vi "FPGA Beam Scanning V1.vi"(1 "Detectors":T1, 2 "Image Acquisition Parameters":T2={"Scan Type"=enum."Sample Scanning", "Scan Mode"=enum."XY", "Fast Axis Frequency (Hz)"=100.0, "Image Format"=128, "Line Accumulations"=1, "Frames Per Capture"=1, "Frames Accumulations"=1, "Image Dimension (um)"=[], "Number of Z Steps"=1, "Z Steps Size (um)"=1.0, "Pixel Size (nm)"=[]} {"Z Steps Size (um)" min=0.0; "Number of Z Steps" min=1; "Frames Accumulations" min=1; "Frames Per Capture" min=1; "Line Accumulations" min=1; "Image Format" items=["64 x 64"=64, "128 x 128"=128, "256 x 256"=256, "512 x 512"=512, "1024 x 1024"=1024, "2048 x 2048"=2048]}) -> ()   [LabVIEW 2014]
uses:
  Type Defs/Image Acquisition Parameters.ctl
  Detectors.ctl
  <vilib>/vision/Image Controls.llb/IMAQ Image.ctl
  <vilib>/FPGAPlugInAG/PCIe-7852R/niLvFpga_Open_PCIe-7852R.vi
  <vilib>/Utility/error.llb/Error Cluster From Error Code.vi
  <vilib>/rvi/errors/niLvFpgaAdjustHostInterfaceError.vi
  <vilib>/rvi/interface/common/niFpgaWaitOnOcc.vi
  <vilib>/FPGAPlugInAG/PCIe-7852R/niLvFpga_Run_PCIe-7852R.vi
  <vilib>/FPGAPlugInAG/PCIe-7852R/niLvFpga_Close_PCIe-7852R.vi
  <vilib>/rvi/interface/nirviOpenFPGA/nirviOpenFPGA.xnode
  FPGA Bitfiles/MainSTEDFPGAProj_FPGATarget2_BeamScanningCamb_cWDGwb0YZ5k.lvbitx
  FPGA Target VIs/FPGA-7852R/Beam Scanning Cambridge V1.vi
  <vilib>/rvi/interface/nirviReadWriteControl/nirviReadWriteControl.xnode
  <vilib>/rvi/interface/nirviMethod/nirviMethod.xnode
  <vilib>/rvi/interface/nirviCloseFPGA/nirviCloseFPGA.xnode
  <vilib>/rvi/errors/niLvFpgaMergeErrorWithErrorCode.vi
  <vilib>/vision/NI_Vision_Development_Module.lvlib
  NiFpgaLv.dll
  <vilib>/FPGAPlugInAG/PCIe-7852R/niLvFpga_ReadFifo_PCIe-7852R.vi
  <vilib>/FPGAPlugInAG/PCIe-7852R/niLvFpga_ConfigureFifo_PCIe-7852R.vi
  <vilib>/FPGAPlugInAG/PCIe-7852R/niLvFpga_StartFifo_PCIe-7852R.vi
panel:
  # "XY"
  # "Z"
  # "Length"
  # "Height"
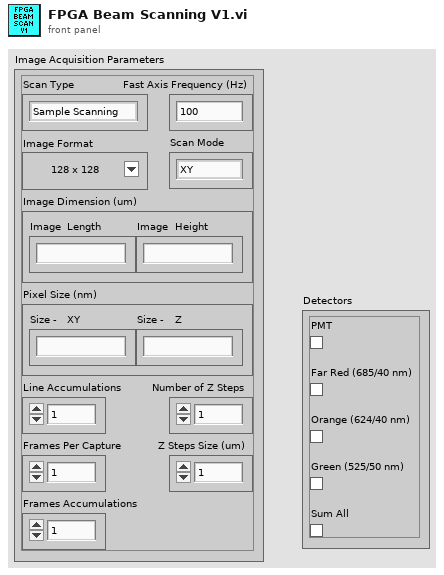
[diagram p1: front panel]
types:
  T1 = typedef "Detectors.ctl" = cluster{"PMT":bool, "Far Red (685/40 nm)":bool, "Orange (624/40 nm)":bool, "Green (525/50 nm)":bool, "Sum All":bool}
  T2 = typedef "Image Acquisition Parameters.ctl" = cluster{"Scan Type":enum16{"Sample Scanning", "Beam Scanning"}, "Scan Mode":enum16{"XY", "XZ", "YZ", "XYZ"}, "Fast Axis Frequency (Hz)":dbl, "Image Format":u16, "Line Accumulations":u16, "Frames Per Capture":u16, "Frames Accumulations":u16, "Image Dimension (um)":dbl[], "Number of Z Steps":u8, "Z Steps Size (um)":dbl, "Pixel Size (nm)":dbl[]}
  T3 = typedef "IMAQ Image.ctl" = refnum<image>
  T4 = enum16{"big-endian, network order", "native, host order", "little-endian"}
  T5 = cluster{"FPGA Sampling Period (ns)":dbl, "Counting Period (us)":dbl, "Samples Per Counting Period":i32, "Start Time (us)":dbl, "Stop Time (us)":dbl, "Normalized Scan End Position":dbl, "Normalized Scan Start Position":dbl}
  T6 = typedef "Scan Parameters.ctl" = cluster{"Fast_Ax_Amp_V":dbl, "Fast_Ax_Off_V":dbl, "Slow_Ax_Amp_V":dbl, "Slow_Ax_Off_V ":dbl, "Slow_Ax_Max_V_VperS":dbl, "Slow_Ax1_Del25ns":i32, "Slow_Ax2_Del25ns":i32, "Stage_X_Off_V":dbl, "Stage_Y_Off_V":dbl, "Stage_Z_Off_V":dbl, "Galvo1_Off_V":dbl, "Galvo2_Off_V":dbl, "Last_Scan_Mode":enum16{"XY", "XZ", "YZ", "XYZ"}, "Current_Scan_Mode":enum16{"XY", "XZ", "YZ", "XYZ"}, "Fly_Back_Lines":u16, "Linear_Ramp_End":u32, "Z_Step_I16":i16, "Z_Start_I16":i16, "Laser_States _U32":u32, "590_Voltage_I16":i16, "775_AOM_Volt_I16":i16, "Blanking OFF":bool, "Unused_Axis_I16":i16}
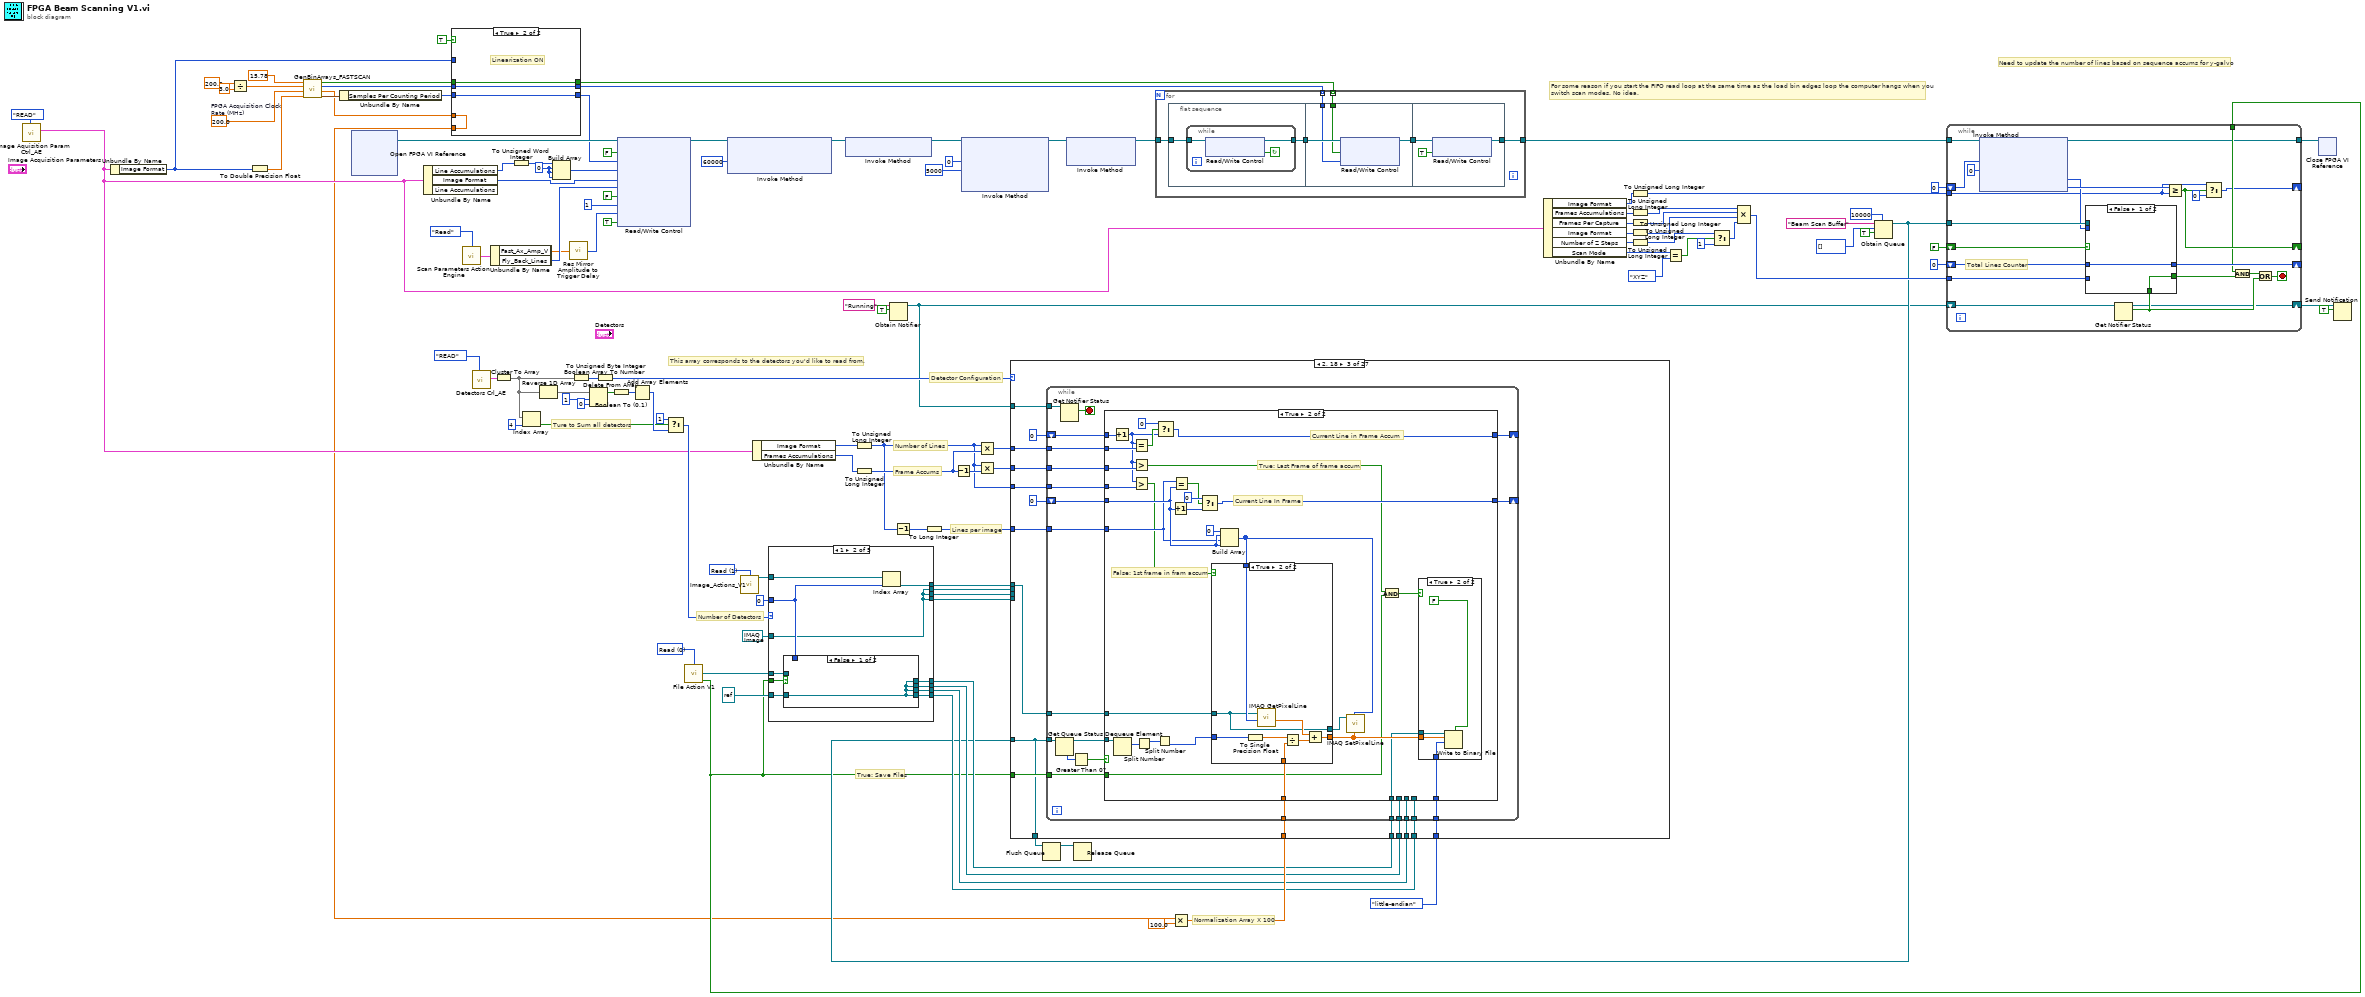
[diagram p0: block diagram]
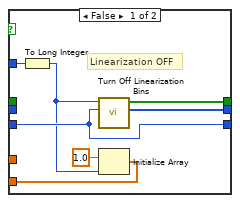
[diagram p2: hidden frame]
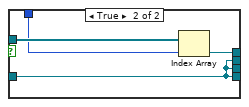
[diagram p4: hidden frame]
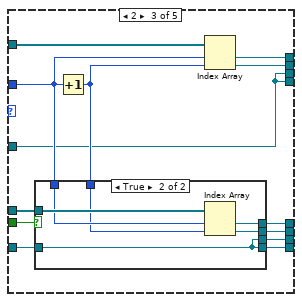
[diagram p5: hidden frame]
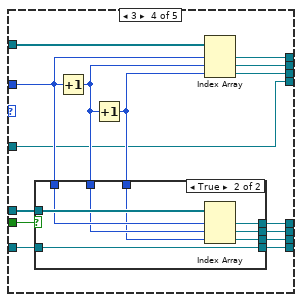
[diagram p7: hidden frame]
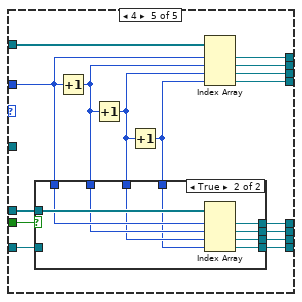
[diagram p9: hidden frame]
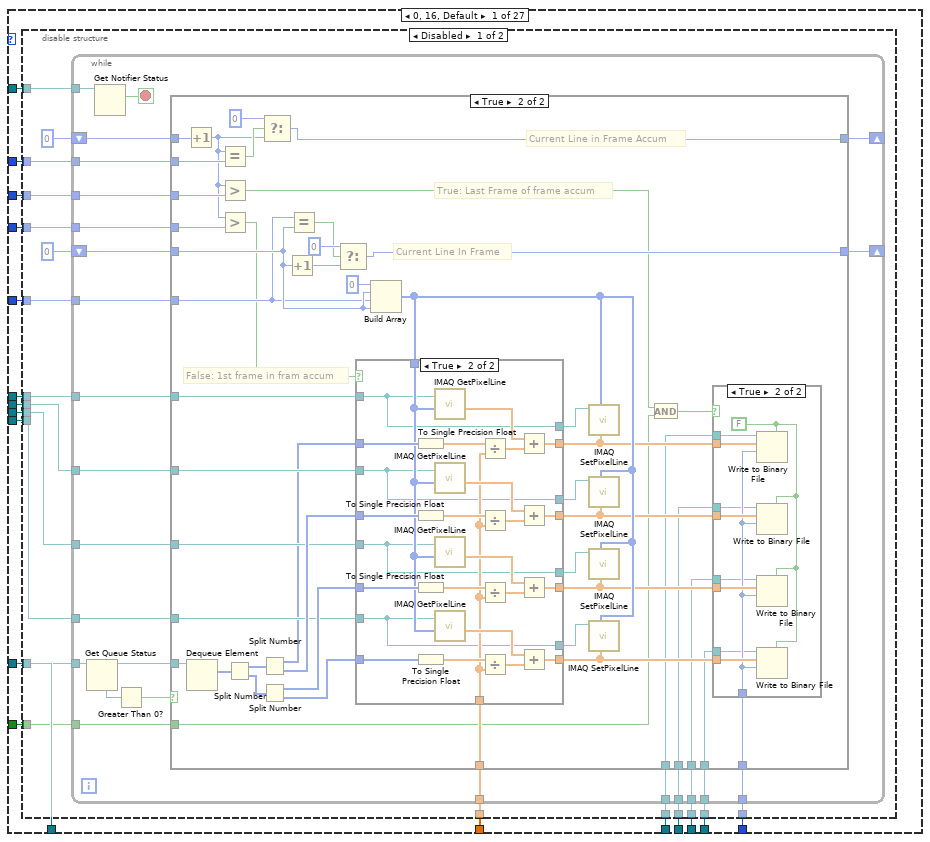
[diagram p11: hidden frame]
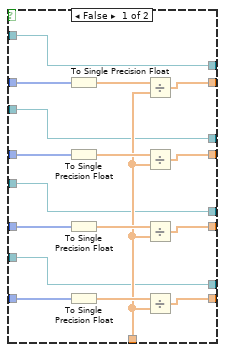
[diagram p14: hidden frame]
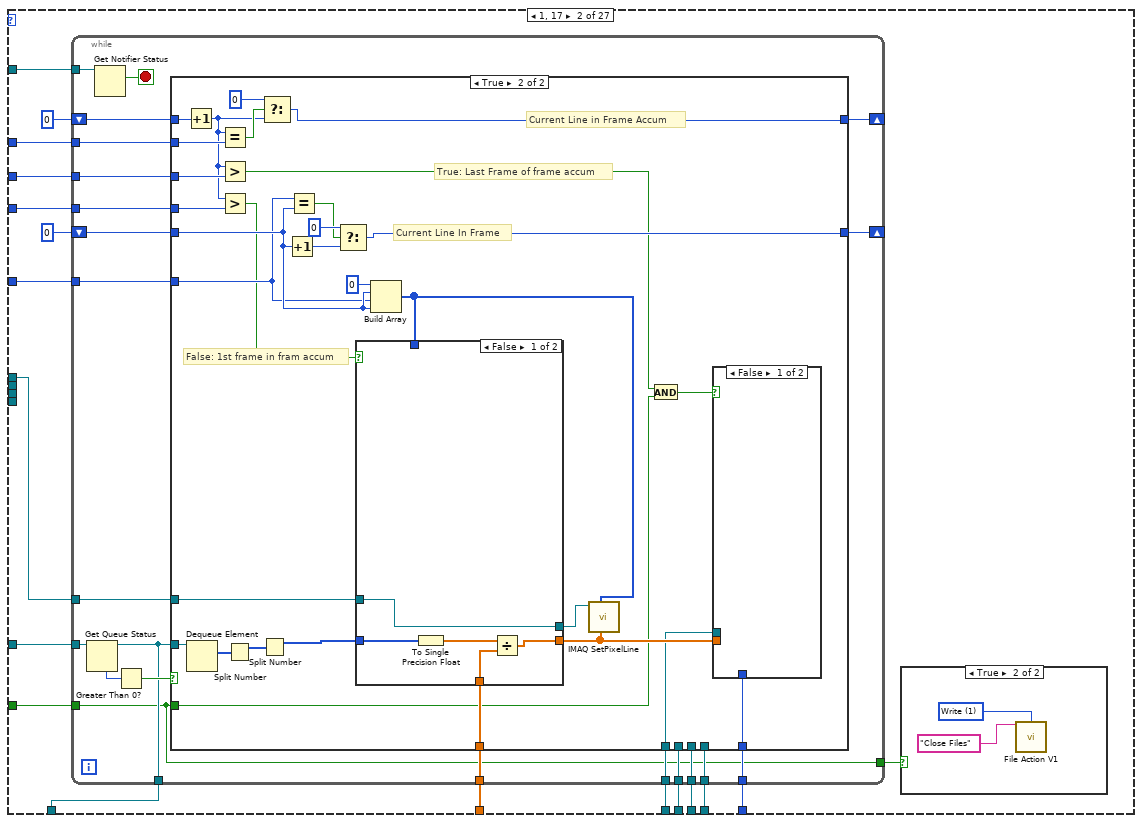
[diagram p16: hidden frame]
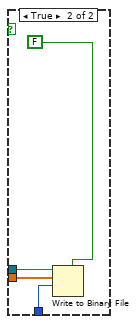
[diagram p19: hidden frame]
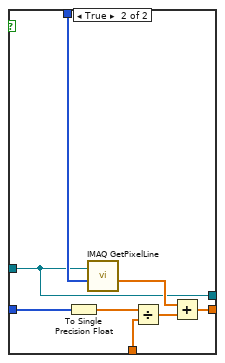
[diagram p20: hidden frame]
diagram:
  w26 = u16 0 items=["Read", "Write"] ("Mode")
  w27 = u16 0 ("element")
  w68 = u16 1 items=["Write", "Read"] ("Mode")
  w114 = 200.0  # FPGA Acquisition Clock Rate (MHz)
  # "Normalization Array X 100"
  # "This array corresponds to the detectors you'd like to read from."
  # "Ture to Sum all detectors"
  # "Number of Detectors"
  # "Detector Configuration"
  # "Frame Accums"
  # "Number of Lines"
  # "True: Save Files"
  # "Lines per image"
  # "For some reason if you start the FIFO read loop at the same time as the load bin edges loop the computer hangs when you\nswitch scan modes. No idea."
  # "Need to update the number of lines based on sequence accums for y-galvo"
  n1 = call "Image Aquisition Param Ctrl_AE.vi"("Action"=enum16{"READ", "WRITE"}."READ") -> ("Image Acquisition Parameters Out"=w15:T2)  [unwired: 10 in]
  n2 = Unbundle By Name(w15) -> ("Image Format"=w6:u16)
  n3 = Divide(x=200.0, y=3.0) -> (x/y=w111:dbl)
  n4 = To Double Precision Float(number=w6) -> (double precision float=w96:dbl)
  n5 = call "GenBinArrays_FASTSCAN.vi"("Pixels Per Line"=w96, "FPGA Acquisition Clock Rate (MHz)"=w114, "Collection Percent (%)"=w111, "Scan Rate (kHz)"=15.78) -> ("Reported Parameters"=w13:T5, "Normalization Array"=w5:sgl[], "Pre Binned Counts (x100)"=w10:u32[], "FPGA Bin Edges"=w12:bool[])
  n6 = Unbundle By Name(w13) -> ("Samples Per Counting Period"=w8:i32)
  n7 = xnode "Open FPGA VI Reference"() -> ("FPGA VI Reference Out"=w118:refnum<k20>)  [unwired: 2 in, 1 out]
  n8 = Unbundle By Name(w15) -> ("Line Accumulations"=w37:u16, "Image Format"=w34:u16)  [unwired: 1 out]
  n9 = case shown="True" TRUE {
    tunnel: w12 -> [_ w129]
    tunnel: [w125 w129] -> w11
    tunnel: w10 -> [_ w128]
    tunnel: [w124 w128] -> w9
    tunnel: w8 -> [w123 w127]
    tunnel: [w123 w127] -> w7
    tunnel: w6 -> [w122 _]
    tunnel: w5 -> [_ w126]
    tunnel: [w119 w126] -> w4
    frame False {
      # "Linearization OFF"
      n10 = To Long Integer(number=w122) -> (32bit integer=w120:i32)
      n11 = call "Turn Off Linearization Bins.vi"("Number of Samples"=w123, "Number of Pixels"=w120) -> ("Pre Binned Values"=w124:u32[], "Equal Edges Array"=w125:bool[])  [unwired: 8 in]
      n12 = Initialize Array(sgl 1.0 ("element"), w120) -> (w119:sgl[])
    }
    frame True {
      # "Linearization ON"
    }
  }
  n13 = call "Scan Parameters Action Engine.vi"("Action"=enum16{"Read", "Write"}."Read") -> ("Scan Parameters OUT"=w32:T6)  [unwired: 14 in]
  n14 = call "Detectors Crl_AE.vi"("Action"=enum16{"READ", "WRITE"}."READ") -> ("Detectors Parameters Out"=w16:T1)  [unwired: 10 in]
  n15 = Unbundle By Name(w32) -> ("Fast_Ax_Amp_V"=w24:dbl, "Fly_Back_Lines"=w31:u16)
  n16 = Cluster To Array(cluster=w16) -> (array=w21:bool[])
  n17 = To Unsigned Word Integer(number=w37) -> (unsigned 16bit integer=w36:u16)
  n18 = Index Array(array=w21, index=4) -> (element=w19:bool)
  n19 = Reverse 1D Array(array=w21) -> (reversed array=w51:bool[])
  n20 = Build Array(w36, w27, w27, w27) -> (w35:u16[])
  n21 = call "Res Mirror Amplitude to Trigger Delay.vi"("Amplitude (V)"=w24) -> ("Trigger Delay (Ticks)"=w1:u16)
  n22 = Boolean Array To Number(Boolean array=w21) -> (number=w23:u32)
  n23 = Delete From Array(array=w51, length=1, index=0) -> (array with subset deleted=w55:bool[])  [unwired: 1 out]
  n24 = To Unsigned Byte Integer(number=w23) -> (unsigned 8bit integer=w22:u8)
  n25 = Boolean To (0,1)(Boolean=w55) -> (0, 1=w54:i16[])
  n26 = xnode "Read/Write Control"("FPGA VI Reference In"=w118, "Ready For Write"=FALSE, "FPGA Samples"=w7, "Accums Per Line"=w35, "Lines Per Image"=w34, "Dead Lines"=w31, "Line Trigger"=FALSE, "Sequences"=u8 1, "Trigger Delay (Ticks)"=w1, "Stop Acquisition"=TRUE) -> ("FPGA VI Reference Out"=w117:refnum<k20>)  [unwired: 1 in, 1 out]
  n27 = Add Array Elements(numeric array=w54) -> (sum=w53:i16)
  n28 = Select(t=i16 1, s=w19, f=w53) -> (s? t:f=w48:i16)
  n29 = call "File Action V1.vi"("Mode"=w26) -> ("File REFs"=w65:refnum<file>[], "Files Open"=w25:bool)  [unwired: 12 in, 1 out]
  n30 = xnode "Invoke Method"("FPGA VI Reference In"=w117, "Requested Depth"=u32 60000) -> ("FPGA VI Reference Out"=w94:refnum<k20>)  [unwired: 1 in, 2 out]
  n31 = call "Image_Actions_V1.vi"("Mode"=w68) -> ("Image REFs OUT"=w67:T3[])  [unwired: 13 in, 1 out]
  n32 = Unbundle By Name(w15) -> ("Image Format"=w87:u16, "Frames Accumulations"=w86:u16)
  n33 = case shown="1" w48 {
    tunnel: [w131 w132 w148 w168 w207] -> w60
    tunnel: [w131 w132 w148 w182 w206] -> w61
    tunnel: [w131 w132 w160 w181 w205] -> w62
    tunnel: [w131 w142 w159 w180 w204] -> w63
    tunnel: 0 ("Offset") -> [_ w138 w155 w176 w200]
    tunnel: w67 -> [_ w141 w158 w179 w203]
    tunnel: T3 refnum ("New Image") -> [w131 w132 w148 w168 _]
    tunnel: w65 -> [_ w139 w156 w177 w201]
    tunnel: w25 -> [_ w140 w157 w178 w202]
    tunnel: [w130 w137 w153 w173 w196] -> w59
    tunnel: [w130 w136 w152 w172 w195] -> w58
    tunnel: [w130 w135 w151 w171 w194] -> w57
    tunnel: [w130 w134 w150 w170 w193] -> w56
    tunnel: refnum<file> refnum ("element") -> [w130 w133 w149 w169 w192]
    frame 0, Default {
    }
    frame 1 {
      n34 = case shown="False" w140 {
        tunnel: w139 -> [_ w147]
        tunnel: w138 -> [_ w146]
        tunnel: [w143 w145] -> w137
        tunnel: [w143 w144] -> w136
        tunnel: [w143 w144] -> w135
        tunnel: [w143 w144] -> w134
        tunnel: w133 -> [w143 w144]
        frame False {
        }
        frame True {
          n35 = Index Array(array=w147, index=w146) -> (element=w145:refnum<file>)
        }
      }
      n36 = Index Array(array=w141, index=w138) -> (element=w142:T3)
    }
    frame 2 {
      n37 = Increment(x=w155) -> (x+1=w154:i32)
      n38 = case shown="True" w157 {
        tunnel: w156 -> [_ w167]
        tunnel: w155 -> [_ w166]
        tunnel: w154 -> [_ w165]
        tunnel: [w161 w164] -> w153
        tunnel: [w161 w163] -> w152
        tunnel: [w161 w162] -> w151
        tunnel: [w161 w162] -> w150
        tunnel: w149 -> [w161 w162]
        frame False {
        }
        frame True {
          n39 = Index Array(array=w167, index #1=w166, index #2=w165) -> (element #1=w164:refnum<file>, element #2=w163:refnum<file>)
        }
      }
      n40 = Index Array(array=w158, index #1=w155, index #2=w154) -> (element #1=w159:T3, element #2=w160:T3)
    }
    frame 3 {
      n41 = Increment(x=w176) -> (x+1=w175:i32)
      n42 = Increment(x=w175) -> (x+1=w174:i32)
      n43 = case shown="True" w178 {
        tunnel: w177 -> [_ w191]
        tunnel: w176 -> [_ w190]
        tunnel: w175 -> [_ w189]
        tunnel: w174 -> [_ w188]
        tunnel: [w183 w187] -> w173
        tunnel: [w183 w186] -> w172
        tunnel: [w183 w185] -> w171
        tunnel: [w183 w184] -> w170
        tunnel: w169 -> [w183 w184]
        frame False {
        }
        frame True {
          n44 = Index Array(array=w191, index #1=w190, index #2=w189, index #3=w188) -> (element #1=w187:refnum<file>, element #2=w186:refnum<file>, element #3=w185:refnum<file>)
        }
      }
      n45 = Index Array(array=w179, index #1=w176, index #2=w175, index #3=w174) -> (element #1=w180:T3, element #2=w181:T3, element #3=w182:T3)
    }
    frame 4 {
      n46 = Increment(x=w200) -> (x+1=w199:i32)
      n47 = Increment(x=w199) -> (x+1=w198:i32)
      n48 = Increment(x=w198) -> (x+1=w197:i32)
      n49 = case shown="True" w202 {
        tunnel: w201 -> [_ w217]
        tunnel: w200 -> [_ w216]
        tunnel: w199 -> [_ w215]
        tunnel: w198 -> [_ w214]
        tunnel: w197 -> [_ w213]
        tunnel: [w208 w212] -> w196
        tunnel: [w208 w211] -> w195
        tunnel: [w208 w210] -> w194
        tunnel: [w208 w209] -> w193
        tunnel: w192 -> [w208 _]
        frame False {
        }
        frame True {
          n50 = Index Array(array=w217, index #1=w216, index #2=w215, index #3=w214, index #4=w213) -> (element #1=w212:refnum<file>, element #2=w211:refnum<file>, element #3=w210:refnum<file>, element #4=w209:refnum<file>)
        }
      }
      n51 = Index Array(array=w203, index #1=w200, index #2=w199, index #3=w198, index #4=w197) -> (element #1=w204:T3, element #2=w205:T3, element #3=w206:T3, element #4=w207:T3)
    }
  }
  n52 = xnode "Invoke Method"("FPGA VI Reference In"=w94) -> ("FPGA VI Reference Out"=w95:refnum<k20>)  [unwired: 1 in, 1 out]
  n53 = To Unsigned Long Integer(number=w87) -> (unsigned 32bit integer=w71:u32)
  n54 = To Unsigned Long Integer(number=w86) -> (unsigned 32bit integer=w72:u32)
  n55 = Obtain Notifier(name (unnamed)="Running", notification data type=TRUE) -> (notifier out=w14:refnum<notifier>)  [unwired: 2 in, 2 out]
  n56 = Decrement(x=w71) -> (x-1=w69:u32)
  n57 = To Long Integer(number=w69) -> (32bit integer=w77:i32)
  n58 = Decrement(x=w72) -> (x-1=w75:u32)
  n59 = xnode "Invoke Method"("FPGA VI Reference In"=w95, "Number of Elements"=u32 0, "Timeout (ms)"=5000) -> ("FPGA VI Reference Out"=w116:refnum<k20>)  [unwired: 1 in, 3 out]
  n60 = Multiply(x=w71, y=w72) -> (x*y=w73:u32)
  n61 = Multiply(x=w71, y=w75) -> (x*y=w74:u32)
  n62 = xnode "Invoke Method"("FPGA VI Reference In"=w116) -> ("FPGA VI Reference Out"=w110:refnum<k20>)  [unwired: 2 in, 1 out]
  n63 = for {
    tunnel: [w221] -> w83
    tunnel: w110 -> [w220]
    tunnel: w11 -> [w219] mode=indexing
    tunnel: w9 -> [w218] mode=indexing
    n64 = flat-sequence {
      tunnel: [w225] -> w223
      tunnel: w220 -> [w224]
      tunnel: w223 -> [w232]
      tunnel: [w231] -> w222
      tunnel: w219 -> [w230]
      tunnel: w218 -> [w229]
      tunnel: w222 -> [w235]
      tunnel: [w234] -> w221
      frame #0 {
        n65 = while {
          tunnel: [w228] -> w225
          tunnel: w224 -> [w227]
          stop <- w226 continue-if-true
          n66 = xnode "Read/Write Control"("FPGA VI Reference In"=w227) -> ("FPGA VI Reference Out"=w228:refnum<k20>, "Ready For Write"=w226:bool)  [unwired: 1 in, 1 out]
        }
      }
      frame #1 {
        n67 = xnode "Read/Write Control"("FPGA VI Reference In"=w232, "BinEdge"=w230, "PreBinnedValue"=w229) -> ("FPGA VI Reference Out"=w231:refnum<k20>)  [unwired: 1 in, 1 out]
      }
      frame #2 {
        n68 = xnode "Read/Write Control"("FPGA VI Reference In"=w235, "Ready For Write"=TRUE) -> ("FPGA VI Reference Out"=w234:refnum<k20>)  [unwired: 1 in, 1 out]
      }
    }
  }
  n69 = Multiply(x=w4, y=sgl 100.0) -> (x*y=w85:sgl[])
  n70 = Unbundle By Name(w15) -> ("Image Format"=w102:u16, "Frames Accumulations"=w45:u16, "Frames Per Capture"=w103:u16, "Image Format"=w46:u16, "Number of Z Steps"=w42:u8, "Scan Mode"=w43:enum16{"XY", "XZ", "YZ", "XYZ"})
  n71 = To Unsigned Long Integer(number=w102) -> (unsigned 32bit integer=w109:u32)
  n72 = To Unsigned Long Integer(number=w45) -> (unsigned 32bit integer=w41:u32)
  n73 = To Unsigned Long Integer(number=w103) -> (unsigned 32bit integer=w40:u32)
  n74 = To Unsigned Long Integer(number=w46) -> (unsigned 32bit integer=w39:u32)
  n75 = To Unsigned Long Integer(number=w42) -> (unsigned 32bit integer=w38:u32)
  n76 = Equal?(x=w43, y=enum16{"XY", "XZ", "YZ", "XYZ"}."XYZ") -> (x = y?=w90:bool)
  n77 = Select(t=w38, s=w90, f=u32 1) -> (s? t:f=w89:u32)
  n78 = Compound Arithmetic op=MULTIPLY(w41, w40, w39, w89) -> (w104:u32)
  n79 = Obtain Queue(max queue size (-1, unlimited)=10000, name (unnamed)="Beam Scan Buffer", element data type=u64[] [], create if not found? (T)=TRUE) -> (queue out=w29:refnum<queue>)  [unwired: 1 in, 2 out]
  n80 = case shown="2, 18" w22 {
    tunnel: w77 -> [w252 w414 w503 w592 w697 w785 w892 w1000 w1124 w1212 w1319 w1427 w1552 w1659 w1785 w1912 w2054 w2143 w2233 w2323 w2415 w2505 w2595 w2687 w2776 w2868 w2960]
    tunnel: w25 -> [w249 w411 w500 w589 w694 w782 w889 w997 w1121 w1209 w1316 w1424 w1549 w1656 w1782 w1909 w2051 w2140 w2230 w2320 w2412 w2502 w2592 w2684 w2773 w2865 w2957]
    tunnel: T4."little-endian" ("byte order (0:big-endian, network order)") -> [w251 w413 w502 w591 w696 w784 w891 w999 w1123 w1211 w1318 w1426 w1551 w1658 w1784 w1911 w2053 w2142 w2232 w2322 w2414 w2504 w2594 w2686 w2775 w2867 w2959]
    tunnel: w85 -> [w250 w412 w501 w590 w695 w783 w890 w998 w1122 w1210 w1317 w1425 w1550 w1657 w1783 w1910 w2052 w2141 w2231 w2321 w2413 w2503 w2593 w2685 w2774 w2866 w2958]
    tunnel: w74 -> [w248 w409 w498 w587 w692 w780 w887 w995 w1119 w1207 w1314 w1422 w1547 w1654 w1780 w1907 w2049 w2138 w2228 w2318 w2410 w2500 w2590 w2682 w2771 w2863 w2955]
    tunnel: w73 -> [w247 w408 w497 w586 w691 w779 w886 w994 w1118 w1206 w1313 w1421 w1546 w1653 w1779 w1906 w2048 w2137 w2227 w2317 w2409 w2499 w2589 w2681 w2770 w2862 w2954]
    tunnel: w71 -> [w246 w407 w496 w585 w690 w778 w885 w993 w1117 w1205 w1312 w1420 w1545 w1652 w1778 w1905 w2047 w2136 w2226 w2316 w2408 w2498 w2588 w2680 w2769 w2861 w2953]
    tunnel: w29 -> [w245 w406 w495 w578 w689 w777 w884 w992 w1116 w1204 w1311 w1419 w1544 w1651 w1777 w1904 w2046 w2135 w2225 w2315 w2407 w2497 w2587 w2679 w2768 w2860 w2952]
    tunnel: w63 -> [w240 w401 w490 w580 w684 w772 w879 w987 w1111 w1199 w1306 w1414 w1539 w1646 w1772 w1899 w2041 w2130 w2220 w2310 w2402 w2492 w2582 w2674 w2763 w2855 w2947]
    tunnel: w62 -> [w239 _ _ w579 _ w771 w878 w986 _ w1198 w1305 w1413 w1538 w1645 w1771 w1898 _ _ _ _ _ _ _ _ _ _ _]
    tunnel: w61 -> [w238 _ _ _ _ _ _ w985 _ _ _ w1412 _ w1644 w1770 w1897 _ _ _ _ _ _ _ _ _ _ _]
    tunnel: w60 -> [w237 _ _ _ _ _ _ _ _ _ _ _ _ _ _ w1896 _ _ _ _ _ _ _ _ _ _ _]
    tunnel: [w245 w400 w495 w577 w689 w777 w884 w992 w1116 w1204 w1311 w1419 w1544 w1651 w1777 w1904 w2046 w2135 w2225 w2315 w2407 w2497 w2587 w2679 w2768 w2860 w2952] -> w28
    tunnel: w59 -> [w244 w405 w494 w584 w688 w776 w883 w991 w1115 w1203 w1310 w1418 w1543 w1650 w1776 w1903 w2045 w2134 w2224 w2314 w2406 w2496 w2586 w2678 w2767 w2859 w2951]
    tunnel: w58 -> [w243 w404 w493 w583 w687 w775 w882 w990 w1114 w1202 w1309 w1417 w1542 w1649 w1775 w1902 w2044 w2133 w2223 w2313 w2405 w2495 w2585 w2677 w2766 w2858 w2950]
    tunnel: w57 -> [w242 w403 w492 w582 w686 w774 w881 w989 w1113 w1201 w1308 w1416 w1541 w1648 w1774 w1901 w2043 w2132 w2222 w2312 w2404 w2494 w2584 w2676 w2765 w2857 w2949]
    tunnel: w56 -> [w241 w402 w491 w581 w685 w773 w880 w988 w1112 w1200 w1307 w1415 w1540 w1647 w1773 w1900 w2042 w2131 w2221 w2311 w2403 w2493 w2583 w2675 w2764 w2856 w2948]
    tunnel: w14 -> [w236 w398 w489 w576 w683 w770 w877 w984 w1110 w1197 w1304 w1411 w1537 w1643 w1769 w1895 w2040 w2129 w2219 w2309 w2401 w2491 w2581 w2673 w2762 w2854 w2946]
    frame 0, 16, Default {
      n81 = disable-structure shown="Disabled" {
        disable-tunnel: w252 -> [w270 _]
        disable-tunnel: w251 -> [w269 _]
        disable-tunnel: w250 -> [w268 _]
        disable-tunnel: w249 -> [w267 _]
        disable-tunnel: w236 -> [w266 _]
        disable-tunnel: w248 -> [w264 _]
        disable-tunnel: w247 -> [w263 _]
        disable-tunnel: w246 -> [w262 _]
        disable-tunnel: w245 -> [w261 _]
        disable-tunnel: w244 -> [w260 _]
        disable-tunnel: w243 -> [w259 _]
        disable-tunnel: w242 -> [w258 _]
        disable-tunnel: w241 -> [w257 _]
        disable-tunnel: w240 -> [w256 _]
        disable-tunnel: w239 -> [w255 _]
        disable-tunnel: w238 -> [w254 _]
        disable-tunnel: w237 -> [w253 _]
        frame Disabled {
          n82 = while {
            shift-right: [w294] -> _
            shift-left: 0 -> [w295]
            tunnel: w270 -> [w296]
            tunnel: w269 -> [w293]
            tunnel: w268 -> [w292]
            tunnel: w267 -> [w291]
            tunnel: w266 -> [w287]
            shift-right: [w284] -> _
            shift-left: u32 0 -> [w285]
            tunnel: w264 -> [w283]
            tunnel: w263 -> [w282]
            tunnel: w262 -> [w281]
            tunnel: w261 -> [w280]
            tunnel: w256 -> [w279]
            tunnel: w255 -> [w278]
            tunnel: w254 -> [w277]
            tunnel: w253 -> [w276]
            tunnel: w260 -> [w275]
            tunnel: w259 -> [w274]
            tunnel: w258 -> [w273]
            tunnel: w257 -> [w272]
            stop <- w286 stop-if-true
            n83 = Get Queue Status(queue=w280) -> (queue out=w288:refnum<queue>, # elements in queue=w290:i32)  [unwired: 2 in, 6 out]
            n84 = Get Notifier Status(notifier=w287) -> (current notification=w286:bool)  [unwired: 1 in, 4 out]
            n85 = Greater Than 0?(x=w290) -> (x > 0?=w289:bool)
            n86 = case shown="True" w289 {
              tunnel: w296 -> [_ w333]
              tunnel: w295 -> [w298 w334]
              tunnel: [w298 w332] -> w294
              tunnel: w293 -> [_ w326]
              tunnel: w292 -> [_ w325]
              tunnel: w291 -> [_ w315]
              tunnel: w288 -> [_ w324]
              tunnel: w285 -> [w297 w321]
              tunnel: [w297 w320] -> w284
              tunnel: w283 -> [_ w319]
              tunnel: w282 -> [_ w318]
              tunnel: w281 -> [_ w313]
              tunnel: w279 -> [_ w311]
              tunnel: w278 -> [_ w310]
              tunnel: w277 -> [_ w309]
              tunnel: w276 -> [_ w308]
              tunnel: w275 -> [_ w302]
              tunnel: w274 -> [_ w301]
              tunnel: w273 -> [_ w300]
              tunnel: w272 -> [_ w299]
              frame False {
              }
              frame True {
                # "False: 1st frame in fram accum"
                # "True: Last Frame of frame accum"
                # "Current Line in Frame Accum"
                # "Current Line In Frame"
                n87 = Increment(x=w321) -> (x+1=w314:u32)
                n88 = Dequeue Element(queue=w324) -> (element=w343:u64[])  [unwired: 2 in, 3 out]
                n89 = Equal?(x=w314, y=w318) -> (x = y?=w323:bool)
                n90 = Greater?(x=w314, y=w319) -> (0:w316:bool)
                n91 = Greater?(x=w314, y=w313) -> (0:w312:bool)
                n92 = Split Number(x=w343) -> (hi(x)=w344:u32[], lo(x)=w342:u32[])
                n93 = Split Number(x=w344) -> (hi(x)=w303:u16[], lo(x)=w341:u16[])
                n94 = Split Number(x=w342) -> (hi(x)=w340:u16[], lo(x)=w339:u16[])
                n95 = Select(t=u32 0, s=w323, f=w314) -> (s? t:f=w320:u32)
                n96 = Increment(x=w334) -> (x+1=w336:i32)
                n97 = Equal?(x=w333, y=w334) -> (x = y?=w335:bool)
                n98 = Select(t=0, s=w335, f=w336) -> (s? t:f=w332:i32)
                n99 = Build Array(0, w334, w333, w334) -> (w331:i32[])
                n100 = case shown="True" w312 {
                  tunnel: w303 -> [w370 w397]
                  tunnel: w341 -> [w365 w396]
                  tunnel: w340 -> [w364 w395]
                  tunnel: w339 -> [w363 w394]
                  tunnel: [w361 w386] -> w328
                  tunnel: [w362 w385] -> w329
                  tunnel: [w369 w384] -> w330
                  tunnel: [w360 w383] -> w327
                  tunnel: w331 -> [_ w378]
                  tunnel: w325 -> [w359 w376]
                  tunnel: w311 -> [w358 w373]
                  tunnel: w310 -> [w357 w374]
                  tunnel: w309 -> [w356 w375]
                  tunnel: w308 -> [w355 w372]
                  tunnel: [w356 w375] -> w305
                  tunnel: [w357 w374] -> w306
                  tunnel: [w358 w373] -> w307
                  tunnel: [w355 w372] -> w304
                  frame False {
                    n101 = To Single Precision Float(number=w370) -> (single precision float=w371:sgl[])
                    n102 = To Single Precision Float(number=w365) -> (single precision float=w368:sgl[])
                    n103 = To Single Precision Float(number=w364) -> (single precision float=w367:sgl[])
                    n104 = To Single Precision Float(number=w363) -> (single precision float=w366:sgl[])
                    n105 = Divide(x=w371, y=w359) -> (x/y=w369:sgl[])
                    n106 = Divide(x=w368, y=w359) -> (x/y=w362:sgl[])
                    n107 = Divide(x=w367, y=w359) -> (x/y=w361:sgl[])
                    n108 = Divide(x=w366, y=w359) -> (x/y=w360:sgl[])
                  }
                  frame True {
                    n109 = To Single Precision Float(number=w397) -> (single precision float=w377:sgl[])
                    n110 = To Single Precision Float(number=w396) -> (single precision float=w393:sgl[])
                    n111 = To Single Precision Float(number=w395) -> (single precision float=w392:sgl[])
                    n112 = To Single Precision Float(number=w394) -> (single precision float=w391:sgl[])
                    n113 = call "IMAQ GetPixelLine"("Line Coordinates"=w378, "Image"=w373) -> ("Pixels Line (Float)"=w382:sgl[])  [unwired: 2 in, 4 out]
                    n114 = call "IMAQ GetPixelLine"("Line Coordinates"=w378, "Image"=w374) -> ("Pixels Line (Float)"=w381:sgl[])  [unwired: 2 in, 4 out]
                    n115 = call "IMAQ GetPixelLine"("Line Coordinates"=w378, "Image"=w375) -> ("Pixels Line (Float)"=w380:sgl[])  [unwired: 2 in, 4 out]
                    n116 = call "IMAQ GetPixelLine"("Line Coordinates"=w378, "Image"=w372) -> ("Pixels Line (Float)"=w379:sgl[])  [unwired: 2 in, 4 out]
                    n117 = Divide(x=w377, y=w376) -> (x/y=w390:sgl[])
                    n118 = Divide(x=w393, y=w376) -> (x/y=w389:sgl[])
                    n119 = Divide(x=w392, y=w376) -> (x/y=w388:sgl[])
                    n120 = Divide(x=w391, y=w376) -> (x/y=w387:sgl[])
                    n121 = Add(x=w382, y=w390) -> (x+y=w384:sgl[])
                    n122 = Add(x=w381, y=w389) -> (x+y=w385:sgl[])
                    n123 = Add(x=w380, y=w388) -> (x+y=w386:sgl[])
                    n124 = Add(x=w379, y=w387) -> (x+y=w383:sgl[])
                  }
                }
                n125 = call "IMAQ SetPixelLine"("Pixels Line (Float)"=w330, "Line Coordinates"=w331, "Image"=w307) -> ()  [unwired: 7 in, 2 out]
                n126 = call "IMAQ SetPixelLine"("Pixels Line (Float)"=w329, "Line Coordinates"=w331, "Image"=w306) -> ()  [unwired: 7 in, 2 out]
                n127 = call "IMAQ SetPixelLine"("Pixels Line (Float)"=w328, "Line Coordinates"=w331, "Image"=w305) -> ()  [unwired: 7 in, 2 out]
                n128 = call "IMAQ SetPixelLine"("Pixels Line (Float)"=w327, "Line Coordinates"=w331, "Image"=w304) -> ()  [unwired: 7 in, 2 out]
                n129 = And(x=w316, y=w315) -> (x .and. y?=w317:bool)
                n130 = case shown="True" w317 {
                  tunnel: w330 -> [_ w354]
                  tunnel: w329 -> [_ w353]
                  tunnel: w328 -> [_ w352]
                  tunnel: w327 -> [_ w351]
                  tunnel: w326 -> [_ w349]
                  tunnel: w302 -> [_ w348]
                  tunnel: w301 -> [_ w347]
                  tunnel: w300 -> [_ w346]
                  tunnel: w299 -> [_ w345]
                  frame False {
                  }
                  frame True {
                    w350 = FALSE ("prepend array or string size? (T)")
                    n131 = Write to Binary File(file (use dialog)=w348, data=w354, 5:w350, 9:w349) -> ()  [unwired: 2 in, 3 out]
                    n132 = Write to Binary File(file (use dialog)=w347, data=w353, 5:w350, 9:w349) -> ()  [unwired: 2 in, 3 out]
                    n133 = Write to Binary File(file (use dialog)=w346, data=w352, 5:w350, 9:w349) -> ()  [unwired: 2 in, 3 out]
                    n134 = Write to Binary File(file (use dialog)=w345, data=w351, 5:w350, 9:w349) -> ()  [unwired: 2 in, 3 out]
                  }
                }
              }
            }
          }
        }
        frame Enabled {
        }
      }
    }
    frame 1, 17 {
      n135 = while {
        shift-right: [w437] -> _
        shift-left: 0 -> [w438]
        tunnel: w414 -> [w439]
        tunnel: w413 -> [w436]
        tunnel: w412 -> [w435]
        tunnel: w411 -> [w418]
        tunnel: w398 -> [w432]
        shift-right: [w429] -> _
        shift-left: u32 0 -> [w430]
        tunnel: w409 -> [w428]
        tunnel: w408 -> [w427]
        tunnel: w407 -> [w426]
        tunnel: w406 -> [w425]
        tunnel: w401 -> [w424]
        tunnel: w405 -> [w423]
        tunnel: w404 -> [w422]
        tunnel: w403 -> [w421]
        tunnel: w402 -> [w420]
        tunnel: [w419] -> w400
        tunnel: [w418] -> w399
        stop <- w431 stop-if-true
        n136 = Get Queue Status(queue=w425) -> (queue out=w419:refnum<queue>, # elements in queue=w434:i32)  [unwired: 2 in, 6 out]
        n137 = Get Notifier Status(notifier=w432) -> (current notification=w431:bool)  [unwired: 1 in, 4 out]
        n138 = Greater Than 0?(x=w434) -> (x > 0?=w433:bool)
        n139 = case shown="True" w433 {
          tunnel: w439 -> [_ w466]
          tunnel: w438 -> [w441 w467]
          tunnel: [w441 w465] -> w437
          tunnel: w436 -> [_ w462]
          tunnel: w435 -> [_ w461]
          tunnel: w418 -> [_ w444]
          tunnel: w419 -> [_ w460]
          tunnel: w430 -> [w440 w457]
          tunnel: [w440 w456] -> w429
          tunnel: w428 -> [_ w455]
          tunnel: w427 -> [_ w454]
          tunnel: w426 -> [_ w450]
          tunnel: w424 -> [_ w448]
          tunnel: w423 -> [_ w446]
          tunnel: w422 -> [_ _]
          tunnel: w421 -> [_ _]
          tunnel: w420 -> [_ _]
          frame False {
          }
          frame True {
            # "False: 1st frame in fram accum"
            # "True: Last Frame of frame accum"
            # "Current Line in Frame Accum"
            # "Current Line In Frame"
            n140 = Increment(x=w457) -> (x+1=w451:u32)
            n141 = Dequeue Element(queue=w460) -> (element=w470:u64[])  [unwired: 2 in, 3 out]
            n142 = Equal?(x=w451, y=w454) -> (x = y?=w459:bool)
            n143 = Greater?(x=w451, y=w455) -> (0:w452:bool)
            n144 = Greater?(x=w451, y=w450) -> (0:w449:bool)
            n145 = Split Number(x=w470) -> (hi(x)=w471:u32[])  [unwired: 1 out]
            n146 = Split Number(x=w471) -> (hi(x)=w445:u16[])  [unwired: 1 out]
            n147 = Select(t=u32 0, s=w459, f=w451) -> (s? t:f=w456:u32)
            n148 = Increment(x=w467) -> (x+1=w443:i32)
            n149 = Equal?(x=w466, y=w467) -> (x = y?=w468:bool)
            n150 = Select(t=0, s=w468, f=w443) -> (s? t:f=w465:i32)
            n151 = Build Array(0, w467, w466, w467) -> (w464:i32[])
            n152 = case shown="False" w449 {
              tunnel: w445 -> [w479 w488]
              tunnel: [w478 w485] -> w463
              tunnel: w464 -> [_ w483]
              tunnel: w461 -> [w477 w482]
              tunnel: w448 -> [w476 w481]
              tunnel: [w476 w481] -> w447
              frame False {
                n153 = To Single Precision Float(number=w479) -> (single precision float=w480:sgl[])
                n154 = Divide(x=w480, y=w477) -> (x/y=w478:sgl[])
              }
              frame True {
                n155 = To Single Precision Float(number=w488) -> (single precision float=w487:sgl[])
                n156 = call "IMAQ GetPixelLine"("Line Coordinates"=w483, "Image"=w481) -> ("Pixels Line (Float)"=w484:sgl[])  [unwired: 2 in, 4 out]
                n157 = Divide(x=w487, y=w482) -> (x/y=w486:sgl[])
                n158 = Add(x=w484, y=w486) -> (x+y=w485:sgl[])
              }
            }
            n159 = call "IMAQ SetPixelLine"("Pixels Line (Float)"=w463, "Line Coordinates"=w464, "Image"=w447) -> ()  [unwired: 7 in, 2 out]
            n160 = And(x=w452, y=w444) -> (x .and. y?=w453:bool)
            n161 = case shown="False" w453 {
              tunnel: w463 -> [_ w475]
              tunnel: w462 -> [_ w473]
              tunnel: w446 -> [_ w472]
              frame False {
              }
              frame True {
                n162 = Write to Binary File(file (use dialog)=w472, data=w475, 5:FALSE ("prepend array or string size? (T)"), 9:w473) -> ()  [unwired: 2 in, 3 out]
              }
            }
          }
        }
      }
      n163 = case shown="True" w399 {
        frame False {
        }
        frame True {
          w417 = u16 1 items=["Read", "Write"] ("Mode")
          n164 = call "File Action V1.vi"("Action"="Close Files", "Mode"=w417) -> ()  [unwired: 11 in, 3 out]
        }
      }
    }
    frame 2, 18 {
      n165 = while {
        shift-right: [w524] -> _
        shift-left: 0 -> [w525]
        tunnel: w503 -> [w526]
        tunnel: w502 -> [w523]
        tunnel: w501 -> [w522]
        tunnel: w500 -> [w521]
        tunnel: w489 -> [w517]
        shift-right: [w514] -> _
        shift-left: u32 0 -> [w515]
        tunnel: w498 -> [w513]
        tunnel: w497 -> [w512]
        tunnel: w496 -> [w511]
        tunnel: w495 -> [w510]
        tunnel: w490 -> [w509]
        tunnel: w494 -> [w508]
        tunnel: w493 -> [w507]
        tunnel: w492 -> [w506]
        tunnel: w491 -> [w505]
        stop <- w516 stop-if-true
        n166 = Get Queue Status(queue=w510) -> (queue out=w518:refnum<queue>, # elements in queue=w520:i32)  [unwired: 2 in, 6 out]
        n167 = Get Notifier Status(notifier=w517) -> (current notification=w516:bool)  [unwired: 1 in, 4 out]
        n168 = Greater Than 0?(x=w520) -> (x > 0?=w519:bool)
        n169 = case shown="True" w519 {
          tunnel: w526 -> [_ w552]
          tunnel: w525 -> [w528 w553]
          tunnel: [w528 w551] -> w524
          tunnel: w523 -> [_ w548]
          tunnel: w522 -> [_ w547]
          tunnel: w521 -> [_ w537]
          tunnel: w518 -> [_ w546]
          tunnel: w515 -> [w527 w543]
          tunnel: [w527 w542] -> w514
          tunnel: w513 -> [_ w541]
          tunnel: w512 -> [_ w540]
          tunnel: w511 -> [_ w535]
          tunnel: w509 -> [_ w533]
          tunnel: w508 -> [_ w531]
          tunnel: w507 -> [_ _]
          tunnel: w506 -> [_ _]
          tunnel: w505 -> [_ _]
          frame False {
          }
          frame True {
            # "False: 1st frame in fram accum"
            # "True: Last Frame of frame accum"
            # "Current Line in Frame Accum"
            # "Current Line In Frame"
            n170 = Increment(x=w543) -> (x+1=w536:u32)
            n171 = Dequeue Element(queue=w546) -> (element=w557:u64[])  [unwired: 2 in, 3 out]
            n172 = Equal?(x=w536, y=w540) -> (x = y?=w545:bool)
            n173 = Greater?(x=w536, y=w541) -> (0:w538:bool)
            n174 = Greater?(x=w536, y=w535) -> (0:w534:bool)
            n175 = Split Number(x=w557) -> (hi(x)=w558:u32[])  [unwired: 1 out]
            n176 = Split Number(x=w558) -> (lo(x)=w530:u16[])  [unwired: 1 out]
            n177 = Select(t=u32 0, s=w545, f=w536) -> (s? t:f=w542:u32)
            n178 = Increment(x=w553) -> (x+1=w555:i32)
            n179 = Equal?(x=w552, y=w553) -> (x = y?=w554:bool)
            n180 = Select(t=0, s=w554, f=w555) -> (s? t:f=w551:i32)
            n181 = Build Array(0, w553, w552, w553) -> (w550:i32[])
            n182 = case shown="True" w534 {
              tunnel: w530 -> [w566 w575]
              tunnel: [w565 w572] -> w549
              tunnel: w550 -> [_ w570]
              tunnel: w547 -> [w564 w569]
              tunnel: w533 -> [w563 w568]
              tunnel: [w563 w568] -> w532
              frame False {
                n183 = To Single Precision Float(number=w566) -> (single precision float=w567:sgl[])
                n184 = Divide(x=w567, y=w564) -> (x/y=w565:sgl[])
              }
              frame True {
                n185 = To Single Precision Float(number=w575) -> (single precision float=w574:sgl[])
                n186 = call "IMAQ GetPixelLine"("Line Coordinates"=w570, "Image"=w568) -> ("Pixels Line (Float)"=w571:sgl[])  [unwired: 2 in, 4 out]
                n187 = Divide(x=w574, y=w569) -> (x/y=w573:sgl[])
                n188 = Add(x=w571, y=w573) -> (x+y=w572:sgl[])
              }
            }
            n189 = call "IMAQ SetPixelLine"("Pixels Line (Float)"=w549, "Line Coordinates"=w550, "Image"=w532) -> ()  [unwired: 7 in, 2 out]
            n190 = And(x=w538, y=w537) -> (x .and. y?=w539:bool)
            n191 = case shown="True" w539 {
              tunnel: w549 -> [_ w562]
              tunnel: w548 -> [_ w560]
              tunnel: w531 -> [_ w559]
              frame False {
              }
              frame True {
                n192 = Write to Binary File(file (use dialog)=w559, data=w562, 5:FALSE ("prepend array or string size? (T)"), 9:w560) -> ()  [unwired: 2 in, 3 out]
              }
            }
          }
        }
      }
    }
    frame 3 {
      n193 = while {
        shift-right: [w614] -> _
        shift-left: 0 -> [w615]
        tunnel: w592 -> [w616]
        tunnel: w591 -> [w613]
        tunnel: w590 -> [w612]
        tunnel: w589 -> [w611]
        tunnel: w576 -> [w608]
        shift-right: [w605] -> _
        shift-left: u32 0 -> [w606]
        tunnel: w587 -> [w604]
        tunnel: w586 -> [w603]
        tunnel: w585 -> [w602]
        tunnel: w578 -> [w601]
        tunnel: w580 -> [w600]
        tunnel: w579 -> [w599]
        tunnel: w584 -> [w598]
        tunnel: w583 -> [w597]
        tunnel: w582 -> [w596]
        tunnel: w581 -> [w595]
        tunnel: [w594] -> w577
        stop <- w607 stop-if-true
        n194 = Get Queue Status(queue=w601) -> (queue out=w594:refnum<queue>, # elements in queue=w610:i32)  [unwired: 2 in, 6 out]
        n195 = Get Notifier Status(notifier=w608) -> (current notification=w607:bool)  [unwired: 1 in, 4 out]
        n196 = Greater Than 0?(x=w610) -> (x > 0?=w609:bool)
        n197 = case shown="True" w609 {
          tunnel: w616 -> [_ w646]
          tunnel: w615 -> [w618 w647]
          tunnel: [w618 w645] -> w614
          tunnel: w613 -> [_ w641]
          tunnel: w612 -> [_ w640]
          tunnel: w611 -> [_ w630]
          tunnel: w594 -> [_ w639]
          tunnel: w606 -> [w617 w636]
          tunnel: [w617 w635] -> w605
          tunnel: w604 -> [_ w634]
          tunnel: w603 -> [_ w633]
          tunnel: w602 -> [_ w628]
          tunnel: w600 -> [_ w626]
          tunnel: w599 -> [_ w625]
          tunnel: w598 -> [_ w622]
          tunnel: w597 -> [_ w621]
          tunnel: w596 -> [_ _]
          tunnel: w595 -> [_ _]
          frame False {
          }
          frame True {
            # "False: 1st frame in fram accum"
            # "True: Last Frame of frame accum"
            # "Current Line in Frame Accum"
            # "Current Line In Frame"
            n198 = Increment(x=w636) -> (x+1=w629:u32)
            n199 = Dequeue Element(queue=w639) -> (element=w652:u64[])  [unwired: 2 in, 3 out]
            n200 = Equal?(x=w629, y=w633) -> (x = y?=w638:bool)
            n201 = Greater?(x=w629, y=w634) -> (0:w631:bool)
            n202 = Greater?(x=w629, y=w628) -> (0:w627:bool)
            n203 = Split Number(x=w652) -> (hi(x)=w653:u32[])  [unwired: 1 out]
            n204 = Split Number(x=w653) -> (hi(x)=w620:u16[], lo(x)=w619:u16[])
            n205 = Select(t=u32 0, s=w638, f=w629) -> (s? t:f=w635:u32)
            n206 = Increment(x=w647) -> (x+1=w649:i32)
            n207 = Equal?(x=w646, y=w647) -> (x = y?=w648:bool)
            n208 = Select(t=0, s=w648, f=w649) -> (s? t:f=w645:i32)
            n209 = Build Array(0, w647, w646, w647) -> (w644:i32[])
            n210 = case shown="True" w627 {
              tunnel: w620 -> [w666 w682]
              tunnel: w619 -> [w665 w681]
              tunnel: [w663 w676] -> w642
              tunnel: [w664 w675] -> w643
              tunnel: w644 -> [_ w672]
              tunnel: w640 -> [w662 w671]
              tunnel: w626 -> [w661 w669]
              tunnel: w625 -> [w660 w670]
              tunnel: [w660 w670] -> w623
              tunnel: [w661 w669] -> w624
              frame False {
                n211 = To Single Precision Float(number=w666) -> (single precision float=w668:sgl[])
                n212 = To Single Precision Float(number=w665) -> (single precision float=w667:sgl[])
                n213 = Divide(x=w668, y=w662) -> (x/y=w664:sgl[])
                n214 = Divide(x=w667, y=w662) -> (x/y=w663:sgl[])
              }
              frame True {
                n215 = To Single Precision Float(number=w682) -> (single precision float=w680:sgl[])
                n216 = To Single Precision Float(number=w681) -> (single precision float=w679:sgl[])
                n217 = call "IMAQ GetPixelLine"("Line Coordinates"=w672, "Image"=w669) -> ("Pixels Line (Float)"=w674:sgl[])  [unwired: 2 in, 4 out]
                n218 = call "IMAQ GetPixelLine"("Line Coordinates"=w672, "Image"=w670) -> ("Pixels Line (Float)"=w673:sgl[])  [unwired: 2 in, 4 out]
                n219 = Divide(x=w680, y=w671) -> (x/y=w678:sgl[])
                n220 = Divide(x=w679, y=w671) -> (x/y=w677:sgl[])
                n221 = Add(x=w674, y=w678) -> (x+y=w675:sgl[])
                n222 = Add(x=w673, y=w677) -> (x+y=w676:sgl[])
              }
            }
            n223 = call "IMAQ SetPixelLine"("Pixels Line (Float)"=w643, "Line Coordinates"=w644, "Image"=w624) -> ()  [unwired: 7 in, 2 out]
            n224 = call "IMAQ SetPixelLine"("Pixels Line (Float)"=w642, "Line Coordinates"=w644, "Image"=w623) -> ()  [unwired: 7 in, 2 out]
            n225 = And(x=w631, y=w630) -> (x .and. y?=w632:bool)
            n226 = case shown="False" w632 {
              tunnel: w643 -> [_ w659]
              tunnel: w642 -> [_ w658]
              tunnel: w641 -> [_ w656]
              tunnel: w622 -> [_ w655]
              tunnel: w621 -> [_ w654]
              frame False {
              }
              frame True {
                w657 = FALSE ("prepend array or string size? (T)")
                n227 = Write to Binary File(file (use dialog)=w655, data=w659, 5:w657, 9:w656) -> ()  [unwired: 2 in, 3 out]
                n228 = Write to Binary File(file (use dialog)=w654, data=w658, 5:w657, 9:w656) -> ()  [unwired: 2 in, 3 out]
              }
            }
          }
        }
      }
    }
    frame 4, 20 {
      n229 = while {
        shift-right: [w718] -> _
        shift-left: 0 -> [w719]
        tunnel: w697 -> [w720]
        tunnel: w696 -> [w717]
        tunnel: w695 -> [w716]
        tunnel: w694 -> [w715]
        tunnel: w683 -> [w711]
        shift-right: [w708] -> _
        shift-left: u32 0 -> [w709]
        tunnel: w692 -> [w707]
        tunnel: w691 -> [w706]
        tunnel: w690 -> [w705]
        tunnel: w689 -> [w704]
        tunnel: w684 -> [w703]
        tunnel: w688 -> [w702]
        tunnel: w687 -> [w701]
        tunnel: w686 -> [w700]
        tunnel: w685 -> [w699]
        stop <- w710 stop-if-true
        n230 = Get Queue Status(queue=w704) -> (queue out=w712:refnum<queue>, # elements in queue=w714:i32)  [unwired: 2 in, 6 out]
        n231 = Get Notifier Status(notifier=w711) -> (current notification=w710:bool)  [unwired: 1 in, 4 out]
        n232 = Greater Than 0?(x=w714) -> (x > 0?=w713:bool)
        n233 = case shown="True" w713 {
          tunnel: w720 -> [_ w745]
          tunnel: w719 -> [w722 w746]
          tunnel: [w722 w744] -> w718
          tunnel: w717 -> [_ w741]
          tunnel: w716 -> [_ w740]
          tunnel: w715 -> [_ w730]
          tunnel: w712 -> [_ w739]
          tunnel: w709 -> [w721 w736]
          tunnel: [w721 w735] -> w708
          tunnel: w707 -> [_ w734]
          tunnel: w706 -> [_ w733]
          tunnel: w705 -> [_ w728]
          tunnel: w703 -> [_ w726]
          tunnel: w702 -> [_ w724]
          tunnel: w701 -> [_ _]
          tunnel: w700 -> [_ _]
          tunnel: w699 -> [_ _]
          frame False {
          }
          frame True {
            # "False: 1st frame in fram accum"
            # "True: Last Frame of frame accum"
            # "Current Line in Frame Accum"
            # "Current Line In Frame"
            n234 = Increment(x=w736) -> (x+1=w729:u32)
            n235 = Dequeue Element(queue=w739) -> (element=w752:u64[])  [unwired: 2 in, 3 out]
            n236 = Equal?(x=w729, y=w733) -> (x = y?=w738:bool)
            n237 = Greater?(x=w729, y=w734) -> (0:w731:bool)
            n238 = Greater?(x=w729, y=w728) -> (0:w727:bool)
            n239 = Split Number(x=w752) -> (lo(x)=w751:u32[])  [unwired: 1 out]
            n240 = Split Number(x=w751) -> (hi(x)=w723:u16[])  [unwired: 1 out]
            n241 = Select(t=u32 0, s=w738, f=w729) -> (s? t:f=w735:u32)
            n242 = Increment(x=w746) -> (x+1=w748:i32)
            n243 = Equal?(x=w745, y=w746) -> (x = y?=w747:bool)
            n244 = Select(t=0, s=w747, f=w748) -> (s? t:f=w744:i32)
            n245 = Build Array(0, w746, w745, w746) -> (w743:i32[])
            n246 = case shown="True" w727 {
              tunnel: w723 -> [w760 w769]
              tunnel: [w759 w766] -> w742
              tunnel: w743 -> [_ w764]
              tunnel: w740 -> [w758 w763]
              tunnel: w726 -> [w757 w762]
              tunnel: [w757 w762] -> w725
              frame False {
                n247 = To Single Precision Float(number=w760) -> (single precision float=w761:sgl[])
                n248 = Divide(x=w761, y=w758) -> (x/y=w759:sgl[])
              }
              frame True {
                n249 = To Single Precision Float(number=w769) -> (single precision float=w768:sgl[])
                n250 = call "IMAQ GetPixelLine"("Line Coordinates"=w764, "Image"=w762) -> ("Pixels Line (Float)"=w765:sgl[])  [unwired: 2 in, 4 out]
                n251 = Divide(x=w768, y=w763) -> (x/y=w767:sgl[])
                n252 = Add(x=w765, y=w767) -> (x+y=w766:sgl[])
              }
            }
            n253 = call "IMAQ SetPixelLine"("Pixels Line (Float)"=w742, "Line Coordinates"=w743, "Image"=w725) -> ()  [unwired: 7 in, 2 out]
            n254 = And(x=w731, y=w730) -> (x .and. y?=w732:bool)
            n255 = case shown="True" w732 {
              tunnel: w742 -> [_ w756]
              tunnel: w741 -> [_ w754]
              tunnel: w724 -> [_ w753]
              frame False {
              }
              frame True {
                n256 = Write to Binary File(file (use dialog)=w753, data=w756, 5:FALSE ("prepend array or string size? (T)"), 9:w754) -> ()  [unwired: 2 in, 3 out]
              }
            }
          }
        }
      }
    }
    frame 5 {
      n257 = while {
        shift-right: [w807] -> _
        shift-left: 0 -> [w808]
        tunnel: w785 -> [w809]
        tunnel: w784 -> [w806]
        tunnel: w783 -> [w805]
        tunnel: w782 -> [w804]
        tunnel: w770 -> [w800]
        shift-right: [w797] -> _
        shift-left: u32 0 -> [w798]
        tunnel: w780 -> [w796]
        tunnel: w779 -> [w795]
        tunnel: w778 -> [w794]
        tunnel: w777 -> [w793]
        tunnel: w772 -> [w792]
        tunnel: w771 -> [w791]
        tunnel: w776 -> [w790]
        tunnel: w775 -> [w789]
        tunnel: w774 -> [w788]
        tunnel: w773 -> [w787]
        stop <- w799 stop-if-true
        n258 = Get Queue Status(queue=w793) -> (queue out=w801:refnum<queue>, # elements in queue=w803:i32)  [unwired: 2 in, 6 out]
        n259 = Get Notifier Status(notifier=w800) -> (current notification=w799:bool)  [unwired: 1 in, 4 out]
        n260 = Greater Than 0?(x=w803) -> (x > 0?=w802:bool)
        n261 = case shown="True" w802 {
          tunnel: w809 -> [_ w838]
          tunnel: w808 -> [w811 w839]
          tunnel: [w811 w837] -> w807
          tunnel: w806 -> [_ w833]
          tunnel: w805 -> [_ w832]
          tunnel: w804 -> [_ w822]
          tunnel: w801 -> [_ w831]
          tunnel: w798 -> [w810 w828]
          tunnel: [w810 w827] -> w797
          tunnel: w796 -> [_ w826]
          tunnel: w795 -> [_ w825]
          tunnel: w794 -> [_ w820]
          tunnel: w792 -> [_ w818]
          tunnel: w791 -> [_ w817]
          tunnel: w790 -> [_ w813]
          tunnel: w789 -> [_ w812]
          tunnel: w788 -> [_ _]
          tunnel: w787 -> [_ _]
          frame False {
          }
          frame True {
            # "False: 1st frame in fram accum"
            # "True: Last Frame of frame accum"
            # "Current Line in Frame Accum"
            # "Current Line In Frame"
            n262 = Increment(x=w828) -> (x+1=w821:u32)
            n263 = Dequeue Element(queue=w831) -> (element=w846:u64[])  [unwired: 2 in, 3 out]
            n264 = Equal?(x=w821, y=w825) -> (x = y?=w830:bool)
            n265 = Greater?(x=w821, y=w826) -> (0:w823:bool)
            n266 = Greater?(x=w821, y=w820) -> (0:w819:bool)
            n267 = Split Number(x=w846) -> (hi(x)=w847:u32[], lo(x)=w845:u32[])
            n268 = Split Number(x=w847) -> (hi(x)=w814:u16[])  [unwired: 1 out]
            n269 = Split Number(x=w845) -> (hi(x)=w844:u16[])  [unwired: 1 out]
            n270 = Select(t=u32 0, s=w830, f=w821) -> (s? t:f=w827:u32)
            n271 = Increment(x=w839) -> (x+1=w841:i32)
            n272 = Equal?(x=w838, y=w839) -> (x = y?=w840:bool)
            n273 = Select(t=0, s=w840, f=w841) -> (s? t:f=w837:i32)
            n274 = Build Array(0, w839, w838, w839) -> (w836:i32[])
            n275 = case shown="False" w819 {
              tunnel: w814 -> [w861 w876]
              tunnel: w844 -> [w858 w875]
              tunnel: [w857 w871] -> w834
              tunnel: [w860 w870] -> w835
              tunnel: w836 -> [_ w867]
              tunnel: w832 -> [w856 w865]
              tunnel: w818 -> [w855 w863]
              tunnel: w817 -> [w854 w864]
              tunnel: [w854 w864] -> w815
              tunnel: [w855 w863] -> w816
              frame False {
                n276 = To Single Precision Float(number=w861) -> (single precision float=w862:sgl[])
                n277 = To Single Precision Float(number=w858) -> (single precision float=w859:sgl[])
                n278 = Divide(x=w862, y=w856) -> (x/y=w860:sgl[])
                n279 = Divide(x=w859, y=w856) -> (x/y=w857:sgl[])
              }
              frame True {
                n280 = To Single Precision Float(number=w876) -> (single precision float=w866:sgl[])
                n281 = To Single Precision Float(number=w875) -> (single precision float=w874:sgl[])
                n282 = call "IMAQ GetPixelLine"("Line Coordinates"=w867, "Image"=w863) -> ("Pixels Line (Float)"=w869:sgl[])  [unwired: 2 in, 4 out]
                n283 = call "IMAQ GetPixelLine"("Line Coordinates"=w867, "Image"=w864) -> ("Pixels Line (Float)"=w868:sgl[])  [unwired: 2 in, 4 out]
                n284 = Divide(x=w866, y=w865) -> (x/y=w873:sgl[])
                n285 = Divide(x=w874, y=w865) -> (x/y=w872:sgl[])
                n286 = Add(x=w869, y=w873) -> (x+y=w870:sgl[])
                n287 = Add(x=w868, y=w872) -> (x+y=w871:sgl[])
              }
            }
            n288 = call "IMAQ SetPixelLine"("Pixels Line (Float)"=w835, "Line Coordinates"=w836, "Image"=w816) -> ()  [unwired: 7 in, 2 out]
            n289 = call "IMAQ SetPixelLine"("Pixels Line (Float)"=w834, "Line Coordinates"=w836, "Image"=w815) -> ()  [unwired: 7 in, 2 out]
            n290 = And(x=w823, y=w822) -> (x .and. y?=w824:bool)
            n291 = case shown="True" w824 {
              tunnel: w835 -> [_ w853]
              tunnel: w834 -> [_ w852]
              tunnel: w833 -> [_ w850]
              tunnel: w813 -> [_ w849]
              tunnel: w812 -> [_ w848]
              frame False {
              }
              frame True {
                w851 = FALSE ("prepend array or string size? (T)")
                n292 = Write to Binary File(file (use dialog)=w849, data=w853, 5:w851, 9:w850) -> ()  [unwired: 2 in, 3 out]
                n293 = Write to Binary File(file (use dialog)=w848, data=w852, 5:w851, 9:w850) -> ()  [unwired: 2 in, 3 out]
              }
            }
          }
        }
      }
    }
    frame 6 {
      n294 = while {
        shift-right: [w914] -> _
        shift-left: 0 -> [w915]
        tunnel: w892 -> [w916]
        tunnel: w891 -> [w913]
        tunnel: w890 -> [w912]
        tunnel: w889 -> [w911]
        tunnel: w877 -> [w907]
        shift-right: [w904] -> _
        shift-left: u32 0 -> [w905]
        tunnel: w887 -> [w903]
        tunnel: w886 -> [w902]
        tunnel: w885 -> [w901]
        tunnel: w884 -> [w900]
        tunnel: w879 -> [w899]
        tunnel: w878 -> [w898]
        tunnel: w883 -> [w897]
        tunnel: w882 -> [w896]
        tunnel: w881 -> [w895]
        tunnel: w880 -> [w894]
        stop <- w906 stop-if-true
        n295 = Get Queue Status(queue=w900) -> (queue out=w908:refnum<queue>, # elements in queue=w910:i32)  [unwired: 2 in, 6 out]
        n296 = Get Notifier Status(notifier=w907) -> (current notification=w906:bool)  [unwired: 1 in, 4 out]
        n297 = Greater Than 0?(x=w910) -> (x > 0?=w909:bool)
        n298 = case shown="False" w909 {
          tunnel: w916 -> [_ w944]
          tunnel: w915 -> [w918 w945]
          tunnel: [w918 w943] -> w914
          tunnel: w913 -> [_ w939]
          tunnel: w912 -> [_ w938]
          tunnel: w911 -> [_ w928]
          tunnel: w908 -> [_ w937]
          tunnel: w905 -> [w917 w934]
          tunnel: [w917 w933] -> w904
          tunnel: w903 -> [_ w932]
          tunnel: w902 -> [_ w931]
          tunnel: w901 -> [_ w926]
          tunnel: w899 -> [_ w924]
          tunnel: w898 -> [_ w923]
          tunnel: w897 -> [_ w920]
          tunnel: w896 -> [_ w919]
          tunnel: w895 -> [_ _]
          tunnel: w894 -> [_ _]
          frame False {
          }
          frame True {
            # "False: 1st frame in fram accum"
            # "True: Last Frame of frame accum"
            # "Current Line in Frame Accum"
            # "Current Line In Frame"
            n299 = Increment(x=w934) -> (x+1=w927:u32)
            n300 = Dequeue Element(queue=w937) -> (element=w953:u64[])  [unwired: 2 in, 3 out]
            n301 = Equal?(x=w927, y=w931) -> (x = y?=w936:bool)
            n302 = Greater?(x=w927, y=w932) -> (0:w929:bool)
            n303 = Greater?(x=w927, y=w926) -> (0:w925:bool)
            n304 = Split Number(x=w953) -> (hi(x)=w954:u32[], lo(x)=w952:u32[])
            n305 = Split Number(x=w954) -> (lo(x)=w951:u16[])  [unwired: 1 out]
            n306 = Split Number(x=w952) -> (hi(x)=w950:u16[])  [unwired: 1 out]
            n307 = Select(t=u32 0, s=w936, f=w927) -> (s? t:f=w933:u32)
            n308 = Increment(x=w945) -> (x+1=w947:i32)
            n309 = Equal?(x=w944, y=w945) -> (x = y?=w946:bool)
            n310 = Select(t=0, s=w946, f=w947) -> (s? t:f=w943:i32)
            n311 = Build Array(0, w945, w944, w945) -> (w942:i32[])
            n312 = case shown="False" w925 {
              tunnel: w951 -> [w967 w983]
              tunnel: w950 -> [w966 w982]
              tunnel: [w964 w977] -> w940
              tunnel: [w965 w976] -> w941
              tunnel: w942 -> [_ w973]
              tunnel: w938 -> [w963 w972]
              tunnel: w924 -> [w962 w970]
              tunnel: w923 -> [w961 w971]
              tunnel: [w961 w971] -> w921
              tunnel: [w962 w970] -> w922
              frame False {
                n313 = To Single Precision Float(number=w967) -> (single precision float=w969:sgl[])
                n314 = To Single Precision Float(number=w966) -> (single precision float=w968:sgl[])
                n315 = Divide(x=w969, y=w963) -> (x/y=w965:sgl[])
                n316 = Divide(x=w968, y=w963) -> (x/y=w964:sgl[])
              }
              frame True {
                n317 = To Single Precision Float(number=w983) -> (single precision float=w981:sgl[])
                n318 = To Single Precision Float(number=w982) -> (single precision float=w980:sgl[])
                n319 = call "IMAQ GetPixelLine"("Line Coordinates"=w973, "Image"=w970) -> ("Pixels Line (Float)"=w975:sgl[])  [unwired: 2 in, 4 out]
                n320 = call "IMAQ GetPixelLine"("Line Coordinates"=w973, "Image"=w971) -> ("Pixels Line (Float)"=w974:sgl[])  [unwired: 2 in, 4 out]
                n321 = Divide(x=w981, y=w972) -> (x/y=w979:sgl[])
                n322 = Divide(x=w980, y=w972) -> (x/y=w978:sgl[])
                n323 = Add(x=w975, y=w979) -> (x+y=w976:sgl[])
                n324 = Add(x=w974, y=w978) -> (x+y=w977:sgl[])
              }
            }
            n325 = call "IMAQ SetPixelLine"("Pixels Line (Float)"=w941, "Line Coordinates"=w942, "Image"=w922) -> ()  [unwired: 7 in, 2 out]
            n326 = call "IMAQ SetPixelLine"("Pixels Line (Float)"=w940, "Line Coordinates"=w942, "Image"=w921) -> ()  [unwired: 7 in, 2 out]
            n327 = And(x=w929, y=w928) -> (x .and. y?=w930:bool)
            n328 = case shown="True" w930 {
              tunnel: w941 -> [_ w960]
              tunnel: w940 -> [_ w959]
              tunnel: w939 -> [_ w957]
              tunnel: w920 -> [_ w956]
              tunnel: w919 -> [_ w955]
              frame False {
              }
              frame True {
                w958 = FALSE ("prepend array or string size? (T)")
                n329 = Write to Binary File(file (use dialog)=w956, data=w960, 5:w958, 9:w957) -> ()  [unwired: 2 in, 3 out]
                n330 = Write to Binary File(file (use dialog)=w955, data=w959, 5:w958, 9:w957) -> ()  [unwired: 2 in, 3 out]
              }
            }
          }
        }
      }
    }
    frame 7 {
      n331 = while {
        shift-right: [w1023] -> _
        shift-left: 0 -> [w1024]
        tunnel: w1000 -> [w1025]
        tunnel: w999 -> [w1022]
        tunnel: w998 -> [w1021]
        tunnel: w997 -> [w1020]
        tunnel: w984 -> [w1016]
        shift-right: [w1013] -> _
        shift-left: u32 0 -> [w1014]
        tunnel: w995 -> [w1012]
        tunnel: w994 -> [w1011]
        tunnel: w993 -> [w1010]
        tunnel: w992 -> [w1009]
        tunnel: w987 -> [w1008]
        tunnel: w986 -> [w1007]
        tunnel: w985 -> [w1006]
        tunnel: w991 -> [w1005]
        tunnel: w990 -> [w1004]
        tunnel: w989 -> [w1003]
        tunnel: w988 -> [w1002]
        stop <- w1015 stop-if-true
        n332 = Get Queue Status(queue=w1009) -> (queue out=w1017:refnum<queue>, # elements in queue=w1019:i32)  [unwired: 2 in, 6 out]
        n333 = Get Notifier Status(notifier=w1016) -> (current notification=w1015:bool)  [unwired: 1 in, 4 out]
        n334 = Greater Than 0?(x=w1019) -> (x > 0?=w1018:bool)
        n335 = case shown="True" w1018 {
          tunnel: w1025 -> [_ w1058]
          tunnel: w1024 -> [w1027 w1059]
          tunnel: [w1027 w1057] -> w1023
          tunnel: w1022 -> [_ w1052]
          tunnel: w1021 -> [_ w1051]
          tunnel: w1020 -> [_ w1041]
          tunnel: w1017 -> [_ w1050]
          tunnel: w1014 -> [w1026 w1047]
          tunnel: [w1026 w1046] -> w1013
          tunnel: w1012 -> [_ w1045]
          tunnel: w1011 -> [_ w1044]
          tunnel: w1010 -> [_ w1039]
          tunnel: w1008 -> [_ w1037]
          tunnel: w1007 -> [_ w1036]
          tunnel: w1006 -> [_ w1035]
          tunnel: w1005 -> [_ w1030]
          tunnel: w1004 -> [_ w1029]
          tunnel: w1003 -> [_ w1028]
          tunnel: w1002 -> [_ _]
          frame False {
          }
          frame True {
            # "False: 1st frame in fram accum"
            # "True: Last Frame of frame accum"
            # "Current Line in Frame Accum"
            # "Current Line In Frame"
            n336 = Increment(x=w1047) -> (x+1=w1040:u32)
            n337 = Dequeue Element(queue=w1050) -> (element=w1067:u64[])  [unwired: 2 in, 3 out]
            n338 = Equal?(x=w1040, y=w1044) -> (x = y?=w1049:bool)
            n339 = Greater?(x=w1040, y=w1045) -> (0:w1042:bool)
            n340 = Greater?(x=w1040, y=w1039) -> (0:w1038:bool)
            n341 = Split Number(x=w1067) -> (hi(x)=w1068:u32[], lo(x)=w1066:u32[])
            n342 = Split Number(x=w1068) -> (hi(x)=w1031:u16[], lo(x)=w1065:u16[])
            n343 = Split Number(x=w1066) -> (hi(x)=w1064:u16[])  [unwired: 1 out]
            n344 = Select(t=u32 0, s=w1049, f=w1040) -> (s? t:f=w1046:u32)
            n345 = Increment(x=w1059) -> (x+1=w1061:i32)
            n346 = Equal?(x=w1058, y=w1059) -> (x = y?=w1060:bool)
            n347 = Select(t=0, s=w1060, f=w1061) -> (s? t:f=w1057:i32)
            n348 = Build Array(0, w1059, w1058, w1059) -> (w1056:i32[])
            n349 = case shown="False" w1038 {
              tunnel: w1031 -> [w1088 w1109]
              tunnel: w1065 -> [w1084 w1108]
              tunnel: w1064 -> [w1083 w1107]
              tunnel: [w1081 w1101] -> w1053
              tunnel: [w1082 w1100] -> w1054
              tunnel: [w1087 w1099] -> w1055
              tunnel: w1056 -> [_ w1095]
              tunnel: w1051 -> [w1080 w1093]
              tunnel: w1037 -> [w1079 w1090]
              tunnel: w1036 -> [w1078 w1091]
              tunnel: w1035 -> [w1077 w1092]
              tunnel: [w1077 w1092] -> w1032
              tunnel: [w1078 w1091] -> w1033
              tunnel: [w1079 w1090] -> w1034
              frame False {
                n350 = To Single Precision Float(number=w1088) -> (single precision float=w1089:sgl[])
                n351 = To Single Precision Float(number=w1084) -> (single precision float=w1086:sgl[])
                n352 = To Single Precision Float(number=w1083) -> (single precision float=w1085:sgl[])
                n353 = Divide(x=w1089, y=w1080) -> (x/y=w1087:sgl[])
                n354 = Divide(x=w1086, y=w1080) -> (x/y=w1082:sgl[])
                n355 = Divide(x=w1085, y=w1080) -> (x/y=w1081:sgl[])
              }
              frame True {
                n356 = To Single Precision Float(number=w1109) -> (single precision float=w1094:sgl[])
                n357 = To Single Precision Float(number=w1108) -> (single precision float=w1106:sgl[])
                n358 = To Single Precision Float(number=w1107) -> (single precision float=w1105:sgl[])
                n359 = call "IMAQ GetPixelLine"("Line Coordinates"=w1095, "Image"=w1090) -> ("Pixels Line (Float)"=w1098:sgl[])  [unwired: 2 in, 4 out]
                n360 = call "IMAQ GetPixelLine"("Line Coordinates"=w1095, "Image"=w1091) -> ("Pixels Line (Float)"=w1097:sgl[])  [unwired: 2 in, 4 out]
                n361 = call "IMAQ GetPixelLine"("Line Coordinates"=w1095, "Image"=w1092) -> ("Pixels Line (Float)"=w1096:sgl[])  [unwired: 2 in, 4 out]
                n362 = Divide(x=w1094, y=w1093) -> (x/y=w1104:sgl[])
                n363 = Divide(x=w1106, y=w1093) -> (x/y=w1103:sgl[])
                n364 = Divide(x=w1105, y=w1093) -> (x/y=w1102:sgl[])
                n365 = Add(x=w1098, y=w1104) -> (x+y=w1099:sgl[])
                n366 = Add(x=w1097, y=w1103) -> (x+y=w1100:sgl[])
                n367 = Add(x=w1096, y=w1102) -> (x+y=w1101:sgl[])
              }
            }
            n368 = call "IMAQ SetPixelLine"("Pixels Line (Float)"=w1055, "Line Coordinates"=w1056, "Image"=w1034) -> ()  [unwired: 7 in, 2 out]
            n369 = call "IMAQ SetPixelLine"("Pixels Line (Float)"=w1054, "Line Coordinates"=w1056, "Image"=w1033) -> ()  [unwired: 7 in, 2 out]
            n370 = call "IMAQ SetPixelLine"("Pixels Line (Float)"=w1053, "Line Coordinates"=w1056, "Image"=w1032) -> ()  [unwired: 7 in, 2 out]
            n371 = And(x=w1042, y=w1041) -> (x .and. y?=w1043:bool)
            n372 = case shown="True" w1043 {
              tunnel: w1055 -> [_ w1076]
              tunnel: w1054 -> [_ w1075]
              tunnel: w1053 -> [_ w1074]
              tunnel: w1052 -> [_ w1072]
              tunnel: w1030 -> [_ w1071]
              tunnel: w1029 -> [_ w1070]
              tunnel: w1028 -> [_ w1069]
              frame False {
              }
              frame True {
                w1073 = FALSE ("prepend array or string size? (T)")
                n373 = Write to Binary File(file (use dialog)=w1071, data=w1076, 5:w1073, 9:w1072) -> ()  [unwired: 2 in, 3 out]
                n374 = Write to Binary File(file (use dialog)=w1070, data=w1075, 5:w1073, 9:w1072) -> ()  [unwired: 2 in, 3 out]
                n375 = Write to Binary File(file (use dialog)=w1069, data=w1074, 5:w1073, 9:w1072) -> ()  [unwired: 2 in, 3 out]
              }
            }
          }
        }
      }
    }
    frame 8, 24 {
      n376 = while {
        shift-right: [w1145] -> _
        shift-left: 0 -> [w1146]
        tunnel: w1124 -> [w1147]
        tunnel: w1123 -> [w1144]
        tunnel: w1122 -> [w1143]
        tunnel: w1121 -> [w1142]
        tunnel: w1110 -> [w1138]
        shift-right: [w1135] -> _
        shift-left: u32 0 -> [w1136]
        tunnel: w1119 -> [w1134]
        tunnel: w1118 -> [w1133]
        tunnel: w1117 -> [w1132]
        tunnel: w1116 -> [w1131]
        tunnel: w1111 -> [w1130]
        tunnel: w1115 -> [w1129]
        tunnel: w1114 -> [w1128]
        tunnel: w1113 -> [w1127]
        tunnel: w1112 -> [w1126]
        stop <- w1137 stop-if-true
        n377 = Get Queue Status(queue=w1131) -> (queue out=w1139:refnum<queue>, # elements in queue=w1141:i32)  [unwired: 2 in, 6 out]
        n378 = Get Notifier Status(notifier=w1138) -> (current notification=w1137:bool)  [unwired: 1 in, 4 out]
        n379 = Greater Than 0?(x=w1141) -> (x > 0?=w1140:bool)
        n380 = case shown="True" w1140 {
          tunnel: w1147 -> [_ w1171]
          tunnel: w1146 -> [w1149 w1172]
          tunnel: [w1149 w1170] -> w1145
          tunnel: w1144 -> [_ w1167]
          tunnel: w1143 -> [_ w1166]
          tunnel: w1142 -> [_ w1156]
          tunnel: w1139 -> [_ w1165]
          tunnel: w1136 -> [w1148 w1162]
          tunnel: [w1148 w1161] -> w1135
          tunnel: w1134 -> [_ w1160]
          tunnel: w1133 -> [_ w1159]
          tunnel: w1132 -> [_ w1154]
          tunnel: w1130 -> [_ w1152]
          tunnel: w1129 -> [_ w1150]
          tunnel: w1128 -> [_ _]
          tunnel: w1127 -> [_ _]
          tunnel: w1126 -> [_ _]
          frame False {
          }
          frame True {
            # "False: 1st frame in fram accum"
            # "True: Last Frame of frame accum"
            # "Current Line in Frame Accum"
            # "Current Line In Frame"
            n381 = Increment(x=w1162) -> (x+1=w1155:u32)
            n382 = Dequeue Element(queue=w1165) -> (element=w1179:u64[])  [unwired: 2 in, 3 out]
            n383 = Equal?(x=w1155, y=w1159) -> (x = y?=w1164:bool)
            n384 = Greater?(x=w1155, y=w1160) -> (0:w1157:bool)
            n385 = Greater?(x=w1155, y=w1154) -> (0:w1153:bool)
            n386 = Split Number(x=w1179) -> (lo(x)=w1178:u32[])  [unwired: 1 out]
            n387 = Split Number(x=w1178) -> (lo(x)=w1177:u16[])  [unwired: 1 out]
            n388 = Select(t=u32 0, s=w1164, f=w1155) -> (s? t:f=w1161:u32)
            n389 = Increment(x=w1172) -> (x+1=w1174:i32)
            n390 = Equal?(x=w1171, y=w1172) -> (x = y?=w1173:bool)
            n391 = Select(t=0, s=w1173, f=w1174) -> (s? t:f=w1170:i32)
            n392 = Build Array(0, w1172, w1171, w1172) -> (w1169:i32[])
            n393 = case shown="True" w1153 {
              tunnel: w1177 -> [w1187 w1196]
              tunnel: [w1186 w1193] -> w1168
              tunnel: w1169 -> [_ w1191]
              tunnel: w1166 -> [w1185 w1190]
              tunnel: w1152 -> [w1184 w1189]
              tunnel: [w1184 w1189] -> w1151
              frame False {
                n394 = To Single Precision Float(number=w1187) -> (single precision float=w1188:sgl[])
                n395 = Divide(x=w1188, y=w1185) -> (x/y=w1186:sgl[])
              }
              frame True {
                n396 = To Single Precision Float(number=w1196) -> (single precision float=w1195:sgl[])
                n397 = call "IMAQ GetPixelLine"("Line Coordinates"=w1191, "Image"=w1189) -> ("Pixels Line (Float)"=w1192:sgl[])  [unwired: 2 in, 4 out]
                n398 = Divide(x=w1195, y=w1190) -> (x/y=w1194:sgl[])
                n399 = Add(x=w1192, y=w1194) -> (x+y=w1193:sgl[])
              }
            }
            n400 = call "IMAQ SetPixelLine"("Pixels Line (Float)"=w1168, "Line Coordinates"=w1169, "Image"=w1151) -> ()  [unwired: 7 in, 2 out]
            n401 = And(x=w1157, y=w1156) -> (x .and. y?=w1158:bool)
            n402 = case shown="True" w1158 {
              tunnel: w1168 -> [_ w1183]
              tunnel: w1167 -> [_ w1181]
              tunnel: w1150 -> [_ w1180]
              frame False {
              }
              frame True {
                n403 = Write to Binary File(file (use dialog)=w1180, data=w1183, 5:FALSE ("prepend array or string size? (T)"), 9:w1181) -> ()  [unwired: 2 in, 3 out]
              }
            }
          }
        }
      }
    }
    frame 9 {
      n404 = while {
        shift-right: [w1234] -> _
        shift-left: 0 -> [w1235]
        tunnel: w1212 -> [w1236]
        tunnel: w1211 -> [w1233]
        tunnel: w1210 -> [w1232]
        tunnel: w1209 -> [w1231]
        tunnel: w1197 -> [w1227]
        shift-right: [w1224] -> _
        shift-left: u32 0 -> [w1225]
        tunnel: w1207 -> [w1223]
        tunnel: w1206 -> [w1222]
        tunnel: w1205 -> [w1221]
        tunnel: w1204 -> [w1220]
        tunnel: w1199 -> [w1219]
        tunnel: w1198 -> [w1218]
        tunnel: w1203 -> [w1217]
        tunnel: w1202 -> [w1216]
        tunnel: w1201 -> [w1215]
        tunnel: w1200 -> [w1214]
        stop <- w1226 stop-if-true
        n405 = Get Queue Status(queue=w1220) -> (queue out=w1228:refnum<queue>, # elements in queue=w1230:i32)  [unwired: 2 in, 6 out]
        n406 = Get Notifier Status(notifier=w1227) -> (current notification=w1226:bool)  [unwired: 1 in, 4 out]
        n407 = Greater Than 0?(x=w1230) -> (x > 0?=w1229:bool)
        n408 = case shown="True" w1229 {
          tunnel: w1236 -> [_ w1265]
          tunnel: w1235 -> [w1238 w1266]
          tunnel: [w1238 w1264] -> w1234
          tunnel: w1233 -> [_ w1260]
          tunnel: w1232 -> [_ w1259]
          tunnel: w1231 -> [_ w1249]
          tunnel: w1228 -> [_ w1258]
          tunnel: w1225 -> [w1237 w1255]
          tunnel: [w1237 w1254] -> w1224
          tunnel: w1223 -> [_ w1253]
          tunnel: w1222 -> [_ w1252]
          tunnel: w1221 -> [_ w1247]
          tunnel: w1219 -> [_ w1245]
          tunnel: w1218 -> [_ w1244]
          tunnel: w1217 -> [_ w1240]
          tunnel: w1216 -> [_ w1239]
          tunnel: w1215 -> [_ _]
          tunnel: w1214 -> [_ _]
          frame False {
          }
          frame True {
            # "False: 1st frame in fram accum"
            # "True: Last Frame of frame accum"
            # "Current Line in Frame Accum"
            # "Current Line In Frame"
            n409 = Increment(x=w1255) -> (x+1=w1248:u32)
            n410 = Dequeue Element(queue=w1258) -> (element=w1273:u64[])  [unwired: 2 in, 3 out]
            n411 = Equal?(x=w1248, y=w1252) -> (x = y?=w1257:bool)
            n412 = Greater?(x=w1248, y=w1253) -> (0:w1250:bool)
            n413 = Greater?(x=w1248, y=w1247) -> (0:w1246:bool)
            n414 = Split Number(x=w1273) -> (hi(x)=w1274:u32[], lo(x)=w1272:u32[])
            n415 = Split Number(x=w1274) -> (hi(x)=w1241:u16[])  [unwired: 1 out]
            n416 = Split Number(x=w1272) -> (lo(x)=w1271:u16[])  [unwired: 1 out]
            n417 = Select(t=u32 0, s=w1257, f=w1248) -> (s? t:f=w1254:u32)
            n418 = Increment(x=w1266) -> (x+1=w1268:i32)
            n419 = Equal?(x=w1265, y=w1266) -> (x = y?=w1267:bool)
            n420 = Select(t=0, s=w1267, f=w1268) -> (s? t:f=w1264:i32)
            n421 = Build Array(0, w1266, w1265, w1266) -> (w1263:i32[])
            n422 = case shown="True" w1246 {
              tunnel: w1241 -> [w1288 w1303]
              tunnel: w1271 -> [w1285 w1302]
              tunnel: [w1287 w1298] -> w1262
              tunnel: [w1284 w1297] -> w1261
              tunnel: w1263 -> [_ w1294]
              tunnel: w1259 -> [w1283 w1292]
              tunnel: w1245 -> [w1282 w1291]
              tunnel: w1244 -> [w1281 w1290]
              tunnel: [w1282 w1291] -> w1243
              tunnel: [w1281 w1290] -> w1242
              frame False {
                n423 = To Single Precision Float(number=w1288) -> (single precision float=w1289:sgl[])
                n424 = To Single Precision Float(number=w1285) -> (single precision float=w1286:sgl[])
                n425 = Divide(x=w1289, y=w1283) -> (x/y=w1287:sgl[])
                n426 = Divide(x=w1286, y=w1283) -> (x/y=w1284:sgl[])
              }
              frame True {
                n427 = To Single Precision Float(number=w1303) -> (single precision float=w1293:sgl[])
                n428 = To Single Precision Float(number=w1302) -> (single precision float=w1301:sgl[])
                n429 = call "IMAQ GetPixelLine"("Line Coordinates"=w1294, "Image"=w1291) -> ("Pixels Line (Float)"=w1296:sgl[])  [unwired: 2 in, 4 out]
                n430 = call "IMAQ GetPixelLine"("Line Coordinates"=w1294, "Image"=w1290) -> ("Pixels Line (Float)"=w1295:sgl[])  [unwired: 2 in, 4 out]
                n431 = Divide(x=w1293, y=w1292) -> (x/y=w1300:sgl[])
                n432 = Divide(x=w1301, y=w1292) -> (x/y=w1299:sgl[])
                n433 = Add(x=w1296, y=w1300) -> (x+y=w1298:sgl[])
                n434 = Add(x=w1295, y=w1299) -> (x+y=w1297:sgl[])
              }
            }
            n435 = call "IMAQ SetPixelLine"("Pixels Line (Float)"=w1262, "Line Coordinates"=w1263, "Image"=w1243) -> ()  [unwired: 7 in, 2 out]
            n436 = call "IMAQ SetPixelLine"("Pixels Line (Float)"=w1261, "Line Coordinates"=w1263, "Image"=w1242) -> ()  [unwired: 7 in, 2 out]
            n437 = And(x=w1250, y=w1249) -> (x .and. y?=w1251:bool)
            n438 = case shown="True" w1251 {
              tunnel: w1262 -> [_ w1280]
              tunnel: w1261 -> [_ w1279]
              tunnel: w1260 -> [_ w1277]
              tunnel: w1240 -> [_ w1276]
              tunnel: w1239 -> [_ w1275]
              frame False {
              }
              frame True {
                w1278 = FALSE ("prepend array or string size? (T)")
                n439 = Write to Binary File(file (use dialog)=w1276, data=w1280, 5:w1278, 9:w1277) -> ()  [unwired: 2 in, 3 out]
                n440 = Write to Binary File(file (use dialog)=w1275, data=w1279, 5:w1278, 9:w1277) -> ()  [unwired: 2 in, 3 out]
              }
            }
          }
        }
      }
    }
    frame 10 {
      n441 = while {
        shift-right: [w1341] -> _
        shift-left: 0 -> [w1342]
        tunnel: w1319 -> [w1343]
        tunnel: w1318 -> [w1340]
        tunnel: w1317 -> [w1339]
        tunnel: w1316 -> [w1338]
        tunnel: w1304 -> [w1334]
        shift-right: [w1331] -> _
        shift-left: u32 0 -> [w1332]
        tunnel: w1314 -> [w1330]
        tunnel: w1313 -> [w1329]
        tunnel: w1312 -> [w1328]
        tunnel: w1311 -> [w1327]
        tunnel: w1306 -> [w1326]
        tunnel: w1305 -> [w1325]
        tunnel: w1310 -> [w1324]
        tunnel: w1309 -> [w1323]
        tunnel: w1308 -> [w1322]
        tunnel: w1307 -> [w1321]
        stop <- w1333 stop-if-true
        n442 = Get Queue Status(queue=w1327) -> (queue out=w1335:refnum<queue>, # elements in queue=w1337:i32)  [unwired: 2 in, 6 out]
        n443 = Get Notifier Status(notifier=w1334) -> (current notification=w1333:bool)  [unwired: 1 in, 4 out]
        n444 = Greater Than 0?(x=w1337) -> (x > 0?=w1336:bool)
        n445 = case shown="True" w1336 {
          tunnel: w1343 -> [_ w1371]
          tunnel: w1342 -> [w1345 w1372]
          tunnel: [w1345 w1370] -> w1341
          tunnel: w1340 -> [_ w1366]
          tunnel: w1339 -> [_ w1365]
          tunnel: w1338 -> [_ w1355]
          tunnel: w1335 -> [_ w1364]
          tunnel: w1332 -> [w1344 w1361]
          tunnel: [w1344 w1360] -> w1331
          tunnel: w1330 -> [_ w1359]
          tunnel: w1329 -> [_ w1358]
          tunnel: w1328 -> [_ w1353]
          tunnel: w1326 -> [_ w1351]
          tunnel: w1325 -> [_ w1350]
          tunnel: w1324 -> [_ w1347]
          tunnel: w1323 -> [_ w1346]
          tunnel: w1322 -> [_ _]
          tunnel: w1321 -> [_ _]
          frame False {
          }
          frame True {
            # "False: 1st frame in fram accum"
            # "True: Last Frame of frame accum"
            # "Current Line in Frame Accum"
            # "Current Line In Frame"
            n446 = Increment(x=w1361) -> (x+1=w1354:u32)
            n447 = Dequeue Element(queue=w1364) -> (element=w1380:u64[])  [unwired: 2 in, 3 out]
            n448 = Equal?(x=w1354, y=w1358) -> (x = y?=w1363:bool)
            n449 = Greater?(x=w1354, y=w1359) -> (0:w1356:bool)
            n450 = Greater?(x=w1354, y=w1353) -> (0:w1352:bool)
            n451 = Split Number(x=w1380) -> (hi(x)=w1381:u32[], lo(x)=w1379:u32[])
            n452 = Split Number(x=w1381) -> (lo(x)=w1378:u16[])  [unwired: 1 out]
            n453 = Split Number(x=w1379) -> (lo(x)=w1377:u16[])  [unwired: 1 out]
            n454 = Select(t=u32 0, s=w1363, f=w1354) -> (s? t:f=w1360:u32)
            n455 = Increment(x=w1372) -> (x+1=w1374:i32)
            n456 = Equal?(x=w1371, y=w1372) -> (x = y?=w1373:bool)
            n457 = Select(t=0, s=w1373, f=w1374) -> (s? t:f=w1370:i32)
            n458 = Build Array(0, w1372, w1371, w1372) -> (w1369:i32[])
            n459 = case shown="True" w1352 {
              tunnel: w1378 -> [w1394 w1410]
              tunnel: w1377 -> [w1393 w1409]
              tunnel: [w1392 w1404] -> w1368
              tunnel: [w1391 w1403] -> w1367
              tunnel: w1369 -> [_ w1400]
              tunnel: w1365 -> [w1390 w1399]
              tunnel: w1351 -> [w1389 w1398]
              tunnel: w1350 -> [w1388 w1397]
              tunnel: [w1389 w1398] -> w1349
              tunnel: [w1388 w1397] -> w1348
              frame False {
                n460 = To Single Precision Float(number=w1394) -> (single precision float=w1396:sgl[])
                n461 = To Single Precision Float(number=w1393) -> (single precision float=w1395:sgl[])
                n462 = Divide(x=w1396, y=w1390) -> (x/y=w1392:sgl[])
                n463 = Divide(x=w1395, y=w1390) -> (x/y=w1391:sgl[])
              }
              frame True {
                n464 = To Single Precision Float(number=w1410) -> (single precision float=w1408:sgl[])
                n465 = To Single Precision Float(number=w1409) -> (single precision float=w1407:sgl[])
                n466 = call "IMAQ GetPixelLine"("Line Coordinates"=w1400, "Image"=w1398) -> ("Pixels Line (Float)"=w1402:sgl[])  [unwired: 2 in, 4 out]
                n467 = call "IMAQ GetPixelLine"("Line Coordinates"=w1400, "Image"=w1397) -> ("Pixels Line (Float)"=w1401:sgl[])  [unwired: 2 in, 4 out]
                n468 = Divide(x=w1408, y=w1399) -> (x/y=w1406:sgl[])
                n469 = Divide(x=w1407, y=w1399) -> (x/y=w1405:sgl[])
                n470 = Add(x=w1402, y=w1406) -> (x+y=w1404:sgl[])
                n471 = Add(x=w1401, y=w1405) -> (x+y=w1403:sgl[])
              }
            }
            n472 = call "IMAQ SetPixelLine"("Pixels Line (Float)"=w1368, "Line Coordinates"=w1369, "Image"=w1349) -> ()  [unwired: 7 in, 2 out]
            n473 = call "IMAQ SetPixelLine"("Pixels Line (Float)"=w1367, "Line Coordinates"=w1369, "Image"=w1348) -> ()  [unwired: 7 in, 2 out]
            n474 = And(x=w1356, y=w1355) -> (x .and. y?=w1357:bool)
            n475 = case shown="True" w1357 {
              tunnel: w1368 -> [_ w1387]
              tunnel: w1367 -> [_ w1386]
              tunnel: w1366 -> [_ w1384]
              tunnel: w1347 -> [_ w1383]
              tunnel: w1346 -> [_ w1382]
              frame False {
              }
              frame True {
                w1385 = FALSE ("prepend array or string size? (T)")
                n476 = Write to Binary File(file (use dialog)=w1383, data=w1387, 5:w1385, 9:w1384) -> ()  [unwired: 2 in, 3 out]
                n477 = Write to Binary File(file (use dialog)=w1382, data=w1386, 5:w1385, 9:w1384) -> ()  [unwired: 2 in, 3 out]
              }
            }
          }
        }
      }
    }
    frame 11 {
      n478 = while {
        shift-right: [w1450] -> _
        shift-left: 0 -> [w1451]
        tunnel: w1427 -> [w1452]
        tunnel: w1426 -> [w1449]
        tunnel: w1425 -> [w1448]
        tunnel: w1424 -> [w1447]
        tunnel: w1411 -> [w1443]
        shift-right: [w1440] -> _
        shift-left: u32 0 -> [w1441]
        tunnel: w1422 -> [w1439]
        tunnel: w1421 -> [w1438]
        tunnel: w1420 -> [w1437]
        tunnel: w1419 -> [w1436]
        tunnel: w1414 -> [w1435]
        tunnel: w1413 -> [w1434]
        tunnel: w1412 -> [w1433]
        tunnel: w1418 -> [w1432]
        tunnel: w1417 -> [w1431]
        tunnel: w1416 -> [w1430]
        tunnel: w1415 -> [w1429]
        stop <- w1442 stop-if-true
        n479 = Get Queue Status(queue=w1436) -> (queue out=w1444:refnum<queue>, # elements in queue=w1446:i32)  [unwired: 2 in, 6 out]
        n480 = Get Notifier Status(notifier=w1443) -> (current notification=w1442:bool)  [unwired: 1 in, 4 out]
        n481 = Greater Than 0?(x=w1446) -> (x > 0?=w1445:bool)
        n482 = case shown="True" w1445 {
          tunnel: w1452 -> [_ w1485]
          tunnel: w1451 -> [w1454 w1486]
          tunnel: [w1454 w1484] -> w1450
          tunnel: w1449 -> [_ w1479]
          tunnel: w1448 -> [_ w1478]
          tunnel: w1447 -> [_ w1468]
          tunnel: w1444 -> [_ w1477]
          tunnel: w1441 -> [w1453 w1474]
          tunnel: [w1453 w1473] -> w1440
          tunnel: w1439 -> [_ w1472]
          tunnel: w1438 -> [_ w1471]
          tunnel: w1437 -> [_ w1466]
          tunnel: w1435 -> [_ w1464]
          tunnel: w1434 -> [_ w1463]
          tunnel: w1433 -> [_ w1462]
          tunnel: w1432 -> [_ w1457]
          tunnel: w1431 -> [_ w1456]
          tunnel: w1430 -> [_ w1455]
          tunnel: w1429 -> [_ _]
          frame False {
          }
          frame True {
            # "False: 1st frame in fram accum"
            # "True: Last Frame of frame accum"
            # "Current Line in Frame Accum"
            # "Current Line In Frame"
            n483 = Increment(x=w1474) -> (x+1=w1467:u32)
            n484 = Dequeue Element(queue=w1477) -> (element=w1494:u64[])  [unwired: 2 in, 3 out]
            n485 = Equal?(x=w1467, y=w1471) -> (x = y?=w1476:bool)
            n486 = Greater?(x=w1467, y=w1472) -> (0:w1469:bool)
            n487 = Greater?(x=w1467, y=w1466) -> (0:w1465:bool)
            n488 = Split Number(x=w1494) -> (hi(x)=w1495:u32[], lo(x)=w1493:u32[])
            n489 = Split Number(x=w1495) -> (hi(x)=w1458:u16[], lo(x)=w1492:u16[])
            n490 = Split Number(x=w1493) -> (lo(x)=w1491:u16[])  [unwired: 1 out]
            n491 = Select(t=u32 0, s=w1476, f=w1467) -> (s? t:f=w1473:u32)
            n492 = Increment(x=w1486) -> (x+1=w1488:i32)
            n493 = Equal?(x=w1485, y=w1486) -> (x = y?=w1487:bool)
            n494 = Select(t=0, s=w1487, f=w1488) -> (s? t:f=w1484:i32)
            n495 = Build Array(0, w1486, w1485, w1486) -> (w1483:i32[])
            n496 = case shown="False" w1465 {
              tunnel: w1458 -> [w1515 w1536]
              tunnel: w1492 -> [w1511 w1535]
              tunnel: w1491 -> [w1510 w1534]
              tunnel: [w1509 w1528] -> w1481
              tunnel: [w1514 w1527] -> w1482
              tunnel: [w1508 w1526] -> w1480
              tunnel: w1483 -> [_ w1522]
              tunnel: w1478 -> [w1507 w1520]
              tunnel: w1464 -> [w1506 w1518]
              tunnel: w1463 -> [w1505 w1519]
              tunnel: w1462 -> [w1504 w1517]
              tunnel: [w1505 w1519] -> w1460
              tunnel: [w1506 w1518] -> w1461
              tunnel: [w1504 w1517] -> w1459
              frame False {
                n497 = To Single Precision Float(number=w1515) -> (single precision float=w1516:sgl[])
                n498 = To Single Precision Float(number=w1511) -> (single precision float=w1513:sgl[])
                n499 = To Single Precision Float(number=w1510) -> (single precision float=w1512:sgl[])
                n500 = Divide(x=w1516, y=w1507) -> (x/y=w1514:sgl[])
                n501 = Divide(x=w1513, y=w1507) -> (x/y=w1509:sgl[])
                n502 = Divide(x=w1512, y=w1507) -> (x/y=w1508:sgl[])
              }
              frame True {
                n503 = To Single Precision Float(number=w1536) -> (single precision float=w1521:sgl[])
                n504 = To Single Precision Float(number=w1535) -> (single precision float=w1533:sgl[])
                n505 = To Single Precision Float(number=w1534) -> (single precision float=w1532:sgl[])
                n506 = call "IMAQ GetPixelLine"("Line Coordinates"=w1522, "Image"=w1518) -> ("Pixels Line (Float)"=w1525:sgl[])  [unwired: 2 in, 4 out]
                n507 = call "IMAQ GetPixelLine"("Line Coordinates"=w1522, "Image"=w1519) -> ("Pixels Line (Float)"=w1524:sgl[])  [unwired: 2 in, 4 out]
                n508 = call "IMAQ GetPixelLine"("Line Coordinates"=w1522, "Image"=w1517) -> ("Pixels Line (Float)"=w1523:sgl[])  [unwired: 2 in, 4 out]
                n509 = Divide(x=w1521, y=w1520) -> (x/y=w1531:sgl[])
                n510 = Divide(x=w1533, y=w1520) -> (x/y=w1530:sgl[])
                n511 = Divide(x=w1532, y=w1520) -> (x/y=w1529:sgl[])
                n512 = Add(x=w1525, y=w1531) -> (x+y=w1527:sgl[])
                n513 = Add(x=w1524, y=w1530) -> (x+y=w1528:sgl[])
                n514 = Add(x=w1523, y=w1529) -> (x+y=w1526:sgl[])
              }
            }
            n515 = call "IMAQ SetPixelLine"("Pixels Line (Float)"=w1482, "Line Coordinates"=w1483, "Image"=w1461) -> ()  [unwired: 7 in, 2 out]
            n516 = call "IMAQ SetPixelLine"("Pixels Line (Float)"=w1481, "Line Coordinates"=w1483, "Image"=w1460) -> ()  [unwired: 7 in, 2 out]
            n517 = call "IMAQ SetPixelLine"("Pixels Line (Float)"=w1480, "Line Coordinates"=w1483, "Image"=w1459) -> ()  [unwired: 7 in, 2 out]
            n518 = And(x=w1469, y=w1468) -> (x .and. y?=w1470:bool)
            n519 = case shown="True" w1470 {
              tunnel: w1482 -> [_ w1503]
              tunnel: w1481 -> [_ w1502]
              tunnel: w1480 -> [_ w1501]
              tunnel: w1479 -> [_ w1499]
              tunnel: w1457 -> [_ w1498]
              tunnel: w1456 -> [_ w1497]
              tunnel: w1455 -> [_ w1496]
              frame False {
              }
              frame True {
                w1500 = FALSE ("prepend array or string size? (T)")
                n520 = Write to Binary File(file (use dialog)=w1498, data=w1503, 5:w1500, 9:w1499) -> ()  [unwired: 2 in, 3 out]
                n521 = Write to Binary File(file (use dialog)=w1497, data=w1502, 5:w1500, 9:w1499) -> ()  [unwired: 2 in, 3 out]
                n522 = Write to Binary File(file (use dialog)=w1496, data=w1501, 5:w1500, 9:w1499) -> ()  [unwired: 2 in, 3 out]
              }
            }
          }
        }
      }
    }
    frame 12 {
      n523 = while {
        shift-right: [w1574] -> _
        shift-left: 0 -> [w1575]
        tunnel: w1552 -> [w1576]
        tunnel: w1551 -> [w1573]
        tunnel: w1550 -> [w1572]
        tunnel: w1549 -> [w1571]
        tunnel: w1537 -> [w1567]
        shift-right: [w1564] -> _
        shift-left: u32 0 -> [w1565]
        tunnel: w1547 -> [w1563]
        tunnel: w1546 -> [w1562]
        tunnel: w1545 -> [w1561]
        tunnel: w1544 -> [w1560]
        tunnel: w1539 -> [w1559]
        tunnel: w1538 -> [w1558]
        tunnel: w1543 -> [w1557]
        tunnel: w1542 -> [w1556]
        tunnel: w1541 -> [w1555]
        tunnel: w1540 -> [w1554]
        stop <- w1566 stop-if-true
        n524 = Get Queue Status(queue=w1560) -> (queue out=w1568:refnum<queue>, # elements in queue=w1570:i32)  [unwired: 2 in, 6 out]
        n525 = Get Notifier Status(notifier=w1567) -> (current notification=w1566:bool)  [unwired: 1 in, 4 out]
        n526 = Greater Than 0?(x=w1570) -> (x > 0?=w1569:bool)
        n527 = case shown="True" w1569 {
          tunnel: w1576 -> [_ w1605]
          tunnel: w1575 -> [w1578 w1606]
          tunnel: [w1578 w1604] -> w1574
          tunnel: w1573 -> [_ w1600]
          tunnel: w1572 -> [_ w1599]
          tunnel: w1571 -> [_ w1589]
          tunnel: w1568 -> [_ w1598]
          tunnel: w1565 -> [w1577 w1595]
          tunnel: [w1577 w1594] -> w1564
          tunnel: w1563 -> [_ w1593]
          tunnel: w1562 -> [_ w1592]
          tunnel: w1561 -> [_ w1587]
          tunnel: w1559 -> [_ w1585]
          tunnel: w1558 -> [_ w1584]
          tunnel: w1557 -> [_ w1581]
          tunnel: w1556 -> [_ w1580]
          tunnel: w1555 -> [_ _]
          tunnel: w1554 -> [_ _]
          frame False {
          }
          frame True {
            # "False: 1st frame in fram accum"
            # "True: Last Frame of frame accum"
            # "Current Line in Frame Accum"
            # "Current Line In Frame"
            n528 = Increment(x=w1595) -> (x+1=w1588:u32)
            n529 = Dequeue Element(queue=w1598) -> (element=w1613:u64[])  [unwired: 2 in, 3 out]
            n530 = Equal?(x=w1588, y=w1592) -> (x = y?=w1597:bool)
            n531 = Greater?(x=w1588, y=w1593) -> (0:w1590:bool)
            n532 = Greater?(x=w1588, y=w1587) -> (0:w1586:bool)
            n533 = Split Number(x=w1613) -> (lo(x)=w1612:u32[])  [unwired: 1 out]
            n534 = Split Number(x=w1612) -> (hi(x)=w1579:u16[], lo(x)=w1611:u16[])
            n535 = Select(t=u32 0, s=w1597, f=w1588) -> (s? t:f=w1594:u32)
            n536 = Increment(x=w1606) -> (x+1=w1608:i32)
            n537 = Equal?(x=w1605, y=w1606) -> (x = y?=w1607:bool)
            n538 = Select(t=0, s=w1607, f=w1608) -> (s? t:f=w1604:i32)
            n539 = Build Array(0, w1606, w1605, w1606) -> (w1603:i32[])
            n540 = case shown="True" w1586 {
              tunnel: w1579 -> [w1627 w1642]
              tunnel: w1611 -> [w1624 w1641]
              tunnel: [w1626 w1637] -> w1602
              tunnel: [w1623 w1636] -> w1601
              tunnel: w1603 -> [_ w1633]
              tunnel: w1599 -> [w1622 w1631]
              tunnel: w1585 -> [w1621 w1630]
              tunnel: w1584 -> [w1620 w1629]
              tunnel: [w1621 w1630] -> w1583
              tunnel: [w1620 w1629] -> w1582
              frame False {
                n541 = To Single Precision Float(number=w1627) -> (single precision float=w1628:sgl[])
                n542 = To Single Precision Float(number=w1624) -> (single precision float=w1625:sgl[])
                n543 = Divide(x=w1628, y=w1622) -> (x/y=w1626:sgl[])
                n544 = Divide(x=w1625, y=w1622) -> (x/y=w1623:sgl[])
              }
              frame True {
                n545 = To Single Precision Float(number=w1642) -> (single precision float=w1632:sgl[])
                n546 = To Single Precision Float(number=w1641) -> (single precision float=w1640:sgl[])
                n547 = call "IMAQ GetPixelLine"("Line Coordinates"=w1633, "Image"=w1630) -> ("Pixels Line (Float)"=w1635:sgl[])  [unwired: 2 in, 4 out]
                n548 = call "IMAQ GetPixelLine"("Line Coordinates"=w1633, "Image"=w1629) -> ("Pixels Line (Float)"=w1634:sgl[])  [unwired: 2 in, 4 out]
                n549 = Divide(x=w1632, y=w1631) -> (x/y=w1639:sgl[])
                n550 = Divide(x=w1640, y=w1631) -> (x/y=w1638:sgl[])
                n551 = Add(x=w1635, y=w1639) -> (x+y=w1637:sgl[])
                n552 = Add(x=w1634, y=w1638) -> (x+y=w1636:sgl[])
              }
            }
            n553 = call "IMAQ SetPixelLine"("Pixels Line (Float)"=w1602, "Line Coordinates"=w1603, "Image"=w1583) -> ()  [unwired: 7 in, 2 out]
            n554 = call "IMAQ SetPixelLine"("Pixels Line (Float)"=w1601, "Line Coordinates"=w1603, "Image"=w1582) -> ()  [unwired: 7 in, 2 out]
            n555 = And(x=w1590, y=w1589) -> (x .and. y?=w1591:bool)
            n556 = case shown="True" w1591 {
              tunnel: w1602 -> [_ w1619]
              tunnel: w1601 -> [_ w1618]
              tunnel: w1600 -> [_ w1616]
              tunnel: w1581 -> [_ w1615]
              tunnel: w1580 -> [_ w1614]
              frame False {
              }
              frame True {
                w1617 = FALSE ("prepend array or string size? (T)")
                n557 = Write to Binary File(file (use dialog)=w1615, data=w1619, 5:w1617, 9:w1616) -> ()  [unwired: 2 in, 3 out]
                n558 = Write to Binary File(file (use dialog)=w1614, data=w1618, 5:w1617, 9:w1616) -> ()  [unwired: 2 in, 3 out]
              }
            }
          }
        }
      }
    }
    frame 13 {
      n559 = while {
        shift-right: [w1682] -> _
        shift-left: 0 -> [w1683]
        tunnel: w1659 -> [w1684]
        tunnel: w1658 -> [w1681]
        tunnel: w1657 -> [w1680]
        tunnel: w1656 -> [w1679]
        tunnel: w1643 -> [w1675]
        shift-right: [w1672] -> _
        shift-left: u32 0 -> [w1673]
        tunnel: w1654 -> [w1671]
        tunnel: w1653 -> [w1670]
        tunnel: w1652 -> [w1669]
        tunnel: w1651 -> [w1668]
        tunnel: w1646 -> [w1667]
        tunnel: w1645 -> [w1666]
        tunnel: w1644 -> [w1665]
        tunnel: w1650 -> [w1664]
        tunnel: w1649 -> [w1663]
        tunnel: w1648 -> [w1662]
        tunnel: w1647 -> [w1661]
        stop <- w1674 stop-if-true
        n560 = Get Queue Status(queue=w1668) -> (queue out=w1676:refnum<queue>, # elements in queue=w1678:i32)  [unwired: 2 in, 6 out]
        n561 = Get Notifier Status(notifier=w1675) -> (current notification=w1674:bool)  [unwired: 1 in, 4 out]
        n562 = Greater Than 0?(x=w1678) -> (x > 0?=w1677:bool)
        n563 = case shown="True" w1677 {
          tunnel: w1684 -> [_ w1717]
          tunnel: w1683 -> [w1686 w1718]
          tunnel: [w1686 w1716] -> w1682
          tunnel: w1681 -> [_ w1711]
          tunnel: w1680 -> [_ w1710]
          tunnel: w1679 -> [_ w1700]
          tunnel: w1676 -> [_ w1709]
          tunnel: w1673 -> [w1685 w1706]
          tunnel: [w1685 w1705] -> w1672
          tunnel: w1671 -> [_ w1704]
          tunnel: w1670 -> [_ w1703]
          tunnel: w1669 -> [_ w1698]
          tunnel: w1667 -> [_ w1696]
          tunnel: w1666 -> [_ w1695]
          tunnel: w1665 -> [_ w1694]
          tunnel: w1664 -> [_ w1689]
          tunnel: w1663 -> [_ w1688]
          tunnel: w1662 -> [_ w1687]
          tunnel: w1661 -> [_ _]
          frame False {
          }
          frame True {
            # "False: 1st frame in fram accum"
            # "True: Last Frame of frame accum"
            # "Current Line in Frame Accum"
            # "Current Line In Frame"
            n564 = Increment(x=w1706) -> (x+1=w1699:u32)
            n565 = Dequeue Element(queue=w1709) -> (element=w1726:u64[])  [unwired: 2 in, 3 out]
            n566 = Equal?(x=w1699, y=w1703) -> (x = y?=w1708:bool)
            n567 = Greater?(x=w1699, y=w1704) -> (0:w1701:bool)
            n568 = Greater?(x=w1699, y=w1698) -> (0:w1697:bool)
            n569 = Split Number(x=w1726) -> (hi(x)=w1727:u32[], lo(x)=w1725:u32[])
            n570 = Split Number(x=w1727) -> (hi(x)=w1690:u16[])  [unwired: 1 out]
            n571 = Split Number(x=w1725) -> (hi(x)=w1724:u16[], lo(x)=w1723:u16[])
            n572 = Select(t=u32 0, s=w1708, f=w1699) -> (s? t:f=w1705:u32)
            n573 = Increment(x=w1718) -> (x+1=w1720:i32)
            n574 = Equal?(x=w1717, y=w1718) -> (x = y?=w1719:bool)
            n575 = Select(t=0, s=w1719, f=w1720) -> (s? t:f=w1716:i32)
            n576 = Build Array(0, w1718, w1717, w1718) -> (w1715:i32[])
            n577 = case shown="True" w1697 {
              tunnel: w1690 -> [w1747 w1768]
              tunnel: w1724 -> [w1743 w1767]
              tunnel: w1723 -> [w1742 w1766]
              tunnel: [w1741 w1760] -> w1713
              tunnel: [w1746 w1759] -> w1714
              tunnel: [w1740 w1758] -> w1712
              tunnel: w1715 -> [_ w1754]
              tunnel: w1710 -> [w1739 w1752]
              tunnel: w1696 -> [w1738 w1750]
              tunnel: w1695 -> [w1737 w1751]
              tunnel: w1694 -> [w1736 w1749]
              tunnel: [w1737 w1751] -> w1692
              tunnel: [w1738 w1750] -> w1693
              tunnel: [w1736 w1749] -> w1691
              frame False {
                n578 = To Single Precision Float(number=w1747) -> (single precision float=w1748:sgl[])
                n579 = To Single Precision Float(number=w1743) -> (single precision float=w1745:sgl[])
                n580 = To Single Precision Float(number=w1742) -> (single precision float=w1744:sgl[])
                n581 = Divide(x=w1748, y=w1739) -> (x/y=w1746:sgl[])
                n582 = Divide(x=w1745, y=w1739) -> (x/y=w1741:sgl[])
                n583 = Divide(x=w1744, y=w1739) -> (x/y=w1740:sgl[])
              }
              frame True {
                n584 = To Single Precision Float(number=w1768) -> (single precision float=w1753:sgl[])
                n585 = To Single Precision Float(number=w1767) -> (single precision float=w1765:sgl[])
                n586 = To Single Precision Float(number=w1766) -> (single precision float=w1764:sgl[])
                n587 = call "IMAQ GetPixelLine"("Line Coordinates"=w1754, "Image"=w1750) -> ("Pixels Line (Float)"=w1757:sgl[])  [unwired: 2 in, 4 out]
                n588 = call "IMAQ GetPixelLine"("Line Coordinates"=w1754, "Image"=w1751) -> ("Pixels Line (Float)"=w1756:sgl[])  [unwired: 2 in, 4 out]
                n589 = call "IMAQ GetPixelLine"("Line Coordinates"=w1754, "Image"=w1749) -> ("Pixels Line (Float)"=w1755:sgl[])  [unwired: 2 in, 4 out]
                n590 = Divide(x=w1753, y=w1752) -> (x/y=w1763:sgl[])
                n591 = Divide(x=w1765, y=w1752) -> (x/y=w1762:sgl[])
                n592 = Divide(x=w1764, y=w1752) -> (x/y=w1761:sgl[])
                n593 = Add(x=w1757, y=w1763) -> (x+y=w1759:sgl[])
                n594 = Add(x=w1756, y=w1762) -> (x+y=w1760:sgl[])
                n595 = Add(x=w1755, y=w1761) -> (x+y=w1758:sgl[])
              }
            }
            n596 = call "IMAQ SetPixelLine"("Pixels Line (Float)"=w1714, "Line Coordinates"=w1715, "Image"=w1693) -> ()  [unwired: 7 in, 2 out]
            n597 = call "IMAQ SetPixelLine"("Pixels Line (Float)"=w1713, "Line Coordinates"=w1715, "Image"=w1692) -> ()  [unwired: 7 in, 2 out]
            n598 = call "IMAQ SetPixelLine"("Pixels Line (Float)"=w1712, "Line Coordinates"=w1715, "Image"=w1691) -> ()  [unwired: 7 in, 2 out]
            n599 = And(x=w1701, y=w1700) -> (x .and. y?=w1702:bool)
            n600 = case shown="True" w1702 {
              tunnel: w1714 -> [_ w1735]
              tunnel: w1713 -> [_ w1734]
              tunnel: w1712 -> [_ w1733]
              tunnel: w1711 -> [_ w1731]
              tunnel: w1689 -> [_ w1730]
              tunnel: w1688 -> [_ w1729]
              tunnel: w1687 -> [_ w1728]
              frame False {
              }
              frame True {
                w1732 = FALSE ("prepend array or string size? (T)")
                n601 = Write to Binary File(file (use dialog)=w1730, data=w1735, 5:w1732, 9:w1731) -> ()  [unwired: 2 in, 3 out]
                n602 = Write to Binary File(file (use dialog)=w1729, data=w1734, 5:w1732, 9:w1731) -> ()  [unwired: 2 in, 3 out]
                n603 = Write to Binary File(file (use dialog)=w1728, data=w1733, 5:w1732, 9:w1731) -> ()  [unwired: 2 in, 3 out]
              }
            }
          }
        }
      }
    }
    frame 14 {
      n604 = while {
        shift-right: [w1808] -> _
        shift-left: 0 -> [w1809]
        tunnel: w1785 -> [w1810]
        tunnel: w1784 -> [w1807]
        tunnel: w1783 -> [w1806]
        tunnel: w1782 -> [w1805]
        tunnel: w1769 -> [w1801]
        shift-right: [w1798] -> _
        shift-left: u32 0 -> [w1799]
        tunnel: w1780 -> [w1797]
        tunnel: w1779 -> [w1796]
        tunnel: w1778 -> [w1795]
        tunnel: w1777 -> [w1794]
        tunnel: w1772 -> [w1789]
        tunnel: w1771 -> [w1788]
        tunnel: w1770 -> [w1787]
        tunnel: w1776 -> [w1793]
        tunnel: w1775 -> [w1792]
        tunnel: w1774 -> [w1791]
        tunnel: w1773 -> [w1790]
        stop <- w1800 stop-if-true
        n605 = Get Queue Status(queue=w1794) -> (queue out=w1802:refnum<queue>, # elements in queue=w1804:i32)  [unwired: 2 in, 6 out]
        n606 = Get Notifier Status(notifier=w1801) -> (current notification=w1800:bool)  [unwired: 1 in, 4 out]
        n607 = Greater Than 0?(x=w1804) -> (x > 0?=w1803:bool)
        n608 = case shown="True" w1803 {
          tunnel: w1810 -> [_ w1842]
          tunnel: w1809 -> [w1812 w1843]
          tunnel: [w1812 w1841] -> w1808
          tunnel: w1807 -> [_ w1836]
          tunnel: w1806 -> [_ w1835]
          tunnel: w1805 -> [_ w1825]
          tunnel: w1802 -> [_ w1834]
          tunnel: w1799 -> [w1811 w1831]
          tunnel: [w1811 w1830] -> w1798
          tunnel: w1797 -> [_ w1829]
          tunnel: w1796 -> [_ w1828]
          tunnel: w1795 -> [_ w1823]
          tunnel: w1789 -> [_ w1821]
          tunnel: w1788 -> [_ w1820]
          tunnel: w1787 -> [_ w1819]
          tunnel: w1793 -> [_ w1815]
          tunnel: w1792 -> [_ w1814]
          tunnel: w1791 -> [_ w1813]
          tunnel: w1790 -> [_ _]
          frame False {
          }
          frame True {
            # "False: 1st frame in fram accum"
            # "True: Last Frame of frame accum"
            # "Current Line in Frame Accum"
            # "Current Line In Frame"
            n609 = Increment(x=w1831) -> (x+1=w1824:u32)
            n610 = Dequeue Element(queue=w1834) -> (element=w1852:u64[])  [unwired: 2 in, 3 out]
            n611 = Equal?(x=w1824, y=w1828) -> (x = y?=w1833:bool)
            n612 = Greater?(x=w1824, y=w1829) -> (0:w1826:bool)
            n613 = Greater?(x=w1824, y=w1823) -> (0:w1822:bool)
            n614 = Split Number(x=w1852) -> (hi(x)=w1853:u32[], lo(x)=w1851:u32[])
            n615 = Split Number(x=w1853) -> (lo(x)=w1850:u16[])  [unwired: 1 out]
            n616 = Split Number(x=w1851) -> (hi(x)=w1849:u16[], lo(x)=w1848:u16[])
            n617 = Select(t=u32 0, s=w1833, f=w1824) -> (s? t:f=w1830:u32)
            n618 = Increment(x=w1843) -> (x+1=w1845:i32)
            n619 = Equal?(x=w1842, y=w1843) -> (x = y?=w1844:bool)
            n620 = Select(t=0, s=w1844, f=w1845) -> (s? t:f=w1841:i32)
            n621 = Build Array(0, w1843, w1842, w1843) -> (w1840:i32[])
            n622 = case shown="True" w1822 {
              tunnel: w1850 -> [w1871 w1894]
              tunnel: w1849 -> [w1870 w1893]
              tunnel: w1848 -> [w1869 w1892]
              tunnel: [w1867 w1885] -> w1838
              tunnel: [w1868 w1884] -> w1839
              tunnel: [w1866 w1883] -> w1837
              tunnel: w1840 -> [_ w1879]
              tunnel: w1835 -> [w1865 w1878]
              tunnel: w1821 -> [w1864 w1876]
              tunnel: w1820 -> [w1863 w1877]
              tunnel: w1819 -> [w1862 w1875]
              tunnel: [w1863 w1877] -> w1817
              tunnel: [w1864 w1876] -> w1818
              tunnel: [w1862 w1875] -> w1816
              frame False {
                n623 = To Single Precision Float(number=w1871) -> (single precision float=w1874:sgl[])
                n624 = To Single Precision Float(number=w1870) -> (single precision float=w1873:sgl[])
                n625 = To Single Precision Float(number=w1869) -> (single precision float=w1872:sgl[])
                n626 = Divide(x=w1874, y=w1865) -> (x/y=w1868:sgl[])
                n627 = Divide(x=w1873, y=w1865) -> (x/y=w1867:sgl[])
                n628 = Divide(x=w1872, y=w1865) -> (x/y=w1866:sgl[])
              }
              frame True {
                n629 = To Single Precision Float(number=w1894) -> (single precision float=w1891:sgl[])
                n630 = To Single Precision Float(number=w1893) -> (single precision float=w1890:sgl[])
                n631 = To Single Precision Float(number=w1892) -> (single precision float=w1889:sgl[])
                n632 = call "IMAQ GetPixelLine"("Line Coordinates"=w1879, "Image"=w1876) -> ("Pixels Line (Float)"=w1882:sgl[])  [unwired: 2 in, 4 out]
                n633 = call "IMAQ GetPixelLine"("Line Coordinates"=w1879, "Image"=w1877) -> ("Pixels Line (Float)"=w1881:sgl[])  [unwired: 2 in, 4 out]
                n634 = call "IMAQ GetPixelLine"("Line Coordinates"=w1879, "Image"=w1875) -> ("Pixels Line (Float)"=w1880:sgl[])  [unwired: 2 in, 4 out]
                n635 = Divide(x=w1891, y=w1878) -> (x/y=w1888:sgl[])
                n636 = Divide(x=w1890, y=w1878) -> (x/y=w1887:sgl[])
                n637 = Divide(x=w1889, y=w1878) -> (x/y=w1886:sgl[])
                n638 = Add(x=w1882, y=w1888) -> (x+y=w1884:sgl[])
                n639 = Add(x=w1881, y=w1887) -> (x+y=w1885:sgl[])
                n640 = Add(x=w1880, y=w1886) -> (x+y=w1883:sgl[])
              }
            }
            n641 = call "IMAQ SetPixelLine"("Pixels Line (Float)"=w1839, "Line Coordinates"=w1840, "Image"=w1818) -> ()  [unwired: 7 in, 2 out]
            n642 = call "IMAQ SetPixelLine"("Pixels Line (Float)"=w1838, "Line Coordinates"=w1840, "Image"=w1817) -> ()  [unwired: 7 in, 2 out]
            n643 = call "IMAQ SetPixelLine"("Pixels Line (Float)"=w1837, "Line Coordinates"=w1840, "Image"=w1816) -> ()  [unwired: 7 in, 2 out]
            n644 = And(x=w1826, y=w1825) -> (x .and. y?=w1827:bool)
            n645 = case shown="True" w1827 {
              tunnel: w1839 -> [_ w1861]
              tunnel: w1838 -> [_ w1860]
              tunnel: w1837 -> [_ w1859]
              tunnel: w1836 -> [_ w1857]
              tunnel: w1815 -> [_ w1856]
              tunnel: w1814 -> [_ w1855]
              tunnel: w1813 -> [_ w1854]
              frame False {
              }
              frame True {
                w1858 = FALSE ("prepend array or string size? (T)")
                n646 = Write to Binary File(file (use dialog)=w1856, data=w1861, 5:w1858, 9:w1857) -> ()  [unwired: 2 in, 3 out]
                n647 = Write to Binary File(file (use dialog)=w1855, data=w1860, 5:w1858, 9:w1857) -> ()  [unwired: 2 in, 3 out]
                n648 = Write to Binary File(file (use dialog)=w1854, data=w1859, 5:w1858, 9:w1857) -> ()  [unwired: 2 in, 3 out]
              }
            }
          }
        }
      }
    }
    frame 15 {
      n649 = while {
        shift-right: [w1936] -> _
        shift-left: 0 -> [w1937]
        tunnel: w1912 -> [w1938]
        tunnel: w1911 -> [w1935]
        tunnel: w1910 -> [w1934]
        tunnel: w1909 -> [w1933]
        tunnel: w1895 -> [w1929]
        shift-right: [w1926] -> _
        shift-left: u32 0 -> [w1927]
        tunnel: w1907 -> [w1925]
        tunnel: w1906 -> [w1924]
        tunnel: w1905 -> [w1923]
        tunnel: w1904 -> [w1922]
        tunnel: w1899 -> [w1921]
        tunnel: w1898 -> [w1920]
        tunnel: w1897 -> [w1919]
        tunnel: w1896 -> [w1918]
        tunnel: w1903 -> [w1917]
        tunnel: w1902 -> [w1916]
        tunnel: w1901 -> [w1915]
        tunnel: w1900 -> [w1914]
        stop <- w1928 stop-if-true
        n650 = Get Queue Status(queue=w1922) -> (queue out=w1930:refnum<queue>, # elements in queue=w1932:i32)  [unwired: 2 in, 6 out]
        n651 = Get Notifier Status(notifier=w1929) -> (current notification=w1928:bool)  [unwired: 1 in, 4 out]
        n652 = Greater Than 0?(x=w1932) -> (x > 0?=w1931:bool)
        n653 = case shown="True" w1931 {
          tunnel: w1938 -> [_ w1975]
          tunnel: w1937 -> [w1940 w1976]
          tunnel: [w1940 w1974] -> w1936
          tunnel: w1935 -> [_ w1968]
          tunnel: w1934 -> [_ w1967]
          tunnel: w1933 -> [_ w1957]
          tunnel: w1930 -> [_ w1966]
          tunnel: w1927 -> [w1939 w1963]
          tunnel: [w1939 w1962] -> w1926
          tunnel: w1925 -> [_ w1961]
          tunnel: w1924 -> [_ w1960]
          tunnel: w1923 -> [_ w1955]
          tunnel: w1921 -> [_ w1953]
          tunnel: w1920 -> [_ w1952]
          tunnel: w1919 -> [_ w1951]
          tunnel: w1918 -> [_ w1950]
          tunnel: w1917 -> [_ w1944]
          tunnel: w1916 -> [_ w1943]
          tunnel: w1915 -> [_ w1942]
          tunnel: w1914 -> [_ w1941]
          frame False {
          }
          frame True {
            # "False: 1st frame in fram accum"
            # "True: Last Frame of frame accum"
            # "Current Line in Frame Accum"
            # "Current Line In Frame"
            n654 = Increment(x=w1963) -> (x+1=w1956:u32)
            n655 = Dequeue Element(queue=w1966) -> (element=w1985:u64[])  [unwired: 2 in, 3 out]
            n656 = Equal?(x=w1956, y=w1960) -> (x = y?=w1965:bool)
            n657 = Greater?(x=w1956, y=w1961) -> (0:w1958:bool)
            n658 = Greater?(x=w1956, y=w1955) -> (0:w1954:bool)
            n659 = Split Number(x=w1985) -> (hi(x)=w1986:u32[], lo(x)=w1984:u32[])
            n660 = Split Number(x=w1986) -> (hi(x)=w1945:u16[], lo(x)=w1983:u16[])
            n661 = Split Number(x=w1984) -> (hi(x)=w1982:u16[], lo(x)=w1981:u16[])
            n662 = Select(t=u32 0, s=w1965, f=w1956) -> (s? t:f=w1962:u32)
            n663 = Increment(x=w1976) -> (x+1=w1978:i32)
            n664 = Equal?(x=w1975, y=w1976) -> (x = y?=w1977:bool)
            n665 = Select(t=0, s=w1977, f=w1978) -> (s? t:f=w1974:i32)
            n666 = Build Array(0, w1976, w1975, w1976) -> (w1973:i32[])
            n667 = case shown="True" w1954 {
              tunnel: w1945 -> [w2012 w2039]
              tunnel: w1983 -> [w2007 w2038]
              tunnel: w1982 -> [w2006 w2037]
              tunnel: w1981 -> [w2005 w2036]
              tunnel: [w2003 w2028] -> w1970
              tunnel: [w2004 w2027] -> w1971
              tunnel: [w2011 w2026] -> w1972
              tunnel: [w2002 w2025] -> w1969
              tunnel: w1973 -> [_ w2020]
              tunnel: w1967 -> [w2001 w2018]
              tunnel: w1953 -> [w2000 w2015]
              tunnel: w1952 -> [w1999 w2016]
              tunnel: w1951 -> [w1998 w2017]
              tunnel: w1950 -> [w1997 w2014]
              tunnel: [w1998 w2017] -> w1947
              tunnel: [w1999 w2016] -> w1948
              tunnel: [w2000 w2015] -> w1949
              tunnel: [w1997 w2014] -> w1946
              frame False {
                n668 = To Single Precision Float(number=w2012) -> (single precision float=w2013:sgl[])
                n669 = To Single Precision Float(number=w2007) -> (single precision float=w2010:sgl[])
                n670 = To Single Precision Float(number=w2006) -> (single precision float=w2009:sgl[])
                n671 = To Single Precision Float(number=w2005) -> (single precision float=w2008:sgl[])
                n672 = Divide(x=w2013, y=w2001) -> (x/y=w2011:sgl[])
                n673 = Divide(x=w2010, y=w2001) -> (x/y=w2004:sgl[])
                n674 = Divide(x=w2009, y=w2001) -> (x/y=w2003:sgl[])
                n675 = Divide(x=w2008, y=w2001) -> (x/y=w2002:sgl[])
              }
              frame True {
                n676 = To Single Precision Float(number=w2039) -> (single precision float=w2019:sgl[])
                n677 = To Single Precision Float(number=w2038) -> (single precision float=w2035:sgl[])
                n678 = To Single Precision Float(number=w2037) -> (single precision float=w2034:sgl[])
                n679 = To Single Precision Float(number=w2036) -> (single precision float=w2033:sgl[])
                n680 = call "IMAQ GetPixelLine"("Line Coordinates"=w2020, "Image"=w2015) -> ("Pixels Line (Float)"=w2024:sgl[])  [unwired: 2 in, 4 out]
                n681 = call "IMAQ GetPixelLine"("Line Coordinates"=w2020, "Image"=w2016) -> ("Pixels Line (Float)"=w2023:sgl[])  [unwired: 2 in, 4 out]
                n682 = call "IMAQ GetPixelLine"("Line Coordinates"=w2020, "Image"=w2017) -> ("Pixels Line (Float)"=w2022:sgl[])  [unwired: 2 in, 4 out]
                n683 = call "IMAQ GetPixelLine"("Line Coordinates"=w2020, "Image"=w2014) -> ("Pixels Line (Float)"=w2021:sgl[])  [unwired: 2 in, 4 out]
                n684 = Divide(x=w2019, y=w2018) -> (x/y=w2032:sgl[])
                n685 = Divide(x=w2035, y=w2018) -> (x/y=w2031:sgl[])
                n686 = Divide(x=w2034, y=w2018) -> (x/y=w2030:sgl[])
                n687 = Divide(x=w2033, y=w2018) -> (x/y=w2029:sgl[])
                n688 = Add(x=w2024, y=w2032) -> (x+y=w2026:sgl[])
                n689 = Add(x=w2023, y=w2031) -> (x+y=w2027:sgl[])
                n690 = Add(x=w2022, y=w2030) -> (x+y=w2028:sgl[])
                n691 = Add(x=w2021, y=w2029) -> (x+y=w2025:sgl[])
              }
            }
            n692 = call "IMAQ SetPixelLine"("Pixels Line (Float)"=w1972, "Line Coordinates"=w1973, "Image"=w1949) -> ()  [unwired: 7 in, 2 out]
            n693 = call "IMAQ SetPixelLine"("Pixels Line (Float)"=w1971, "Line Coordinates"=w1973, "Image"=w1948) -> ()  [unwired: 7 in, 2 out]
            n694 = call "IMAQ SetPixelLine"("Pixels Line (Float)"=w1970, "Line Coordinates"=w1973, "Image"=w1947) -> ()  [unwired: 7 in, 2 out]
            n695 = call "IMAQ SetPixelLine"("Pixels Line (Float)"=w1969, "Line Coordinates"=w1973, "Image"=w1946) -> ()  [unwired: 7 in, 2 out]
            n696 = And(x=w1958, y=w1957) -> (x .and. y?=w1959:bool)
            n697 = case shown="True" w1959 {
              tunnel: w1972 -> [_ w1996]
              tunnel: w1971 -> [_ w1995]
              tunnel: w1970 -> [_ w1994]
              tunnel: w1969 -> [_ w1993]
              tunnel: w1968 -> [_ w1991]
              tunnel: w1944 -> [_ w1990]
              tunnel: w1943 -> [_ w1989]
              tunnel: w1942 -> [_ w1988]
              tunnel: w1941 -> [_ w1987]
              frame False {
              }
              frame True {
                w1992 = FALSE ("prepend array or string size? (T)")
                n698 = Write to Binary File(file (use dialog)=w1990, data=w1996, 5:w1992, 9:w1991) -> ()  [unwired: 2 in, 3 out]
                n699 = Write to Binary File(file (use dialog)=w1989, data=w1995, 5:w1992, 9:w1991) -> ()  [unwired: 2 in, 3 out]
                n700 = Write to Binary File(file (use dialog)=w1988, data=w1994, 5:w1992, 9:w1991) -> ()  [unwired: 2 in, 3 out]
                n701 = Write to Binary File(file (use dialog)=w1987, data=w1993, 5:w1992, 9:w1991) -> ()  [unwired: 2 in, 3 out]
              }
            }
          }
        }
      }
    }
    frame 19 {
      n702 = while {
        shift-right: [w2075] -> _
        shift-left: 0 -> [w2076]
        tunnel: w2054 -> [w2077]
        tunnel: w2053 -> [w2074]
        tunnel: w2052 -> [w2073]
        tunnel: w2051 -> [w2072]
        tunnel: w2040 -> [w2068]
        shift-right: [w2065] -> _
        shift-left: u32 0 -> [w2066]
        tunnel: w2049 -> [w2064]
        tunnel: w2048 -> [w2063]
        tunnel: w2047 -> [w2062]
        tunnel: w2046 -> [w2061]
        tunnel: w2041 -> [w2060]
        tunnel: w2045 -> [w2059]
        tunnel: w2044 -> [w2058]
        tunnel: w2043 -> [w2057]
        tunnel: w2042 -> [w2056]
        stop <- w2067 stop-if-true
        n703 = Get Queue Status(queue=w2061) -> (queue out=w2069:refnum<queue>, # elements in queue=w2071:i32)  [unwired: 2 in, 6 out]
        n704 = Get Notifier Status(notifier=w2068) -> (current notification=w2067:bool)  [unwired: 1 in, 4 out]
        n705 = Greater Than 0?(x=w2071) -> (x > 0?=w2070:bool)
        n706 = case shown="True" w2070 {
          tunnel: w2077 -> [_ w2106]
          tunnel: w2076 -> [w2079 w2107]
          tunnel: [w2079 w2105] -> w2075
          tunnel: w2074 -> [_ w2102]
          tunnel: w2073 -> [_ w2101]
          tunnel: w2072 -> [_ w2091]
          tunnel: w2069 -> [_ w2100]
          tunnel: w2066 -> [w2078 w2097]
          tunnel: [w2078 w2096] -> w2065
          tunnel: w2064 -> [_ w2095]
          tunnel: w2063 -> [_ w2094]
          tunnel: w2062 -> [_ w2089]
          tunnel: w2060 -> [_ w2087]
          tunnel: w2059 -> [_ w2085]
          tunnel: w2058 -> [_ _]
          tunnel: w2057 -> [_ _]
          tunnel: w2056 -> [_ _]
          frame False {
          }
          frame True {
            # "True: Last Frame of frame accum"
            # "Current Line in Frame Accum"
            # "Current Line In Frame"
            n707 = Increment(x=w2097) -> (x+1=w2090:u32)
            n708 = Dequeue Element(queue=w2100) -> (element=w2112:u64[])  [unwired: 2 in, 3 out]
            n709 = Equal?(x=w2090, y=w2094) -> (x = y?=w2099:bool)
            n710 = Greater?(x=w2090, y=w2095) -> (0:w2092:bool)
            n711 = Greater?(x=w2090, y=w2089) -> (0:w2088:bool)
            n712 = Split Number(x=w2112) -> (hi(x)=w2113:u32[])  [unwired: 1 out]
            n713 = Split Number(x=w2113) -> (hi(x)=w2084:u16[], lo(x)=w2083:u16[])
            n714 = Select(t=u32 0, s=w2099, f=w2090) -> (s? t:f=w2096:u32)
            n715 = Increment(x=w2107) -> (x+1=w2109:i32)
            n716 = Equal?(x=w2106, y=w2107) -> (x = y?=w2108:bool)
            n717 = To Single Precision Float(number=w2084) -> (single precision float=w2082:sgl[])
            n718 = To Single Precision Float(number=w2083) -> (single precision float=w2081:sgl[])
            n719 = Select(t=0, s=w2108, f=w2109) -> (s? t:f=w2105:i32)
            n720 = Add(x=w2082, y=w2081) -> (x+y=w2080:sgl[])
            n721 = Build Array(0, w2107, w2106, w2107) -> (w2104:i32[])
            n722 = case shown="False" w2088 {
              tunnel: [w2121 w2127] -> w2103
              tunnel: w2104 -> [_ w2125]
              tunnel: w2101 -> [w2120 w2124]
              tunnel: w2087 -> [w2119 w2123]
              tunnel: [w2119 w2123] -> w2086
              tunnel: w2080 -> [w2118 w2122]
              frame False {
                n723 = Divide(x=w2118, y=w2120) -> (x/y=w2121:sgl[])
              }
              frame True {
                n724 = call "IMAQ GetPixelLine"("Line Coordinates"=w2125, "Image"=w2123) -> ("Pixels Line (Float)"=w2126:sgl[])  [unwired: 2 in, 4 out]
                n725 = Divide(x=w2122, y=w2124) -> (x/y=w2128:sgl[])
                n726 = Add(x=w2126, y=w2128) -> (x+y=w2127:sgl[])
              }
            }
            n727 = call "IMAQ SetPixelLine"("Pixels Line (Float)"=w2103, "Line Coordinates"=w2104, "Image"=w2086) -> ()  [unwired: 7 in, 2 out]
            n728 = And(x=w2092, y=w2091) -> (x .and. y?=w2093:bool)
            n729 = case shown="True" w2093 {
              tunnel: w2103 -> [_ w2117]
              tunnel: w2102 -> [_ w2115]
              tunnel: w2085 -> [_ w2114]
              frame False {
              }
              frame True {
                n730 = Write to Binary File(file (use dialog)=w2114, data=w2117, 5:FALSE ("prepend array or string size? (T)"), 9:w2115) -> ()  [unwired: 2 in, 3 out]
              }
            }
          }
        }
      }
    }
    frame 21 {
      n731 = while {
        shift-right: [w2164] -> _
        shift-left: 0 -> [w2165]
        tunnel: w2143 -> [w2166]
        tunnel: w2142 -> [w2163]
        tunnel: w2141 -> [w2162]
        tunnel: w2140 -> [w2161]
        tunnel: w2129 -> [w2157]
        shift-right: [w2154] -> _
        shift-left: u32 0 -> [w2155]
        tunnel: w2138 -> [w2153]
        tunnel: w2137 -> [w2152]
        tunnel: w2136 -> [w2151]
        tunnel: w2135 -> [w2150]
        tunnel: w2130 -> [w2149]
        tunnel: w2134 -> [w2148]
        tunnel: w2133 -> [w2147]
        tunnel: w2132 -> [w2146]
        tunnel: w2131 -> [w2145]
        stop <- w2156 stop-if-true
        n732 = Get Queue Status(queue=w2150) -> (queue out=w2158:refnum<queue>, # elements in queue=w2160:i32)  [unwired: 2 in, 6 out]
        n733 = Get Notifier Status(notifier=w2157) -> (current notification=w2156:bool)  [unwired: 1 in, 4 out]
        n734 = Greater Than 0?(x=w2160) -> (x > 0?=w2159:bool)
        n735 = case shown="True" w2159 {
          tunnel: w2166 -> [_ w2195]
          tunnel: w2165 -> [w2168 w2196]
          tunnel: [w2168 w2194] -> w2164
          tunnel: w2163 -> [_ w2191]
          tunnel: w2162 -> [_ w2190]
          tunnel: w2161 -> [_ w2180]
          tunnel: w2158 -> [_ w2189]
          tunnel: w2155 -> [w2167 w2186]
          tunnel: [w2167 w2185] -> w2154
          tunnel: w2153 -> [_ w2184]
          tunnel: w2152 -> [_ w2183]
          tunnel: w2151 -> [_ w2178]
          tunnel: w2149 -> [_ w2176]
          tunnel: w2148 -> [_ w2174]
          tunnel: w2147 -> [_ _]
          tunnel: w2146 -> [_ _]
          tunnel: w2145 -> [_ _]
          frame False {
          }
          frame True {
            # "True: Last Frame of frame accum"
            # "Current Line in Frame Accum"
            # "Current Line In Frame"
            n736 = Increment(x=w2186) -> (x+1=w2179:u32)
            n737 = Dequeue Element(queue=w2189) -> (element=w2202:u64[])  [unwired: 2 in, 3 out]
            n738 = Equal?(x=w2179, y=w2183) -> (x = y?=w2188:bool)
            n739 = Greater?(x=w2179, y=w2184) -> (0:w2181:bool)
            n740 = Greater?(x=w2179, y=w2178) -> (0:w2177:bool)
            n741 = Split Number(x=w2202) -> (hi(x)=w2203:u32[], lo(x)=w2201:u32[])
            n742 = Split Number(x=w2203) -> (hi(x)=w2173:u16[])  [unwired: 1 out]
            n743 = Split Number(x=w2201) -> (hi(x)=w2169:u16[])  [unwired: 1 out]
            n744 = Select(t=u32 0, s=w2188, f=w2179) -> (s? t:f=w2185:u32)
            n745 = Increment(x=w2196) -> (x+1=w2198:i32)
            n746 = Equal?(x=w2195, y=w2196) -> (x = y?=w2197:bool)
            n747 = To Single Precision Float(number=w2173) -> (single precision float=w2172:sgl[])
            n748 = To Single Precision Float(number=w2169) -> (single precision float=w2171:sgl[])
            n749 = Select(t=0, s=w2197, f=w2198) -> (s? t:f=w2194:i32)
            n750 = Add(x=w2172, y=w2171) -> (x+y=w2170:sgl[])
            n751 = Build Array(0, w2196, w2195, w2196) -> (w2193:i32[])
            n752 = case shown="False" w2177 {
              tunnel: [w2211 w2217] -> w2192
              tunnel: w2193 -> [_ w2215]
              tunnel: w2190 -> [w2210 w2214]
              tunnel: w2176 -> [w2209 w2213]
              tunnel: [w2209 w2213] -> w2175
              tunnel: w2170 -> [w2208 w2212]
              frame False {
                n753 = Divide(x=w2208, y=w2210) -> (x/y=w2211:sgl[])
              }
              frame True {
                n754 = call "IMAQ GetPixelLine"("Line Coordinates"=w2215, "Image"=w2213) -> ("Pixels Line (Float)"=w2216:sgl[])  [unwired: 2 in, 4 out]
                n755 = Divide(x=w2212, y=w2214) -> (x/y=w2218:sgl[])
                n756 = Add(x=w2216, y=w2218) -> (x+y=w2217:sgl[])
              }
            }
            n757 = call "IMAQ SetPixelLine"("Pixels Line (Float)"=w2192, "Line Coordinates"=w2193, "Image"=w2175) -> ()  [unwired: 7 in, 2 out]
            n758 = And(x=w2181, y=w2180) -> (x .and. y?=w2182:bool)
            n759 = case shown="True" w2182 {
              tunnel: w2192 -> [_ w2207]
              tunnel: w2191 -> [_ w2205]
              tunnel: w2174 -> [_ w2204]
              frame False {
              }
              frame True {
                n760 = Write to Binary File(file (use dialog)=w2204, data=w2207, 5:FALSE ("prepend array or string size? (T)"), 9:w2205) -> ()  [unwired: 2 in, 3 out]
              }
            }
          }
        }
      }
    }
    frame 22 {
      n761 = while {
        shift-right: [w2254] -> _
        shift-left: 0 -> [w2255]
        tunnel: w2233 -> [w2256]
        tunnel: w2232 -> [w2253]
        tunnel: w2231 -> [w2252]
        tunnel: w2230 -> [w2251]
        tunnel: w2219 -> [w2247]
        shift-right: [w2244] -> _
        shift-left: u32 0 -> [w2245]
        tunnel: w2228 -> [w2243]
        tunnel: w2227 -> [w2242]
        tunnel: w2226 -> [w2241]
        tunnel: w2225 -> [w2240]
        tunnel: w2220 -> [w2239]
        tunnel: w2224 -> [w2238]
        tunnel: w2223 -> [w2237]
        tunnel: w2222 -> [w2236]
        tunnel: w2221 -> [w2235]
        stop <- w2246 stop-if-true
        n762 = Get Queue Status(queue=w2240) -> (queue out=w2248:refnum<queue>, # elements in queue=w2250:i32)  [unwired: 2 in, 6 out]
        n763 = Get Notifier Status(notifier=w2247) -> (current notification=w2246:bool)  [unwired: 1 in, 4 out]
        n764 = Greater Than 0?(x=w2250) -> (x > 0?=w2249:bool)
        n765 = case shown="True" w2249 {
          tunnel: w2256 -> [_ w2285]
          tunnel: w2255 -> [w2258 w2286]
          tunnel: [w2258 w2284] -> w2254
          tunnel: w2253 -> [_ w2281]
          tunnel: w2252 -> [_ w2280]
          tunnel: w2251 -> [_ w2270]
          tunnel: w2248 -> [_ w2279]
          tunnel: w2245 -> [w2257 w2276]
          tunnel: [w2257 w2275] -> w2244
          tunnel: w2243 -> [_ w2274]
          tunnel: w2242 -> [_ w2273]
          tunnel: w2241 -> [_ w2268]
          tunnel: w2239 -> [_ w2266]
          tunnel: w2238 -> [_ w2264]
          tunnel: w2237 -> [_ _]
          tunnel: w2236 -> [_ _]
          tunnel: w2235 -> [_ _]
          frame False {
          }
          frame True {
            # "True: Last Frame of frame accum"
            # "Current Line in Frame Accum"
            # "Current Line In Frame"
            n766 = Increment(x=w2276) -> (x+1=w2269:u32)
            n767 = Dequeue Element(queue=w2279) -> (element=w2292:u64[])  [unwired: 2 in, 3 out]
            n768 = Equal?(x=w2269, y=w2273) -> (x = y?=w2278:bool)
            n769 = Greater?(x=w2269, y=w2274) -> (0:w2271:bool)
            n770 = Greater?(x=w2269, y=w2268) -> (0:w2267:bool)
            n771 = Split Number(x=w2292) -> (hi(x)=w2293:u32[], lo(x)=w2291:u32[])
            n772 = Split Number(x=w2293) -> (lo(x)=w2259:u16[])  [unwired: 1 out]
            n773 = Split Number(x=w2291) -> (hi(x)=w2260:u16[])  [unwired: 1 out]
            n774 = Select(t=u32 0, s=w2278, f=w2269) -> (s? t:f=w2275:u32)
            n775 = Increment(x=w2286) -> (x+1=w2288:i32)
            n776 = Equal?(x=w2285, y=w2286) -> (x = y?=w2287:bool)
            n777 = To Single Precision Float(number=w2259) -> (single precision float=w2263:sgl[])
            n778 = To Single Precision Float(number=w2260) -> (single precision float=w2262:sgl[])
            n779 = Select(t=0, s=w2287, f=w2288) -> (s? t:f=w2284:i32)
            n780 = Add(x=w2263, y=w2262) -> (x+y=w2261:sgl[])
            n781 = Build Array(0, w2286, w2285, w2286) -> (w2283:i32[])
            n782 = case shown="False" w2267 {
              tunnel: [w2301 w2307] -> w2282
              tunnel: w2283 -> [_ w2305]
              tunnel: w2280 -> [w2300 w2304]
              tunnel: w2266 -> [w2299 w2303]
              tunnel: [w2299 w2303] -> w2265
              tunnel: w2261 -> [w2298 w2302]
              frame False {
                n783 = Divide(x=w2298, y=w2300) -> (x/y=w2301:sgl[])
              }
              frame True {
                n784 = call "IMAQ GetPixelLine"("Line Coordinates"=w2305, "Image"=w2303) -> ("Pixels Line (Float)"=w2306:sgl[])  [unwired: 2 in, 4 out]
                n785 = Divide(x=w2302, y=w2304) -> (x/y=w2308:sgl[])
                n786 = Add(x=w2306, y=w2308) -> (x+y=w2307:sgl[])
              }
            }
            n787 = call "IMAQ SetPixelLine"("Pixels Line (Float)"=w2282, "Line Coordinates"=w2283, "Image"=w2265) -> ()  [unwired: 7 in, 2 out]
            n788 = And(x=w2271, y=w2270) -> (x .and. y?=w2272:bool)
            n789 = case shown="True" w2272 {
              tunnel: w2282 -> [_ w2297]
              tunnel: w2281 -> [_ w2295]
              tunnel: w2264 -> [_ w2294]
              frame False {
              }
              frame True {
                n790 = Write to Binary File(file (use dialog)=w2294, data=w2297, 5:FALSE ("prepend array or string size? (T)"), 9:w2295) -> ()  [unwired: 2 in, 3 out]
              }
            }
          }
        }
      }
    }
    frame 23 {
      n791 = while {
        shift-right: [w2344] -> _
        shift-left: 0 -> [w2345]
        tunnel: w2323 -> [w2346]
        tunnel: w2322 -> [w2343]
        tunnel: w2321 -> [w2342]
        tunnel: w2320 -> [w2341]
        tunnel: w2309 -> [w2337]
        shift-right: [w2334] -> _
        shift-left: u32 0 -> [w2335]
        tunnel: w2318 -> [w2333]
        tunnel: w2317 -> [w2332]
        tunnel: w2316 -> [w2331]
        tunnel: w2315 -> [w2330]
        tunnel: w2310 -> [w2329]
        tunnel: w2314 -> [w2328]
        tunnel: w2313 -> [w2327]
        tunnel: w2312 -> [w2326]
        tunnel: w2311 -> [w2325]
        stop <- w2336 stop-if-true
        n792 = Get Queue Status(queue=w2330) -> (queue out=w2338:refnum<queue>, # elements in queue=w2340:i32)  [unwired: 2 in, 6 out]
        n793 = Get Notifier Status(notifier=w2337) -> (current notification=w2336:bool)  [unwired: 1 in, 4 out]
        n794 = Greater Than 0?(x=w2340) -> (x > 0?=w2339:bool)
        n795 = case shown="True" w2339 {
          tunnel: w2346 -> [_ w2377]
          tunnel: w2345 -> [w2348 w2378]
          tunnel: [w2348 w2376] -> w2344
          tunnel: w2343 -> [_ w2373]
          tunnel: w2342 -> [_ w2372]
          tunnel: w2341 -> [_ w2362]
          tunnel: w2338 -> [_ w2371]
          tunnel: w2335 -> [w2347 w2368]
          tunnel: [w2347 w2367] -> w2334
          tunnel: w2333 -> [_ w2366]
          tunnel: w2332 -> [_ w2365]
          tunnel: w2331 -> [_ w2360]
          tunnel: w2329 -> [_ w2358]
          tunnel: w2328 -> [_ w2356]
          tunnel: w2327 -> [_ _]
          tunnel: w2326 -> [_ _]
          tunnel: w2325 -> [_ _]
          frame False {
          }
          frame True {
            # "True: Last Frame of frame accum"
            # "Current Line in Frame Accum"
            # "Current Line In Frame"
            n796 = Increment(x=w2368) -> (x+1=w2361:u32)
            n797 = Dequeue Element(queue=w2371) -> (element=w2384:u64[])  [unwired: 2 in, 3 out]
            n798 = Equal?(x=w2361, y=w2365) -> (x = y?=w2370:bool)
            n799 = Greater?(x=w2361, y=w2366) -> (0:w2363:bool)
            n800 = Greater?(x=w2361, y=w2360) -> (0:w2359:bool)
            n801 = Split Number(x=w2384) -> (hi(x)=w2385:u32[], lo(x)=w2383:u32[])
            n802 = Split Number(x=w2385) -> (hi(x)=w2354:u16[], lo(x)=w2353:u16[])
            n803 = Split Number(x=w2383) -> (hi(x)=w2355:u16[])  [unwired: 1 out]
            n804 = Select(t=u32 0, s=w2370, f=w2361) -> (s? t:f=w2367:u32)
            n805 = Increment(x=w2378) -> (x+1=w2380:i32)
            n806 = Equal?(x=w2377, y=w2378) -> (x = y?=w2379:bool)
            n807 = To Single Precision Float(number=w2354) -> (single precision float=w2352:sgl[])
            n808 = To Single Precision Float(number=w2353) -> (single precision float=w2350:sgl[])
            n809 = To Single Precision Float(number=w2355) -> (single precision float=w2351:sgl[])
            n810 = Select(t=0, s=w2379, f=w2380) -> (s? t:f=w2376:i32)
            n811 = Compound Arithmetic op=ADD(w2352, w2350, w2351) -> (w2349:sgl[])
            n812 = Build Array(0, w2378, w2377, w2378) -> (w2375:i32[])
            n813 = case shown="False" w2359 {
              tunnel: [w2393 w2399] -> w2374
              tunnel: w2375 -> [_ w2397]
              tunnel: w2372 -> [w2392 w2396]
              tunnel: w2358 -> [w2391 w2395]
              tunnel: [w2391 w2395] -> w2357
              tunnel: w2349 -> [w2390 w2394]
              frame False {
                n814 = Divide(x=w2390, y=w2392) -> (x/y=w2393:sgl[])
              }
              frame True {
                n815 = call "IMAQ GetPixelLine"("Line Coordinates"=w2397, "Image"=w2395) -> ("Pixels Line (Float)"=w2398:sgl[])  [unwired: 2 in, 4 out]
                n816 = Divide(x=w2394, y=w2396) -> (x/y=w2400:sgl[])
                n817 = Add(x=w2398, y=w2400) -> (x+y=w2399:sgl[])
              }
            }
            n818 = call "IMAQ SetPixelLine"("Pixels Line (Float)"=w2374, "Line Coordinates"=w2375, "Image"=w2357) -> ()  [unwired: 7 in, 2 out]
            n819 = And(x=w2363, y=w2362) -> (x .and. y?=w2364:bool)
            n820 = case shown="True" w2364 {
              tunnel: w2374 -> [_ w2389]
              tunnel: w2373 -> [_ w2387]
              tunnel: w2356 -> [_ w2386]
              frame False {
              }
              frame True {
                n821 = Write to Binary File(file (use dialog)=w2386, data=w2389, 5:FALSE ("prepend array or string size? (T)"), 9:w2387) -> ()  [unwired: 2 in, 3 out]
              }
            }
          }
        }
      }
    }
    frame 25 {
      n822 = while {
        shift-right: [w2436] -> _
        shift-left: 0 -> [w2437]
        tunnel: w2415 -> [w2438]
        tunnel: w2414 -> [w2435]
        tunnel: w2413 -> [w2434]
        tunnel: w2412 -> [w2433]
        tunnel: w2401 -> [w2429]
        shift-right: [w2426] -> _
        shift-left: u32 0 -> [w2427]
        tunnel: w2410 -> [w2425]
        tunnel: w2409 -> [w2424]
        tunnel: w2408 -> [w2423]
        tunnel: w2407 -> [w2422]
        tunnel: w2402 -> [w2421]
        tunnel: w2406 -> [w2420]
        tunnel: w2405 -> [w2419]
        tunnel: w2404 -> [w2418]
        tunnel: w2403 -> [w2417]
        stop <- w2428 stop-if-true
        n823 = Get Queue Status(queue=w2422) -> (queue out=w2430:refnum<queue>, # elements in queue=w2432:i32)  [unwired: 2 in, 6 out]
        n824 = Get Notifier Status(notifier=w2429) -> (current notification=w2428:bool)  [unwired: 1 in, 4 out]
        n825 = Greater Than 0?(x=w2432) -> (x > 0?=w2431:bool)
        n826 = case shown="True" w2431 {
          tunnel: w2438 -> [_ w2467]
          tunnel: w2437 -> [w2440 w2468]
          tunnel: [w2440 w2466] -> w2436
          tunnel: w2435 -> [_ w2463]
          tunnel: w2434 -> [_ w2462]
          tunnel: w2433 -> [_ w2452]
          tunnel: w2430 -> [_ w2461]
          tunnel: w2427 -> [w2439 w2458]
          tunnel: [w2439 w2457] -> w2426
          tunnel: w2425 -> [_ w2456]
          tunnel: w2424 -> [_ w2455]
          tunnel: w2423 -> [_ w2450]
          tunnel: w2421 -> [_ w2448]
          tunnel: w2420 -> [_ w2446]
          tunnel: w2419 -> [_ _]
          tunnel: w2418 -> [_ _]
          tunnel: w2417 -> [_ _]
          frame False {
          }
          frame True {
            # "True: Last Frame of frame accum"
            # "Current Line in Frame Accum"
            # "Current Line In Frame"
            n827 = Increment(x=w2458) -> (x+1=w2451:u32)
            n828 = Dequeue Element(queue=w2461) -> (element=w2474:u64[])  [unwired: 2 in, 3 out]
            n829 = Equal?(x=w2451, y=w2455) -> (x = y?=w2460:bool)
            n830 = Greater?(x=w2451, y=w2456) -> (0:w2453:bool)
            n831 = Greater?(x=w2451, y=w2450) -> (0:w2449:bool)
            n832 = Split Number(x=w2474) -> (hi(x)=w2475:u32[], lo(x)=w2473:u32[])
            n833 = Split Number(x=w2475) -> (hi(x)=w2441:u16[])  [unwired: 1 out]
            n834 = Split Number(x=w2473) -> (lo(x)=w2442:u16[])  [unwired: 1 out]
            n835 = Select(t=u32 0, s=w2460, f=w2451) -> (s? t:f=w2457:u32)
            n836 = Increment(x=w2468) -> (x+1=w2470:i32)
            n837 = Equal?(x=w2467, y=w2468) -> (x = y?=w2469:bool)
            n838 = To Single Precision Float(number=w2441) -> (single precision float=w2445:sgl[])
            n839 = To Single Precision Float(number=w2442) -> (single precision float=w2444:sgl[])
            n840 = Select(t=0, s=w2469, f=w2470) -> (s? t:f=w2466:i32)
            n841 = Add(x=w2445, y=w2444) -> (x+y=w2443:sgl[])
            n842 = Build Array(0, w2468, w2467, w2468) -> (w2465:i32[])
            n843 = case shown="False" w2449 {
              tunnel: [w2483 w2489] -> w2464
              tunnel: w2465 -> [_ w2487]
              tunnel: w2462 -> [w2482 w2486]
              tunnel: w2448 -> [w2481 w2485]
              tunnel: [w2481 w2485] -> w2447
              tunnel: w2443 -> [w2480 w2484]
              frame False {
                n844 = Divide(x=w2480, y=w2482) -> (x/y=w2483:sgl[])
              }
              frame True {
                n845 = call "IMAQ GetPixelLine"("Line Coordinates"=w2487, "Image"=w2485) -> ("Pixels Line (Float)"=w2488:sgl[])  [unwired: 2 in, 4 out]
                n846 = Divide(x=w2484, y=w2486) -> (x/y=w2490:sgl[])
                n847 = Add(x=w2488, y=w2490) -> (x+y=w2489:sgl[])
              }
            }
            n848 = call "IMAQ SetPixelLine"("Pixels Line (Float)"=w2464, "Line Coordinates"=w2465, "Image"=w2447) -> ()  [unwired: 7 in, 2 out]
            n849 = And(x=w2453, y=w2452) -> (x .and. y?=w2454:bool)
            n850 = case shown="True" w2454 {
              tunnel: w2464 -> [_ w2479]
              tunnel: w2463 -> [_ w2477]
              tunnel: w2446 -> [_ w2476]
              frame False {
              }
              frame True {
                n851 = Write to Binary File(file (use dialog)=w2476, data=w2479, 5:FALSE ("prepend array or string size? (T)"), 9:w2477) -> ()  [unwired: 2 in, 3 out]
              }
            }
          }
        }
      }
    }
    frame 26 {
      n852 = while {
        shift-right: [w2526] -> _
        shift-left: 0 -> [w2527]
        tunnel: w2505 -> [w2528]
        tunnel: w2504 -> [w2525]
        tunnel: w2503 -> [w2524]
        tunnel: w2502 -> [w2523]
        tunnel: w2491 -> [w2519]
        shift-right: [w2516] -> _
        shift-left: u32 0 -> [w2517]
        tunnel: w2500 -> [w2515]
        tunnel: w2499 -> [w2514]
        tunnel: w2498 -> [w2513]
        tunnel: w2497 -> [w2512]
        tunnel: w2492 -> [w2511]
        tunnel: w2496 -> [w2510]
        tunnel: w2495 -> [w2509]
        tunnel: w2494 -> [w2508]
        tunnel: w2493 -> [w2507]
        stop <- w2518 stop-if-true
        n853 = Get Queue Status(queue=w2512) -> (queue out=w2520:refnum<queue>, # elements in queue=w2522:i32)  [unwired: 2 in, 6 out]
        n854 = Get Notifier Status(notifier=w2519) -> (current notification=w2518:bool)  [unwired: 1 in, 4 out]
        n855 = Greater Than 0?(x=w2522) -> (x > 0?=w2521:bool)
        n856 = case shown="True" w2521 {
          tunnel: w2528 -> [_ w2557]
          tunnel: w2527 -> [w2530 w2558]
          tunnel: [w2530 w2556] -> w2526
          tunnel: w2525 -> [_ w2553]
          tunnel: w2524 -> [_ w2552]
          tunnel: w2523 -> [_ w2542]
          tunnel: w2520 -> [_ w2551]
          tunnel: w2517 -> [w2529 w2548]
          tunnel: [w2529 w2547] -> w2516
          tunnel: w2515 -> [_ w2546]
          tunnel: w2514 -> [_ w2545]
          tunnel: w2513 -> [_ w2540]
          tunnel: w2511 -> [_ w2538]
          tunnel: w2510 -> [_ w2536]
          tunnel: w2509 -> [_ _]
          tunnel: w2508 -> [_ _]
          tunnel: w2507 -> [_ _]
          frame False {
          }
          frame True {
            # "True: Last Frame of frame accum"
            # "Current Line in Frame Accum"
            # "Current Line In Frame"
            n857 = Increment(x=w2548) -> (x+1=w2541:u32)
            n858 = Dequeue Element(queue=w2551) -> (element=w2564:u64[])  [unwired: 2 in, 3 out]
            n859 = Equal?(x=w2541, y=w2545) -> (x = y?=w2550:bool)
            n860 = Greater?(x=w2541, y=w2546) -> (0:w2543:bool)
            n861 = Greater?(x=w2541, y=w2540) -> (0:w2539:bool)
            n862 = Split Number(x=w2564) -> (hi(x)=w2565:u32[], lo(x)=w2563:u32[])
            n863 = Split Number(x=w2565) -> (lo(x)=w2532:u16[])  [unwired: 1 out]
            n864 = Split Number(x=w2563) -> (lo(x)=w2531:u16[])  [unwired: 1 out]
            n865 = Select(t=u32 0, s=w2550, f=w2541) -> (s? t:f=w2547:u32)
            n866 = Increment(x=w2558) -> (x+1=w2560:i32)
            n867 = Equal?(x=w2557, y=w2558) -> (x = y?=w2559:bool)
            n868 = To Single Precision Float(number=w2532) -> (single precision float=w2535:sgl[])
            n869 = To Single Precision Float(number=w2531) -> (single precision float=w2534:sgl[])
            n870 = Select(t=0, s=w2559, f=w2560) -> (s? t:f=w2556:i32)
            n871 = Add(x=w2535, y=w2534) -> (x+y=w2533:sgl[])
            n872 = Build Array(0, w2558, w2557, w2558) -> (w2555:i32[])
            n873 = case shown="False" w2539 {
              tunnel: [w2573 w2579] -> w2554
              tunnel: w2555 -> [_ w2577]
              tunnel: w2552 -> [w2572 w2576]
              tunnel: w2538 -> [w2571 w2575]
              tunnel: [w2571 w2575] -> w2537
              tunnel: w2533 -> [w2570 w2574]
              frame False {
                n874 = Divide(x=w2570, y=w2572) -> (x/y=w2573:sgl[])
              }
              frame True {
                n875 = call "IMAQ GetPixelLine"("Line Coordinates"=w2577, "Image"=w2575) -> ("Pixels Line (Float)"=w2578:sgl[])  [unwired: 2 in, 4 out]
                n876 = Divide(x=w2574, y=w2576) -> (x/y=w2580:sgl[])
                n877 = Add(x=w2578, y=w2580) -> (x+y=w2579:sgl[])
              }
            }
            n878 = call "IMAQ SetPixelLine"("Pixels Line (Float)"=w2554, "Line Coordinates"=w2555, "Image"=w2537) -> ()  [unwired: 7 in, 2 out]
            n879 = And(x=w2543, y=w2542) -> (x .and. y?=w2544:bool)
            n880 = case shown="True" w2544 {
              tunnel: w2554 -> [_ w2569]
              tunnel: w2553 -> [_ w2567]
              tunnel: w2536 -> [_ w2566]
              frame False {
              }
              frame True {
                n881 = Write to Binary File(file (use dialog)=w2566, data=w2569, 5:FALSE ("prepend array or string size? (T)"), 9:w2567) -> ()  [unwired: 2 in, 3 out]
              }
            }
          }
        }
      }
    }
    frame 27 {
      n882 = while {
        shift-right: [w2616] -> _
        shift-left: 0 -> [w2617]
        tunnel: w2595 -> [w2618]
        tunnel: w2594 -> [w2615]
        tunnel: w2593 -> [w2614]
        tunnel: w2592 -> [w2613]
        tunnel: w2581 -> [w2609]
        shift-right: [w2606] -> _
        shift-left: u32 0 -> [w2607]
        tunnel: w2590 -> [w2605]
        tunnel: w2589 -> [w2604]
        tunnel: w2588 -> [w2603]
        tunnel: w2587 -> [w2602]
        tunnel: w2582 -> [w2601]
        tunnel: w2586 -> [w2600]
        tunnel: w2585 -> [w2599]
        tunnel: w2584 -> [w2598]
        tunnel: w2583 -> [w2597]
        stop <- w2608 stop-if-true
        n883 = Get Queue Status(queue=w2602) -> (queue out=w2610:refnum<queue>, # elements in queue=w2612:i32)  [unwired: 2 in, 6 out]
        n884 = Get Notifier Status(notifier=w2609) -> (current notification=w2608:bool)  [unwired: 1 in, 4 out]
        n885 = Greater Than 0?(x=w2612) -> (x > 0?=w2611:bool)
        n886 = case shown="True" w2611 {
          tunnel: w2618 -> [_ w2649]
          tunnel: w2617 -> [w2620 w2650]
          tunnel: [w2620 w2648] -> w2616
          tunnel: w2615 -> [_ w2645]
          tunnel: w2614 -> [_ w2644]
          tunnel: w2613 -> [_ w2634]
          tunnel: w2610 -> [_ w2643]
          tunnel: w2607 -> [w2619 w2640]
          tunnel: [w2619 w2639] -> w2606
          tunnel: w2605 -> [_ w2638]
          tunnel: w2604 -> [_ w2637]
          tunnel: w2603 -> [_ w2632]
          tunnel: w2601 -> [_ w2630]
          tunnel: w2600 -> [_ w2628]
          tunnel: w2599 -> [_ _]
          tunnel: w2598 -> [_ _]
          tunnel: w2597 -> [_ _]
          frame False {
          }
          frame True {
            # "True: Last Frame of frame accum"
            # "Current Line in Frame Accum"
            # "Current Line In Frame"
            n887 = Increment(x=w2640) -> (x+1=w2633:u32)
            n888 = Dequeue Element(queue=w2643) -> (element=w2656:u64[])  [unwired: 2 in, 3 out]
            n889 = Equal?(x=w2633, y=w2637) -> (x = y?=w2642:bool)
            n890 = Greater?(x=w2633, y=w2638) -> (0:w2635:bool)
            n891 = Greater?(x=w2633, y=w2632) -> (0:w2631:bool)
            n892 = Split Number(x=w2656) -> (hi(x)=w2657:u32[], lo(x)=w2655:u32[])
            n893 = Split Number(x=w2657) -> (hi(x)=w2627:u16[], lo(x)=w2626:u16[])
            n894 = Split Number(x=w2655) -> (lo(x)=w2621:u16[])  [unwired: 1 out]
            n895 = Select(t=u32 0, s=w2642, f=w2633) -> (s? t:f=w2639:u32)
            n896 = Increment(x=w2650) -> (x+1=w2652:i32)
            n897 = Equal?(x=w2649, y=w2650) -> (x = y?=w2651:bool)
            n898 = To Single Precision Float(number=w2627) -> (single precision float=w2625:sgl[])
            n899 = To Single Precision Float(number=w2626) -> (single precision float=w2623:sgl[])
            n900 = To Single Precision Float(number=w2621) -> (single precision float=w2624:sgl[])
            n901 = Select(t=0, s=w2651, f=w2652) -> (s? t:f=w2648:i32)
            n902 = Compound Arithmetic op=ADD(w2625, w2623, w2624) -> (w2622:sgl[])
            n903 = Build Array(0, w2650, w2649, w2650) -> (w2647:i32[])
            n904 = case shown="False" w2631 {
              tunnel: [w2665 w2671] -> w2646
              tunnel: w2647 -> [_ w2669]
              tunnel: w2644 -> [w2664 w2668]
              tunnel: w2630 -> [w2663 w2667]
              tunnel: [w2663 w2667] -> w2629
              tunnel: w2622 -> [w2662 w2666]
              frame False {
                n905 = Divide(x=w2662, y=w2664) -> (x/y=w2665:sgl[])
              }
              frame True {
                n906 = call "IMAQ GetPixelLine"("Line Coordinates"=w2669, "Image"=w2667) -> ("Pixels Line (Float)"=w2670:sgl[])  [unwired: 2 in, 4 out]
                n907 = Divide(x=w2666, y=w2668) -> (x/y=w2672:sgl[])
                n908 = Add(x=w2670, y=w2672) -> (x+y=w2671:sgl[])
              }
            }
            n909 = call "IMAQ SetPixelLine"("Pixels Line (Float)"=w2646, "Line Coordinates"=w2647, "Image"=w2629) -> ()  [unwired: 7 in, 2 out]
            n910 = And(x=w2635, y=w2634) -> (x .and. y?=w2636:bool)
            n911 = case shown="True" w2636 {
              tunnel: w2646 -> [_ w2661]
              tunnel: w2645 -> [_ w2659]
              tunnel: w2628 -> [_ w2658]
              frame False {
              }
              frame True {
                n912 = Write to Binary File(file (use dialog)=w2658, data=w2661, 5:FALSE ("prepend array or string size? (T)"), 9:w2659) -> ()  [unwired: 2 in, 3 out]
              }
            }
          }
        }
      }
    }
    frame 28 {
      n913 = while {
        shift-right: [w2708] -> _
        shift-left: 0 -> [w2709]
        tunnel: w2687 -> [w2710]
        tunnel: w2686 -> [w2707]
        tunnel: w2685 -> [w2706]
        tunnel: w2684 -> [w2705]
        tunnel: w2673 -> [w2701]
        shift-right: [w2698] -> _
        shift-left: u32 0 -> [w2699]
        tunnel: w2682 -> [w2697]
        tunnel: w2681 -> [w2696]
        tunnel: w2680 -> [w2695]
        tunnel: w2679 -> [w2694]
        tunnel: w2674 -> [w2693]
        tunnel: w2678 -> [w2692]
        tunnel: w2677 -> [w2691]
        tunnel: w2676 -> [w2690]
        tunnel: w2675 -> [w2689]
        stop <- w2700 stop-if-true
        n914 = Get Queue Status(queue=w2694) -> (queue out=w2702:refnum<queue>, # elements in queue=w2704:i32)  [unwired: 2 in, 6 out]
        n915 = Get Notifier Status(notifier=w2701) -> (current notification=w2700:bool)  [unwired: 1 in, 4 out]
        n916 = Greater Than 0?(x=w2704) -> (x > 0?=w2703:bool)
        n917 = case shown="True" w2703 {
          tunnel: w2710 -> [_ w2739]
          tunnel: w2709 -> [w2712 w2740]
          tunnel: [w2712 w2738] -> w2708
          tunnel: w2707 -> [_ w2735]
          tunnel: w2706 -> [_ w2734]
          tunnel: w2705 -> [_ w2724]
          tunnel: w2702 -> [_ w2733]
          tunnel: w2699 -> [w2711 w2730]
          tunnel: [w2711 w2729] -> w2698
          tunnel: w2697 -> [_ w2728]
          tunnel: w2696 -> [_ w2727]
          tunnel: w2695 -> [_ w2722]
          tunnel: w2693 -> [_ w2720]
          tunnel: w2692 -> [_ w2718]
          tunnel: w2691 -> [_ _]
          tunnel: w2690 -> [_ _]
          tunnel: w2689 -> [_ _]
          frame False {
          }
          frame True {
            # "True: Last Frame of frame accum"
            # "Current Line in Frame Accum"
            # "Current Line In Frame"
            n918 = Increment(x=w2730) -> (x+1=w2723:u32)
            n919 = Dequeue Element(queue=w2733) -> (element=w2746:u64[])  [unwired: 2 in, 3 out]
            n920 = Equal?(x=w2723, y=w2727) -> (x = y?=w2732:bool)
            n921 = Greater?(x=w2723, y=w2728) -> (0:w2725:bool)
            n922 = Greater?(x=w2723, y=w2722) -> (0:w2721:bool)
            n923 = Split Number(x=w2746) -> (lo(x)=w2745:u32[])  [unwired: 1 out]
            n924 = Split Number(x=w2745) -> (hi(x)=w2713:u16[], lo(x)=w2714:u16[])
            n925 = Select(t=u32 0, s=w2732, f=w2723) -> (s? t:f=w2729:u32)
            n926 = Increment(x=w2740) -> (x+1=w2742:i32)
            n927 = Equal?(x=w2739, y=w2740) -> (x = y?=w2741:bool)
            n928 = To Single Precision Float(number=w2713) -> (single precision float=w2717:sgl[])
            n929 = To Single Precision Float(number=w2714) -> (single precision float=w2716:sgl[])
            n930 = Select(t=0, s=w2741, f=w2742) -> (s? t:f=w2738:i32)
            n931 = Add(x=w2717, y=w2716) -> (x+y=w2715:sgl[])
            n932 = Build Array(0, w2740, w2739, w2740) -> (w2737:i32[])
            n933 = case shown="False" w2721 {
              tunnel: [w2754 w2760] -> w2736
              tunnel: w2737 -> [_ w2758]
              tunnel: w2734 -> [w2753 w2757]
              tunnel: w2720 -> [w2752 w2756]
              tunnel: [w2752 w2756] -> w2719
              tunnel: w2715 -> [w2751 w2755]
              frame False {
                n934 = Divide(x=w2751, y=w2753) -> (x/y=w2754:sgl[])
              }
              frame True {
                n935 = call "IMAQ GetPixelLine"("Line Coordinates"=w2758, "Image"=w2756) -> ("Pixels Line (Float)"=w2759:sgl[])  [unwired: 2 in, 4 out]
                n936 = Divide(x=w2755, y=w2757) -> (x/y=w2761:sgl[])
                n937 = Add(x=w2759, y=w2761) -> (x+y=w2760:sgl[])
              }
            }
            n938 = call "IMAQ SetPixelLine"("Pixels Line (Float)"=w2736, "Line Coordinates"=w2737, "Image"=w2719) -> ()  [unwired: 7 in, 2 out]
            n939 = And(x=w2725, y=w2724) -> (x .and. y?=w2726:bool)
            n940 = case shown="True" w2726 {
              tunnel: w2736 -> [_ w2750]
              tunnel: w2735 -> [_ w2748]
              tunnel: w2718 -> [_ w2747]
              frame False {
              }
              frame True {
                n941 = Write to Binary File(file (use dialog)=w2747, data=w2750, 5:FALSE ("prepend array or string size? (T)"), 9:w2748) -> ()  [unwired: 2 in, 3 out]
              }
            }
          }
        }
      }
    }
    frame 29 {
      n942 = while {
        shift-right: [w2797] -> _
        shift-left: 0 -> [w2798]
        tunnel: w2776 -> [w2799]
        tunnel: w2775 -> [w2796]
        tunnel: w2774 -> [w2795]
        tunnel: w2773 -> [w2794]
        tunnel: w2762 -> [w2790]
        shift-right: [w2787] -> _
        shift-left: u32 0 -> [w2788]
        tunnel: w2771 -> [w2786]
        tunnel: w2770 -> [w2785]
        tunnel: w2769 -> [w2784]
        tunnel: w2768 -> [w2783]
        tunnel: w2763 -> [w2782]
        tunnel: w2767 -> [w2781]
        tunnel: w2766 -> [w2780]
        tunnel: w2765 -> [w2779]
        tunnel: w2764 -> [w2778]
        stop <- w2789 stop-if-true
        n943 = Get Queue Status(queue=w2783) -> (queue out=w2791:refnum<queue>, # elements in queue=w2793:i32)  [unwired: 2 in, 6 out]
        n944 = Get Notifier Status(notifier=w2790) -> (current notification=w2789:bool)  [unwired: 1 in, 4 out]
        n945 = Greater Than 0?(x=w2793) -> (x > 0?=w2792:bool)
        n946 = case shown="True" w2792 {
          tunnel: w2799 -> [_ w2830]
          tunnel: w2798 -> [w2801 w2831]
          tunnel: [w2801 w2829] -> w2797
          tunnel: w2796 -> [_ w2826]
          tunnel: w2795 -> [_ w2825]
          tunnel: w2794 -> [_ w2815]
          tunnel: w2791 -> [_ w2824]
          tunnel: w2788 -> [w2800 w2821]
          tunnel: [w2800 w2820] -> w2787
          tunnel: w2786 -> [_ w2819]
          tunnel: w2785 -> [_ w2818]
          tunnel: w2784 -> [_ w2813]
          tunnel: w2782 -> [_ w2811]
          tunnel: w2781 -> [_ w2809]
          tunnel: w2780 -> [_ _]
          tunnel: w2779 -> [_ _]
          tunnel: w2778 -> [_ _]
          frame False {
          }
          frame True {
            # "True: Last Frame of frame accum"
            # "Current Line in Frame Accum"
            # "Current Line In Frame"
            n947 = Increment(x=w2821) -> (x+1=w2814:u32)
            n948 = Dequeue Element(queue=w2824) -> (element=w2837:u64[])  [unwired: 2 in, 3 out]
            n949 = Equal?(x=w2814, y=w2818) -> (x = y?=w2823:bool)
            n950 = Greater?(x=w2814, y=w2819) -> (0:w2816:bool)
            n951 = Greater?(x=w2814, y=w2813) -> (0:w2812:bool)
            n952 = Split Number(x=w2837) -> (hi(x)=w2838:u32[], lo(x)=w2836:u32[])
            n953 = Split Number(x=w2838) -> (hi(x)=w2808:u16[])  [unwired: 1 out]
            n954 = Split Number(x=w2836) -> (hi(x)=w2803:u16[], lo(x)=w2802:u16[])
            n955 = Select(t=u32 0, s=w2823, f=w2814) -> (s? t:f=w2820:u32)
            n956 = Increment(x=w2831) -> (x+1=w2833:i32)
            n957 = Equal?(x=w2830, y=w2831) -> (x = y?=w2832:bool)
            n958 = To Single Precision Float(number=w2808) -> (single precision float=w2807:sgl[])
            n959 = To Single Precision Float(number=w2803) -> (single precision float=w2805:sgl[])
            n960 = To Single Precision Float(number=w2802) -> (single precision float=w2806:sgl[])
            n961 = Select(t=0, s=w2832, f=w2833) -> (s? t:f=w2829:i32)
            n962 = Compound Arithmetic op=ADD(w2807, w2805, w2806) -> (w2804:sgl[])
            n963 = Build Array(0, w2831, w2830, w2831) -> (w2828:i32[])
            n964 = case shown="False" w2812 {
              tunnel: [w2846 w2852] -> w2827
              tunnel: w2828 -> [_ w2850]
              tunnel: w2825 -> [w2845 w2849]
              tunnel: w2811 -> [w2844 w2848]
              tunnel: [w2844 w2848] -> w2810
              tunnel: w2804 -> [w2843 w2847]
              frame False {
                n965 = Divide(x=w2843, y=w2845) -> (x/y=w2846:sgl[])
              }
              frame True {
                n966 = call "IMAQ GetPixelLine"("Line Coordinates"=w2850, "Image"=w2848) -> ("Pixels Line (Float)"=w2851:sgl[])  [unwired: 2 in, 4 out]
                n967 = Divide(x=w2847, y=w2849) -> (x/y=w2853:sgl[])
                n968 = Add(x=w2851, y=w2853) -> (x+y=w2852:sgl[])
              }
            }
            n969 = call "IMAQ SetPixelLine"("Pixels Line (Float)"=w2827, "Line Coordinates"=w2828, "Image"=w2810) -> ()  [unwired: 7 in, 2 out]
            n970 = And(x=w2816, y=w2815) -> (x .and. y?=w2817:bool)
            n971 = case shown="True" w2817 {
              tunnel: w2827 -> [_ w2842]
              tunnel: w2826 -> [_ w2840]
              tunnel: w2809 -> [_ w2839]
              frame False {
              }
              frame True {
                n972 = Write to Binary File(file (use dialog)=w2839, data=w2842, 5:FALSE ("prepend array or string size? (T)"), 9:w2840) -> ()  [unwired: 2 in, 3 out]
              }
            }
          }
        }
      }
    }
    frame 30 {
      n973 = while {
        shift-right: [w2889] -> _
        shift-left: 0 -> [w2890]
        tunnel: w2868 -> [w2891]
        tunnel: w2867 -> [w2888]
        tunnel: w2866 -> [w2887]
        tunnel: w2865 -> [w2886]
        tunnel: w2854 -> [w2882]
        shift-right: [w2879] -> _
        shift-left: u32 0 -> [w2880]
        tunnel: w2863 -> [w2878]
        tunnel: w2862 -> [w2877]
        tunnel: w2861 -> [w2876]
        tunnel: w2860 -> [w2875]
        tunnel: w2855 -> [w2874]
        tunnel: w2859 -> [w2873]
        tunnel: w2858 -> [w2872]
        tunnel: w2857 -> [w2871]
        tunnel: w2856 -> [w2870]
        stop <- w2881 stop-if-true
        n974 = Get Queue Status(queue=w2875) -> (queue out=w2883:refnum<queue>, # elements in queue=w2885:i32)  [unwired: 2 in, 6 out]
        n975 = Get Notifier Status(notifier=w2882) -> (current notification=w2881:bool)  [unwired: 1 in, 4 out]
        n976 = Greater Than 0?(x=w2885) -> (x > 0?=w2884:bool)
        n977 = case shown="True" w2884 {
          tunnel: w2891 -> [_ w2922]
          tunnel: w2890 -> [w2893 w2923]
          tunnel: [w2893 w2921] -> w2889
          tunnel: w2888 -> [_ w2918]
          tunnel: w2887 -> [_ w2917]
          tunnel: w2886 -> [_ w2907]
          tunnel: w2883 -> [_ w2916]
          tunnel: w2880 -> [w2892 w2913]
          tunnel: [w2892 w2912] -> w2879
          tunnel: w2878 -> [_ w2911]
          tunnel: w2877 -> [_ w2910]
          tunnel: w2876 -> [_ w2905]
          tunnel: w2874 -> [_ w2903]
          tunnel: w2873 -> [_ w2901]
          tunnel: w2872 -> [_ _]
          tunnel: w2871 -> [_ _]
          tunnel: w2870 -> [_ _]
          frame False {
          }
          frame True {
            # "True: Last Frame of frame accum"
            # "Current Line in Frame Accum"
            # "Current Line In Frame"
            n978 = Increment(x=w2913) -> (x+1=w2906:u32)
            n979 = Dequeue Element(queue=w2916) -> (element=w2929:u64[])  [unwired: 2 in, 3 out]
            n980 = Equal?(x=w2906, y=w2910) -> (x = y?=w2915:bool)
            n981 = Greater?(x=w2906, y=w2911) -> (0:w2908:bool)
            n982 = Greater?(x=w2906, y=w2905) -> (0:w2904:bool)
            n983 = Split Number(x=w2929) -> (hi(x)=w2930:u32[], lo(x)=w2928:u32[])
            n984 = Split Number(x=w2930) -> (lo(x)=w2894:u16[])  [unwired: 1 out]
            n985 = Split Number(x=w2928) -> (hi(x)=w2896:u16[], lo(x)=w2895:u16[])
            n986 = Select(t=u32 0, s=w2915, f=w2906) -> (s? t:f=w2912:u32)
            n987 = Increment(x=w2923) -> (x+1=w2925:i32)
            n988 = Equal?(x=w2922, y=w2923) -> (x = y?=w2924:bool)
            n989 = To Single Precision Float(number=w2894) -> (single precision float=w2900:sgl[])
            n990 = To Single Precision Float(number=w2896) -> (single precision float=w2898:sgl[])
            n991 = To Single Precision Float(number=w2895) -> (single precision float=w2899:sgl[])
            n992 = Select(t=0, s=w2924, f=w2925) -> (s? t:f=w2921:i32)
            n993 = Compound Arithmetic op=ADD(w2900, w2898, w2899) -> (w2897:sgl[])
            n994 = Build Array(0, w2923, w2922, w2923) -> (w2920:i32[])
            n995 = case shown="False" w2904 {
              tunnel: [w2938 w2944] -> w2919
              tunnel: w2920 -> [_ w2942]
              tunnel: w2917 -> [w2937 w2941]
              tunnel: w2903 -> [w2936 w2940]
              tunnel: [w2936 w2940] -> w2902
              tunnel: w2897 -> [w2935 w2939]
              frame False {
                n996 = Divide(x=w2935, y=w2937) -> (x/y=w2938:sgl[])
              }
              frame True {
                n997 = call "IMAQ GetPixelLine"("Line Coordinates"=w2942, "Image"=w2940) -> ("Pixels Line (Float)"=w2943:sgl[])  [unwired: 2 in, 4 out]
                n998 = Divide(x=w2939, y=w2941) -> (x/y=w2945:sgl[])
                n999 = Add(x=w2943, y=w2945) -> (x+y=w2944:sgl[])
              }
            }
            n1000 = call "IMAQ SetPixelLine"("Pixels Line (Float)"=w2919, "Line Coordinates"=w2920, "Image"=w2902) -> ()  [unwired: 7 in, 2 out]
            n1001 = And(x=w2908, y=w2907) -> (x .and. y?=w2909:bool)
            n1002 = case shown="True" w2909 {
              tunnel: w2919 -> [_ w2934]
              tunnel: w2918 -> [_ w2932]
              tunnel: w2901 -> [_ w2931]
              frame False {
              }
              frame True {
                n1003 = Write to Binary File(file (use dialog)=w2931, data=w2934, 5:FALSE ("prepend array or string size? (T)"), 9:w2932) -> ()  [unwired: 2 in, 3 out]
              }
            }
          }
        }
      }
    }
    frame 31 {
      n1004 = while {
        shift-right: [w2981] -> _
        shift-left: 0 -> [w2982]
        tunnel: w2960 -> [w2983]
        tunnel: w2959 -> [w2980]
        tunnel: w2958 -> [w2979]
        tunnel: w2957 -> [w2978]
        tunnel: w2946 -> [w2974]
        shift-right: [w2971] -> _
        shift-left: u32 0 -> [w2972]
        tunnel: w2955 -> [w2970]
        tunnel: w2954 -> [w2969]
        tunnel: w2953 -> [w2968]
        tunnel: w2952 -> [w2967]
        tunnel: w2947 -> [w2966]
        tunnel: w2951 -> [w2965]
        tunnel: w2950 -> [w2964]
        tunnel: w2949 -> [w2963]
        tunnel: w2948 -> [w2962]
        stop <- w2973 stop-if-true
        n1005 = Get Queue Status(queue=w2967) -> (queue out=w2975:refnum<queue>, # elements in queue=w2977:i32)  [unwired: 2 in, 6 out]
        n1006 = Get Notifier Status(notifier=w2974) -> (current notification=w2973:bool)  [unwired: 1 in, 4 out]
        n1007 = Greater Than 0?(x=w2977) -> (x > 0?=w2976:bool)
        n1008 = case shown="True" w2976 {
          tunnel: w2983 -> [_ w3016]
          tunnel: w2982 -> [w2985 w3017]
          tunnel: [w2985 w3015] -> w2981
          tunnel: w2980 -> [_ w3012]
          tunnel: w2979 -> [_ w3011]
          tunnel: w2978 -> [_ w3001]
          tunnel: w2975 -> [_ w3010]
          tunnel: w2972 -> [w2984 w3007]
          tunnel: [w2984 w3006] -> w2971
          tunnel: w2970 -> [_ w3005]
          tunnel: w2969 -> [_ w3004]
          tunnel: w2968 -> [_ w2999]
          tunnel: w2966 -> [_ w2997]
          tunnel: w2965 -> [_ w2995]
          tunnel: w2964 -> [_ _]
          tunnel: w2963 -> [_ _]
          tunnel: w2962 -> [_ _]
          frame False {
          }
          frame True {
            # "True: Last Frame of frame accum"
            # "Current Line in Frame Accum"
            # "Current Line In Frame"
            n1009 = Increment(x=w3007) -> (x+1=w3000:u32)
            n1010 = Dequeue Element(queue=w3010) -> (element=w3023:u64[])  [unwired: 2 in, 3 out]
            n1011 = Equal?(x=w3000, y=w3004) -> (x = y?=w3009:bool)
            n1012 = Greater?(x=w3000, y=w3005) -> (0:w3002:bool)
            n1013 = Greater?(x=w3000, y=w2999) -> (0:w2998:bool)
            n1014 = Split Number(x=w3023) -> (hi(x)=w3024:u32[], lo(x)=w3022:u32[])
            n1015 = Split Number(x=w3024) -> (hi(x)=w2989:u16[], lo(x)=w2988:u16[])
            n1016 = Split Number(x=w3022) -> (hi(x)=w2987:u16[], lo(x)=w2986:u16[])
            n1017 = Select(t=u32 0, s=w3009, f=w3000) -> (s? t:f=w3006:u32)
            n1018 = Increment(x=w3017) -> (x+1=w3019:i32)
            n1019 = Equal?(x=w3016, y=w3017) -> (x = y?=w3018:bool)
            n1020 = To Single Precision Float(number=w2989) -> (single precision float=w2994:sgl[])
            n1021 = To Single Precision Float(number=w2988) -> (single precision float=w2992:sgl[])
            n1022 = To Single Precision Float(number=w2987) -> (single precision float=w2993:sgl[])
            n1023 = To Single Precision Float(number=w2986) -> (single precision float=w2990:sgl[])
            n1024 = Select(t=0, s=w3018, f=w3019) -> (s? t:f=w3015:i32)
            n1025 = Compound Arithmetic op=ADD(w2994, w2992, w2993, w2990) -> (w2991:sgl[])
            n1026 = Build Array(0, w3017, w3016, w3017) -> (w3014:i32[])
            n1027 = case shown="False" w2998 {
              tunnel: [w3032 w3038] -> w3013
              tunnel: w3014 -> [_ w3036]
              tunnel: w3011 -> [w3031 w3035]
              tunnel: w2997 -> [w3030 w3034]
              tunnel: [w3030 w3034] -> w2996
              tunnel: w2991 -> [w3029 w3033]
              frame False {
                n1028 = Divide(x=w3029, y=w3031) -> (x/y=w3032:sgl[])
              }
              frame True {
                n1029 = call "IMAQ GetPixelLine"("Line Coordinates"=w3036, "Image"=w3034) -> ("Pixels Line (Float)"=w3037:sgl[])  [unwired: 2 in, 4 out]
                n1030 = Divide(x=w3033, y=w3035) -> (x/y=w3039:sgl[])
                n1031 = Add(x=w3037, y=w3039) -> (x+y=w3038:sgl[])
              }
            }
            n1032 = call "IMAQ SetPixelLine"("Pixels Line (Float)"=w3013, "Line Coordinates"=w3014, "Image"=w2996) -> ()  [unwired: 7 in, 2 out]
            n1033 = And(x=w3002, y=w3001) -> (x .and. y?=w3003:bool)
            n1034 = case shown="True" w3003 {
              tunnel: w3013 -> [_ w3028]
              tunnel: w3012 -> [_ w3026]
              tunnel: w2995 -> [_ w3025]
              frame False {
              }
              frame True {
                n1035 = Write to Binary File(file (use dialog)=w3025, data=w3028, 5:FALSE ("prepend array or string size? (T)"), 9:w3026) -> ()  [unwired: 2 in, 3 out]
              }
            }
          }
        }
      }
    }
  }
  n1036 = Flush Queue(queue=w28) -> (queue out=w70:refnum<queue>)  [unwired: 1 in, 2 out]
  n1037 = Release Queue(queue=w70) -> ()  [unwired: 2 in, 3 out]
  n1038 = while {
    tunnel: w83 -> [w3060]
    shift-right: [w3042] -> _
    shift-left: u32 0 -> [w3041]
    tunnel: w109 -> [w3040]
    shift-right: [w3056] -> _
    shift-left: FALSE -> [w3055]
    tunnel: w29 -> [w3054]
    shift-right: [w3052] -> _
    shift-left: u32 0 -> [w3053]
    tunnel: w104 -> [w3048]
    tunnel: w25 -> [w3045]
    tunnel: [w3043] -> w84
    shift-right: [w3044] -> w98
    shift-left: w14 -> [w3061]
    stop <- w3051 stop-if-true
    # "Total Lines Counter"
    n1039 = xnode "Invoke Method"("FPGA VI Reference In"=w3060, "Number of Elements"=w3041, "Timeout (ms)"=0) -> ("FPGA VI Reference Out"=w3043:refnum<k20>, "Data"=w3049:u64[], "Elements Remaining"=w3058:u32)  [unwired: 1 in, 1 out]
    n1040 = Get Notifier Status(notifier=w3061) -> (notifier out=w3044:refnum<notifier>, current notification=w3050:bool)  [unwired: 1 in, 3 out]
    n1041 = case shown="False" w3055 {
      tunnel: w3049 -> [_ w3064]
      tunnel: w3054 -> [_ w3070]
      tunnel: w3053 -> [w3063 w3067]
      tunnel: [w3063 w3068] -> w3052
      tunnel: [w3062 w3066] -> w3047
      tunnel: w3050 -> [w3062 _]
      tunnel: w3048 -> [_ w3065]
      frame False {
      }
      frame True {
        n1042 = Increment(x=w3067) -> (x+1=w3068:u32)
        n1043 = Enqueue Element(queue=w3070, element=w3064, timeout in ms (-1)=0) -> ()  [unwired: 1 in, 3 out]
        n1044 = Equal?(x=w3068, y=w3065) -> (x = y?=w3066:bool)
      }
    }
    n1045 = Greater Or Equal?(x=w3058, y=w3040) -> (x >= y?=w3056:bool)
    n1046 = Select(t=w3040, s=w3056, f=u32 0) -> (s? t:f=w3042:u32)
    n1047 = And(x=w3045, y=w3047) -> (x .and. y?=w3046:bool)
    n1048 = Or(x=w3046, y=w3050) -> (x .or. y?=w3051:bool)
  }
  n1049 = xnode "Close FPGA VI Reference"("FPGA VI Reference In"=w84) -> ()  [unwired: 1 in, 1 out]
  n1050 = Send Notification(notification=TRUE, notifier=w98) -> ()  [unwired: 1 in, 2 out]
